vi "Text control 2 v7.3_pump-specific.vi"() -> ()   [LabVIEW 2019]
panel:
  in  "Tab Control":enum32{"Main", "Other parameters"}(tab)
  out "Vdg vs time (Bias Stress)":cluster{"Y data in":dbl[], "X data in":dbl[]}[](graph)
  out "Vp vs Vg (FPP)":cluster{"Y data in":dbl[], "X data in":dbl[]}[](graph)
  out "Vp vs time (FPP Bias Stress)":cluster{"Y data in":dbl[], "X data in":dbl[]}[](graph)
  out "Line running":i32
  out "Total lines":i32
  out "Path":path=path "C:/users/rlp38/09Apr2009LTtesting/test2.txt"
  out "I vs Vg":cluster{"Y data in":dbl[], "X data in":dbl[]}[](graph)
  out "Is max":dbl format="%.2e"
  out "Id max":dbl format="%.2e"
  out "Ig max":dbl format="%.2e"
  out "Imax vs time":cluster{"Y data in":dbl[], "X data in":dbl[]}[](graph)
  out "Imin vs time":cluster{"Y data in":dbl[], "X data in":dbl[]}[](graph)
  out "I vs Vd":cluster{"Y data in":dbl[], "X data in":dbl[]}[](graph)
  in  "Script":string
  out "Command running:":string
  out "Serial port data":string
  out "Elapsed Time":dbl caption="Elapsed Time (s)"
  in  "Time Units":u16(ring)=1 items=["Seconds", "Minutes", "Hours"]
  in  "Time Offset":dbl caption="Set Start Time (s)"
  in  "Reset":bool
  in  "Auto Reset":bool
  in  "integration time":u32(slide) max=2 step=1 scale=0.0..2.0
  in  "Interrupt scan":bool
  out "Absolute plunger position vs time":cluster{"Y data in":dbl[], "X data in":dbl[]}[](graph)
  out "Valve position vs time":cluster{"Y data in":dbl[], "X data in":dbl[]}[](graph)
  out "Is on":dbl format="%.2e"
  out "Id on":dbl format="%.2e"
  out "Ig on":dbl format="%.2e"
  out "Ion vs time":cluster{"Y data in":dbl[], "X data in":dbl[]}[](graph)
  out "Ioff vs time":cluster{"Y data in":dbl[], "X data in":dbl[]}[](graph)
  out "Ig min":dbl format="%.2e"
  out "Id min":dbl format="%.2e"
  out "Is min":dbl format="%.2e"
  out "Is off":dbl format="%.2e"
  out "Id off":dbl format="%.2e"
  out "Ig off":dbl format="%.2e"
  in  "Integration time (long)":dbl=0.32 min=0.04 max=2.0 step=0.02 format="%.2f"
  in  "Integration time (short)":dbl=0.0019 min=8e-05 max=0.0019 step=8e-05 format="%^.0e"
  in  "Gate: Compliance":dbl=0.001 format="%.8f"
  in  "Drain: Compliance":dbl=0.001 format="%.8f"
  in  "Hard stop pump":bool
  in  "Halt pump":bool
  in  "Interrupt program":bool
  in  "Suffix (script)":string="step_1_up-H2O_initial_script.txt"
  in  "Filename (variable part)":string="step_1_up-H2O_initial_"
  in  "Plot output curve extrema vs time":bool
  in  "Plot transfer curve extrema vs time":bool=TRUE
  in  "Plot sample extrema vs time":bool
  out "I vs time (Bias Stress)":cluster{"Y data in":dbl[], "X data in":dbl[]}[](graph)
  out "Vp1":dbl format="%.2e"
  out "Vp2":dbl format="%.2e"
  in  "Sample I - Probe 4 (Disabled)":u32(ring)=3 items=["SMU1  ", "SMU2  ", "SMU3  ", "SMU4  ", "SMU5  ", "SMU6  ", "VSU1  ", "VSU2  "]
  in  "Sample I - Source/Common":u32(ring) items=["SMU1  ", "SMU2  ", "SMU3  ", "SMU4  ", "SMU5  ", "SMU6  ", "VSU1  ", "VSU2  "]
  in  "Sample I - Probe 3 (Disabled)":u32(ring)=2 items=["SMU1  ", "SMU2  ", "SMU3  ", "SMU4  ", "SMU5  ", "SMU6  ", "VSU1  ", "VSU2  "]
  in  "Sample I - Drain/Gate":u32(ring)=1 items=["SMU1  ", "SMU2  ", "SMU3  ", "SMU4  ", "SMU5  ", "SMU6  ", "VSU1  ", "VSU2  "]
  in  "Sample - Probe 4":u32(ring)=3 items=["SMU1  ", "SMU2  ", "SMU3  ", "SMU4  ", "SMU5  ", "SMU6  ", "VSU1  ", "VSU2  "]
  in  "Sample - Source/Common":u32(ring) items=["SMU1  ", "SMU2  ", "SMU3  ", "SMU4  ", "SMU5  ", "SMU6  ", "VSU1  ", "VSU2  "]
  in  "Sample - Gate":u32(ring)=2 items=["SMU1  ", "SMU2  ", "SMU3  ", "SMU4  ", "SMU5  ", "SMU6  ", "VSU1  ", "VSU2  "]
  in  "Sample - Drain":u32(ring)=1 items=["SMU1  ", "SMU2  ", "SMU3  ", "SMU4  ", "SMU5  ", "SMU6  ", "VSU1  ", "VSU2  "]
  in  "VSU2 Stress - Source/Common":u32(ring) items=["SMU1  ", "SMU2  ", "SMU3  ", "SMU4  ", "SMU5  ", "SMU6  ", "VSU1  "]
  in  "Stress I - Source/Common":u32(ring) items=["SMU1  ", "SMU2  ", "SMU3  ", "SMU4  ", "SMU5  ", "SMU6  ", "VSU1  ", "VSU2  "]
  in  "Stress I - Drain/Gate":u32(ring)=1 items=["SMU1  ", "SMU2  ", "SMU3  ", "SMU4  ", "SMU5  ", "SMU6  ", "VSU1  ", "VSU2  "]
  in  "Stress V - Source/Common":u32(ring) items=["SMU1  ", "SMU2  ", "SMU3  ", "SMU4  ", "SMU5  ", "SMU6  ", "VSU1  ", "VSU2  "]
  in  "Stress V - Gate":u32(ring)=2 items=["SMU1  ", "SMU2  ", "SMU3  ", "SMU4  ", "SMU5  ", "SMU6  ", "VSU1  ", "VSU2  "]
  in  "Stress V - Drain":u32(ring)=1 items=["SMU1  ", "SMU2  ", "SMU3  ", "SMU4  ", "SMU5  ", "SMU6  ", "VSU1  ", "VSU2  "]
  in  "FPP - Source":u32(ring)=6 items=["SMU1  ", "SMU2  ", "SMU3  ", "SMU4  ", "SMU5  ", "SMU6  ", "VSU1  ", "VSU2  "]
  in  "FPP - Probe 2":u32(ring)=3 items=["SMU1  ", "SMU2  ", "SMU3  ", "SMU4  ", "SMU5  ", "SMU6  ", "VSU1  ", "VSU2  "]
  in  "FPP - Probe 1":u32(ring) items=["SMU1  ", "SMU2  ", "SMU3  ", "SMU4  ", "SMU5  ", "SMU6  ", "VSU1  ", "VSU2  "]
  in  "FPP - Gate":u32(ring)=2 items=["SMU1  ", "SMU2  ", "SMU3  ", "SMU4  ", "SMU5  ", "SMU6  ", "VSU1  ", "VSU2  "]
  in  "FPP - Drain":u32(ring)=1 items=["SMU1  ", "SMU2  ", "SMU3  ", "SMU4  ", "SMU5  ", "SMU6  ", "VSU1  ", "VSU2  "]
  in  "Pulsed Stress V - Vextra":u32(ring)=6 items=["SMU1  ", "SMU2  ", "SMU3  ", "SMU4  ", "SMU5  ", "SMU6  ", "VSU1  ", "VSU2  "]
  in  "Pulsed Stress V - Probe 4":u32(ring)=3 items=["SMU1  ", "SMU2  ", "SMU3  ", "SMU4  ", "SMU5  ", "SMU6  ", "VSU1  ", "VSU2  "]
  in  "Pulsed Stress V - Source/Common":u32(ring) items=["SMU1  ", "SMU2  ", "SMU3  ", "SMU4  ", "SMU5  ", "SMU6  ", "VSU1  ", "VSU2  "]
  in  "Pulsed Stress V - Gate":u32(ring)=2 items=["SMU1  ", "SMU2  ", "SMU3  ", "SMU4  ", "SMU5  ", "SMU6  ", "VSU1  ", "VSU2  "]
  in  "Pulsed Stress V - Drain":u32(ring)=1 items=["SMU1  ", "SMU2  ", "SMU3  ", "SMU4  ", "SMU5  ", "SMU6  ", "VSU1  ", "VSU2  "]
  in  "Transfer/Output - Probe 4":u32(ring)=3 items=["SMU1  ", "SMU2  ", "SMU3  ", "SMU4  ", "SMU5  ", "SMU6  ", "VSU1  ", "VSU2  "]
  in  "Transfer/Output - Source/Common":u32(ring) items=["SMU1  ", "SMU2  ", "SMU3  ", "SMU4  ", "SMU5  ", "SMU6  ", "VSU1  ", "VSU2  "]
  in  "Transfer/Output - Gate":u32(ring)=2 items=["SMU1  ", "SMU2  ", "SMU3  ", "SMU4  ", "SMU5  ", "SMU6  ", "VSU1  ", "VSU2  "]
  in  "Transfer/Output - Drain":u32(ring)=1 items=["SMU1  ", "SMU2  ", "SMU3  ", "SMU4  ", "SMU5  ", "SMU6  ", "VSU1  ", "VSU2  "]
  in  "Gate Range\nmode":u16(ring) items=["Auto", "Limited", "Fixed"]
  in  "Gate Range":u8(slide)=3 max=11 scale=0.0..11.0
  in  "Source/Drain\nRange mode":u16(ring) items=["Auto", "Limited", "Fixed"]
  in  "Source/Drain Range":u8(slide)=3 max=11 scale=0.0..11.0
  in  "Panel Controls":T1={"Emergency Stop"=refnum, "TransGraph Max"=1e-05, "Text/Graph (text=false)"=TRUE} {"TransGraph Max" format="%.2e"}
  in  "Panel Controls 2":T2={"Emergency Stop"=refnum, "TransGraph Max"=1e-05, "Text/Graph (text=false)"=TRUE, "TransGraph Min"=1e-11} {"TransGraph Min" format="%.2e"; "TransGraph Max" format="%.2e"}
  in  "Probe 4":cluster{"on/off":bool, "Voltage":dbl} {"Voltage" min=-100.0 max=100.0 format="%.2f"}
  in  "Full Reset":bool
  in  "Standby":T3
  out "error out":errorcluster
  in  "Delay before read (ms)":u32=1000
  in  "byte count":u32=64
  in  "Serial End Mode for Reads":u16(ring)=2 items=["None", "LastBit", "TermChar"]
  in  "Timeout (ms)":u32=10000
  in  "Enable Termination\nChar (T)":bool=TRUE
  in  "Termination char\n(0xA = '\\n' = LF)\n(0xD = '\\r' = CR)":u8=13 format="%.0x"
  in  "flow control":u16(ring) items=["None"=0, "XON/XOFF"=1, "RTS/CTS"=2, "DTR/DSR"=4]
  in  "stop bits":u16(ring)=10 items=["1.0"=10, "1.5"=15, "2.0"=20]
  in  "parity":u16(ring) items=["None", "Odd", "Even", "Mark", "Space"]
  in  "data bits":u16=8 min=5 max=8 step=1
  in  "VISA resource name":refnum<visa-resource-name>="COM6"
  in  "baud rate":u32=9600
  out "Timings Indicator":T4 {"integration time" scale=0.0..2.0}
  in  "Timings (overwritten by the Front Panel)":T5={"integration time"=0, "Short/Long integration time"=0.00064, "hold time (sec)"=0.0, "delay time (sec)"=0.0, "Step Time (0 disables)"=0.0, "sweep method"=0, "Pulse period"=0.005, "Base voltage"=0.0, "Pulse width"=0.0005} {"Pulse width" min=0.0005 max=0.1 step=0.0001 format="%.4f"; "Base voltage" format="%^.4e"; "Pulse period" min=0.005 max=1.0 step=0.0001 format="%.4f"; "sweep method" items=["Continuous", "Pulsed"]; "Step Time (0 disables)" format="%.2f"; "delay time (sec)" format="%.4f"; "hold time (sec)" format="%.4f"; "Short/Long integration time" format="%^.0e"; "integration time" scale=0.0..2.0}
  out "Probe 4 Indicator":cluster{"on/off":bool, "Voltage":dbl} {"Voltage" min=-100.0 max=100.0 format="%.2f"}
  in  "VISA resource name in":refnum<visa-resource-name>="GPIB0::14::INSTR"
  in  "Gate":T6={"Gate Start"=0.0, "Gate Stop"=2.0, "Gate Step (linear only)"=1.0, "Gate Compliance"=0.0001, "Gate PComp"=0.0, "Range mode"=0, "Range"=6} {"Range" max=11 scale=0.0..11.0; "Range mode" items=["Auto", "Limited", "Fixed"]; "Gate PComp" format="%^.2e"; "Gate Compliance" format="%^.2e"; "Gate Step (linear only)" format="%^.4e"; "Gate Stop" format="%^.4e"; "Gate Start" format="%^.4e"}
  in  "Drain 2":T7={"Drain Start"=0.0, "Drain Stop"=2.0, "Drain Compliance"=0.0001, "Drain Step"=1.0, "Drain PComp"=0.0, "Range mode"=0, "Range"=6} {"Range" max=11 scale=0.0..11.0; "Range mode" items=["Auto", "Limited", "Fixed"]; "Drain PComp" format="%^.2e"; "Drain Step" format="%^.4e"; "Drain Compliance" format="%^.2e"; "Drain Stop" format="%^.4e"; "Drain Start" format="%^.4e"}
  # "Syntax:\nitime [s|m|l] time(sec): [s|m|l] determines the integration time setting (small|medium|long) and time sets the value.\nNOTE: The value of the integration time has to be within the range allowed by its category (s|m|l), otherwise, the closest value will be used. (e.g. if the category is set to short but the time value is very long, the actual value used will be the maximum short integration time.\nIntegration times:\n    Short: Default: 640 us. Range: 8E-5 - 1.92E-3 seconds.\n    Medium: Fixed at 1 NPL cycle (0.02 seconds).\n    Long: Default: 16 NPL cycles (0.32 seconds). Range: 2-100 NPL cycles (0.04 seconds - 2 seconds).\ngaterangemode [a|l|f]\ndrainrangemode [a|l|f]\npulsed [on|off] PulsePeriod(sec) PulseBaseVoltage PulseONWidth(sec)\nstandby [on l off]\nwait NumMilliseconds\nwait-min NumMinutes\n# texthere = comment\nProbe4 [ON|OFF] Voltage\ntransfer [s|d] VgStart VgStop VgStep VdStart VdStop VdStep\noutput [s|d] VgStart VgStop VgStep VdStart VdStop VdStep\nsample Vg Vd NumSamples Time(s) SampleInterval(s)\nsamplei Idg NumSamples Time(s) SampleInterval(s) VDGcompliance\n100 samples is approximately 13 seconds with medium integration\n# If in doubt use SampleInterval(s) = 0.004\n    NOTE: When doing bias stress measurements, it is best to set the Time Units to \"Seconds\", as the \"sample\" command has been configured to give the output to seconds.\nstressV VG VD IGcompliance IDcompliance Duration(sec)\nstressI IDG VDGcompliance Duration(sec)\nvsu2pulse Bias Duration(s)\npulsedstressV [s|d] VEstop VgON VgOFF Period(s) PulseONwidth(s) Vd\nsample-fpp Vg Vd NumSamples Time\nresample-fpp Vg Vd\ntransfer-fpp [s|d] VgStart VgStop VgStep VdStart VdStop VdStep\noutput-fpp [s|d] VgStart VgStop VgStep VdStart VdStop VdStep\nserial SerialPortCommand\npump SerialPortCommand for the SPM pump\n\nSPM Pump Syntax (<x>: pump number, use 1 if only one pump):\nif the command syntax contains [R], then append the letter R to the command\n/<x>Q: query (a query command should follow each command)\n/<x>Z[R] or /<x>Y[R]: initialize pump\n/<x>N<n>[R] (<n>=0,1): <0> (<1>) microstep 0.01 mm (0.00125 mm) resolution\n/<x>I<n> (<n>=0-6): turn to port number n (clockwise)\n/<x>O<n> (<n>=0-6): turn to port number n (counterclockwise)\n/<x>X: Re-execute last command string\n/<x>G<n>[R] (<n>=0-60000): repeat command sequence (default: 0, 0=loop forever)\n/<x>g: Mark the start of a repeat sequence (max = 10)\n/<x>M<n>[R] (<n>=0-86400000): delay command execution by n milliseconds\n/<x>H: Halt; Pause the sequence after finishing the current move\n/<x>T: Hardstop; Interrupt the current move and suppress it from the sequence\n/<x>A<n>[R] (<n>=0-3000 with N=0, 0-24000 with N=1): absolute position\n/<x>P<n>[R] (<n>=0-3000 with N=0, 0-24000 with N=1): relative pickup\n/<x>D<n>[R] (<n>=0-3000 with N=0, 0-24000 with N=1): relative dispense\n/<x>V<n>[R] (<n>=1-1600 default: 150): set peak speed (pulses/sec)\nNOTE: The lowest speed limit is 1 pulse/sec, not 5, as the manual states.\n/<x>S<n>[R] (<n>=10-40 default: 22): set speed (NOT in pulses/sec, look in manual)\nNOTE: When controlled with absolute position, one does not need to pay special attention to the syringe that is mounted on the pump.\nWithdraw from lower stage (ports 3, 5), dispense from higher stage (ports 2, 4, 6).\nConnect Port 1 to waste."
  # "Time"
  # "1\n2\n3\n4\n5\n6\n7\n8\n9\n10\n11\n12\n13\n14\n15\n16\n17\n18\n19\n20"
  # "Serial port settings"
  # "SMUs"
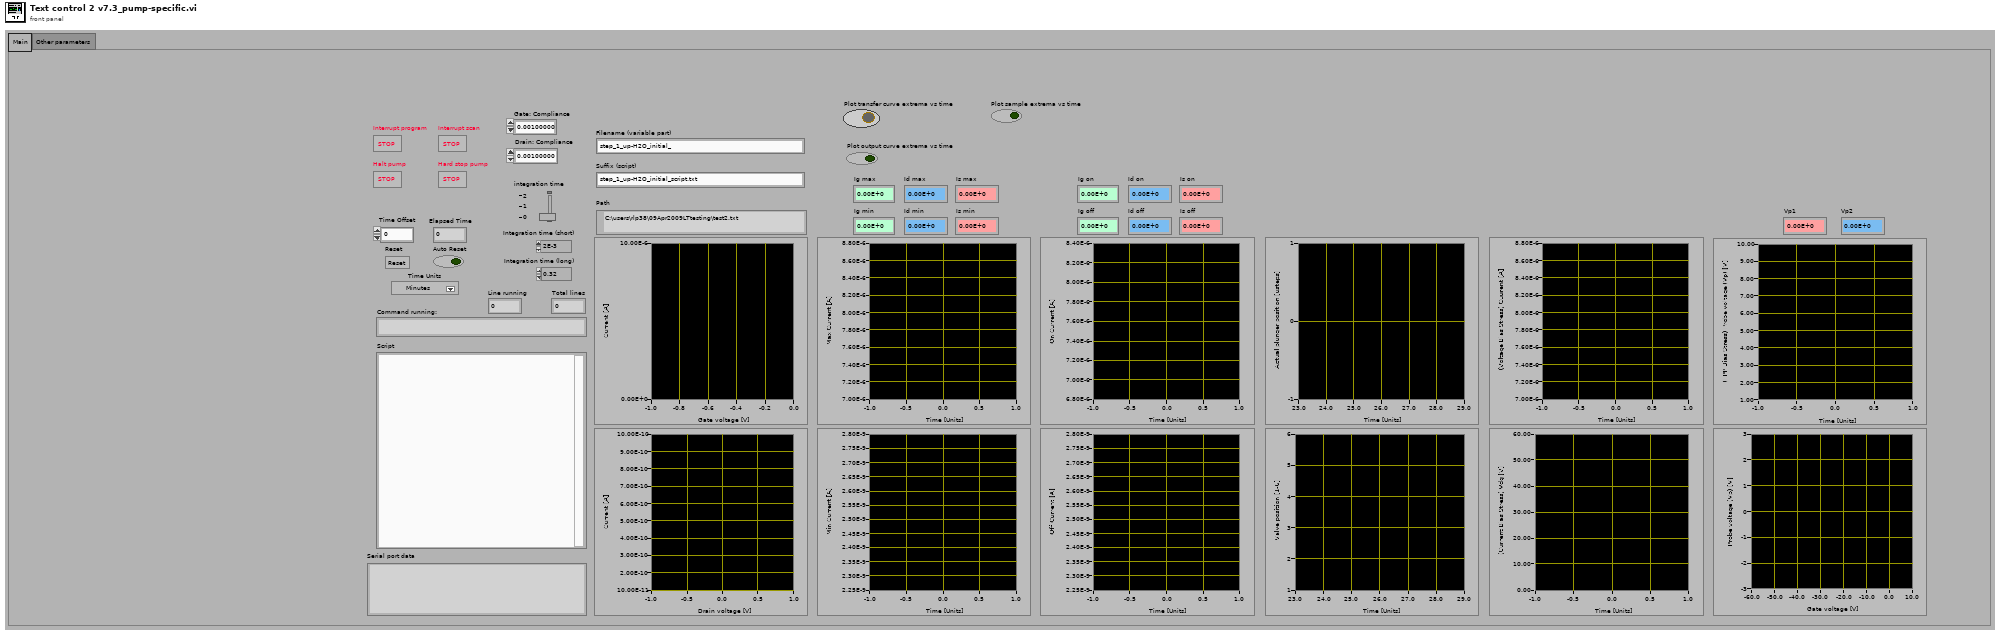
[diagram p1: front panel]
types:
  T1 = cluster{"Emergency Stop":refnum<vi>, "TransGraph Max":dbl, "Text/Graph (text=false)":bool}
  T2 = cluster{"Emergency Stop":refnum<vi>, "TransGraph Max":dbl, "Text/Graph (text=false)":bool, "TransGraph Min":dbl}
  T3 = cluster{"Gate Standby":bool, "Drain Standby":bool}
  T4 = cluster{"Short/Long integration time":dbl, "hold time (sec)":dbl, "delay time (sec)":dbl, "Step Time (0 disables)":dbl, "sweep method":u16, "Pulse period":dbl, "Base voltage":dbl, "Pulse width":dbl, "integration time":u32}
  T5 = cluster{"integration time":u32, "Short/Long integration time":dbl, "hold time (sec)":dbl, "delay time (sec)":dbl, "Step Time (0 disables)":dbl, "sweep method":u16, "Pulse period":dbl, "Base voltage":dbl, "Pulse width":dbl}
  T6 = cluster{"Gate Start":dbl, "Gate Stop":dbl, "Gate Step (linear only)":dbl, "Gate Compliance":dbl, "Gate PComp":dbl, "Range mode":u16, "Range":u8}
  T7 = cluster{"Drain Start":dbl, "Drain Stop":dbl, "Drain Compliance":dbl, "Drain Step":dbl, "Drain PComp":dbl, "Range mode":u16, "Range":u8}
  T8 = enum16{"open", "replace", "create", "open or create", "replace or create", "replace or create with confirmation"}
  T9 = cluster{"V2 Start":dbl, "V2 Step":dbl, "Number of points":i32}
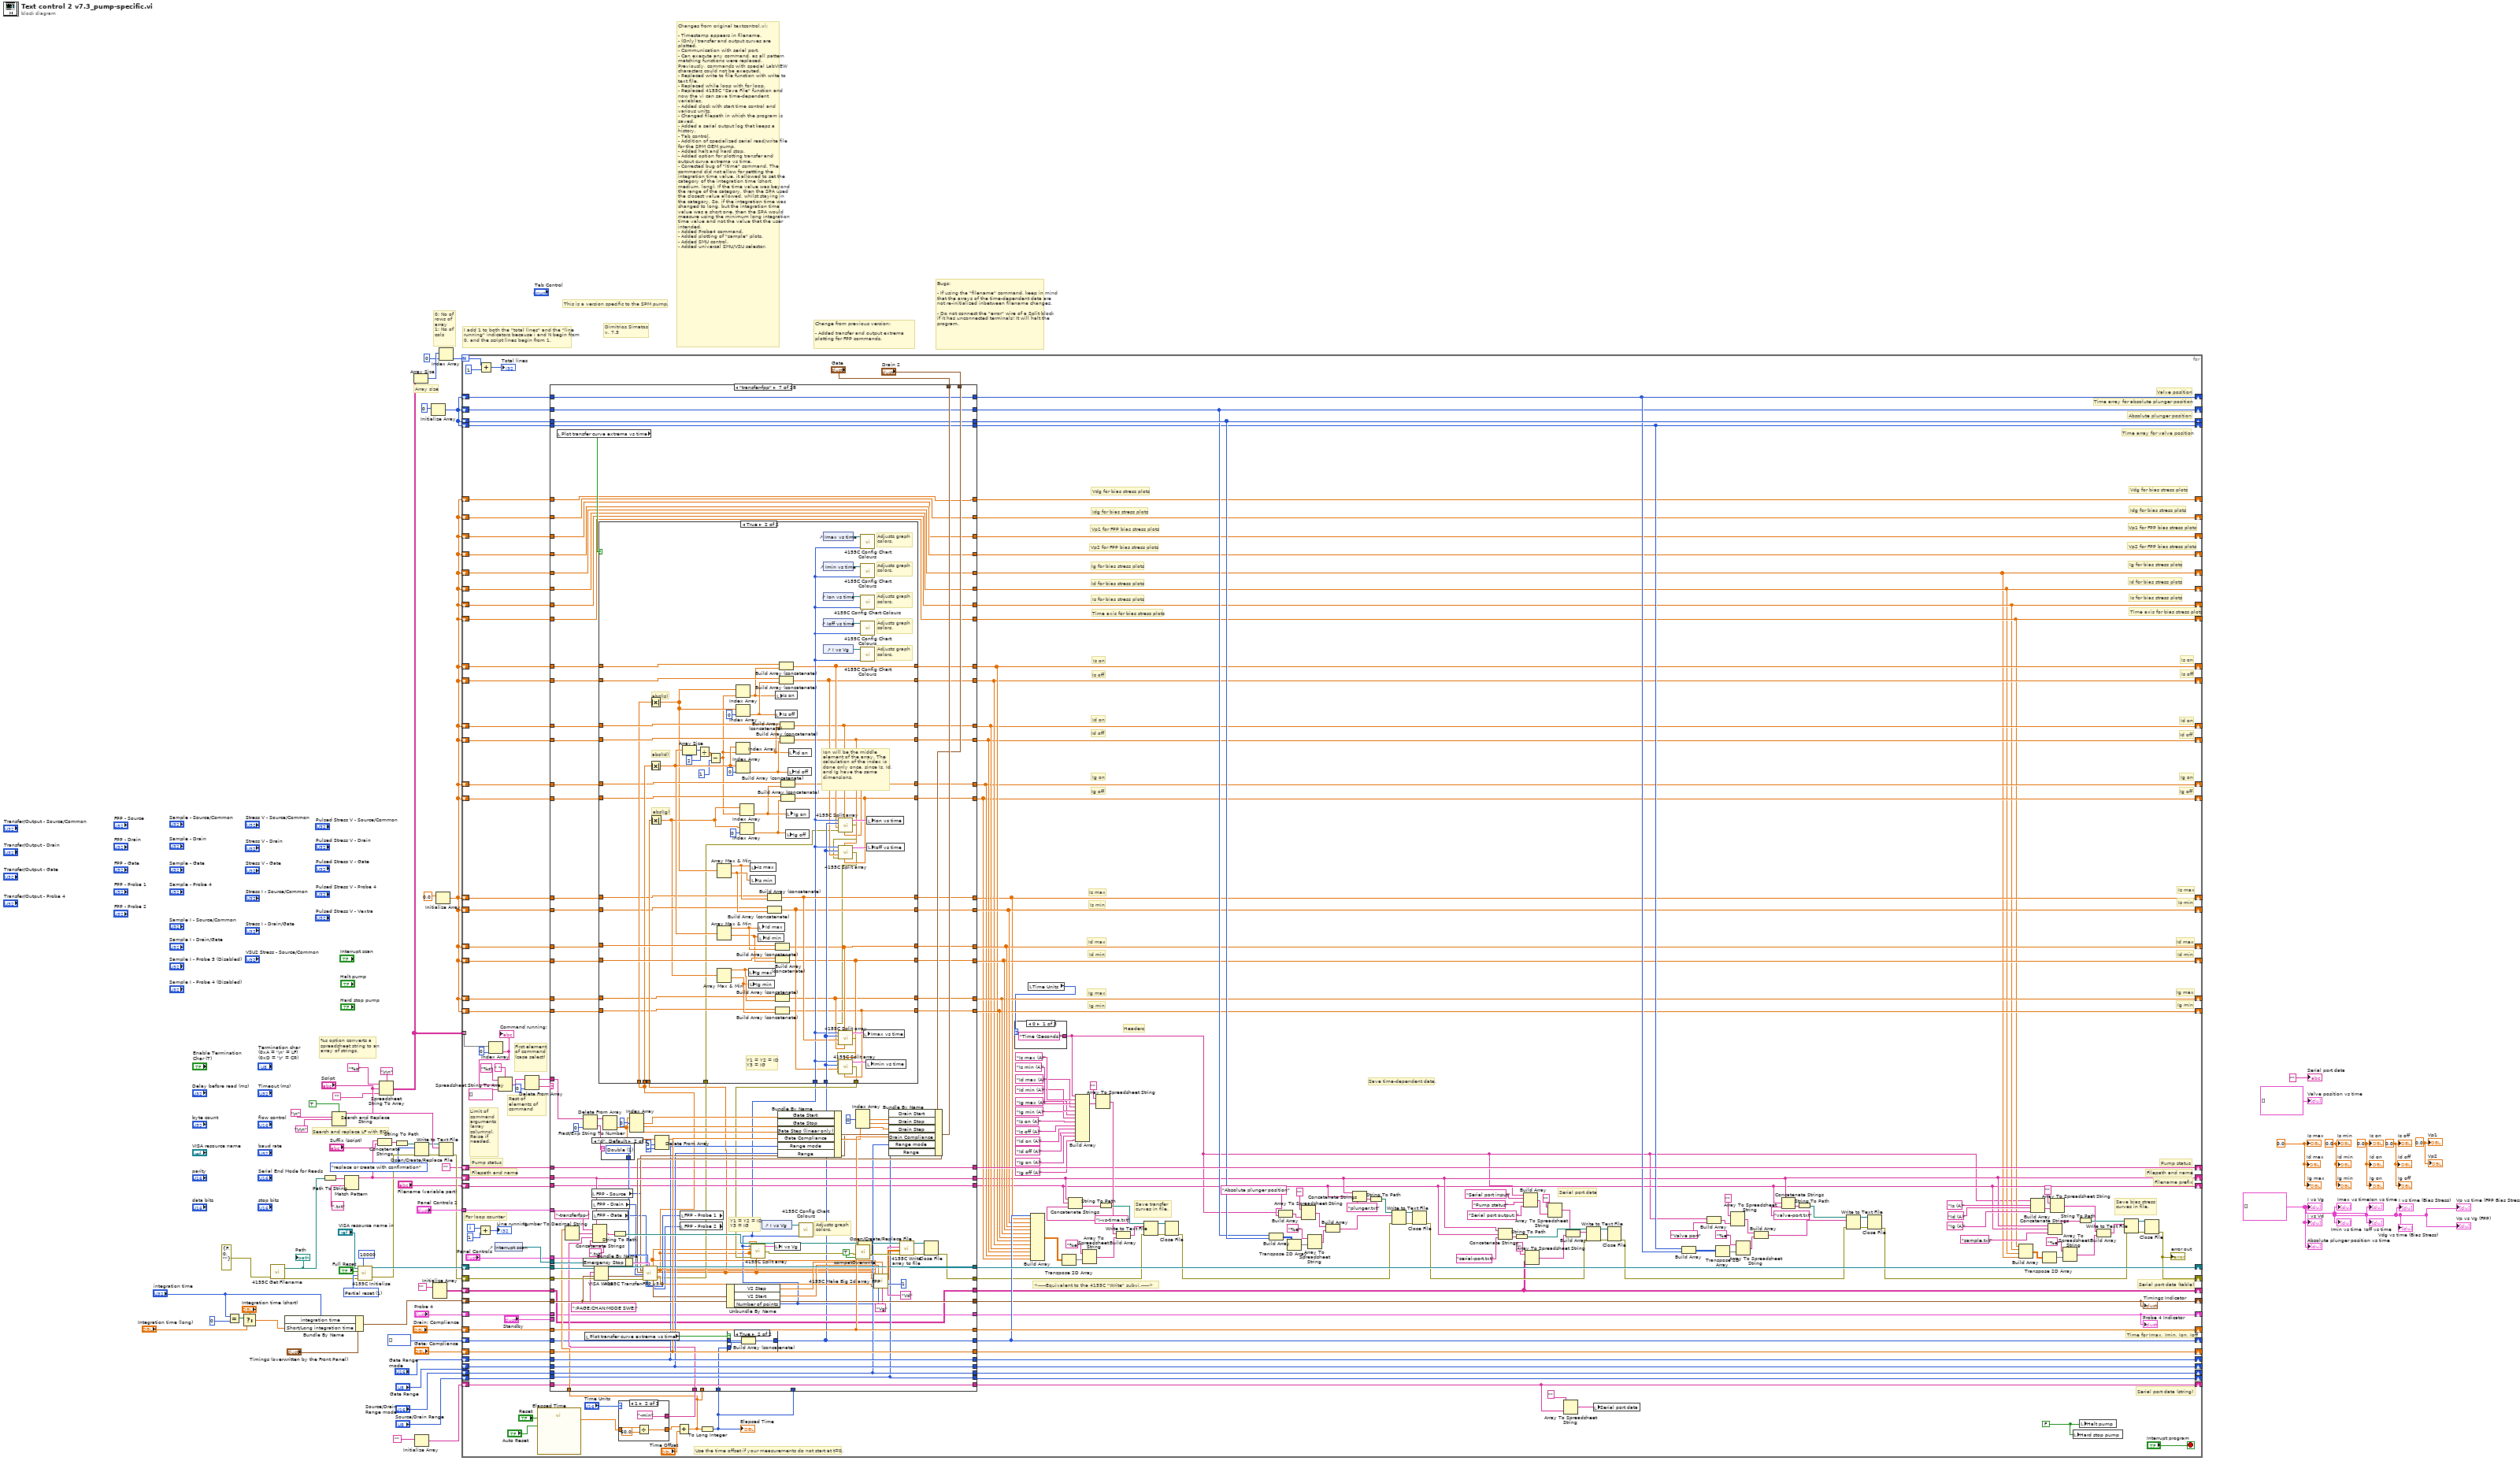
[diagram p0: block diagram]
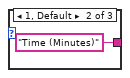
[diagram p2: hidden frame]
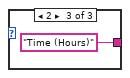
[diagram p3: hidden frame]
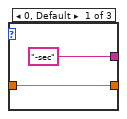
[diagram p4: hidden frame]
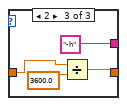
[diagram p5: hidden frame]
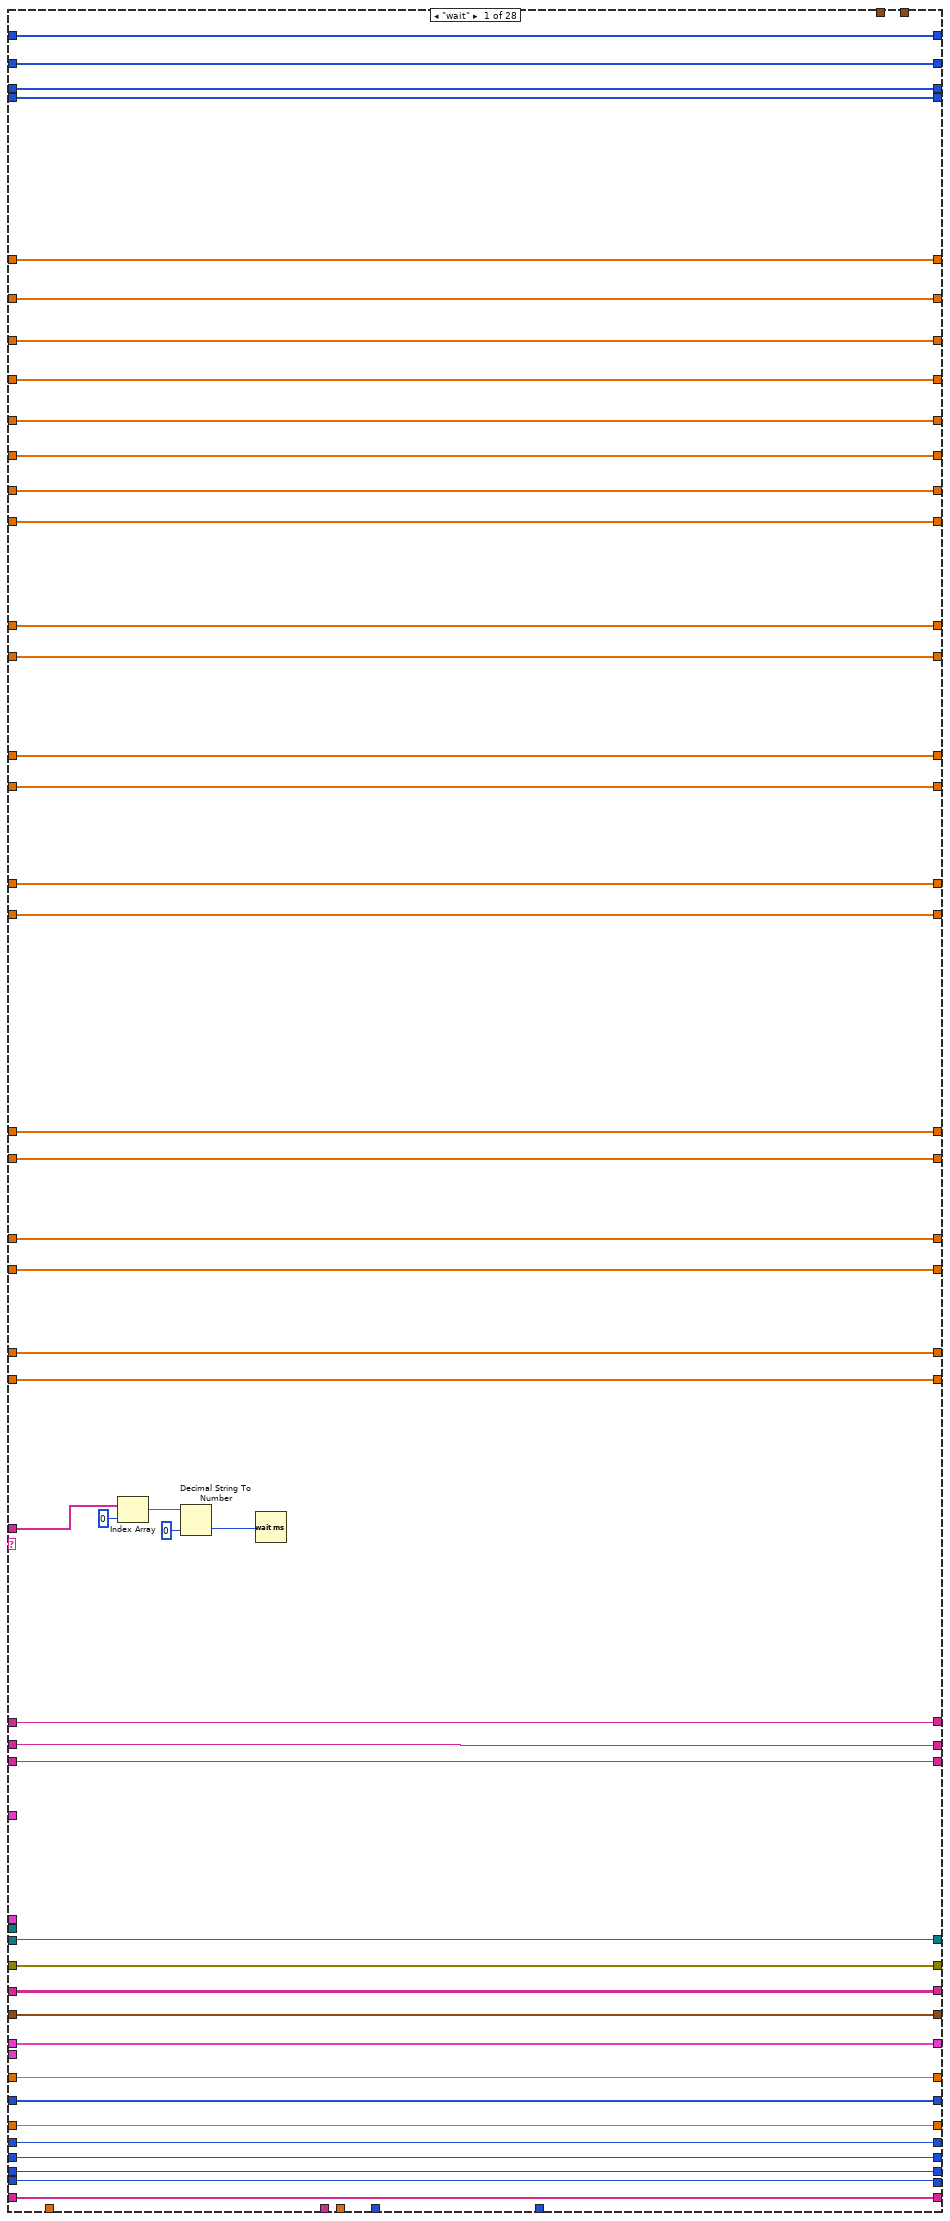
[diagram p6: hidden frame]
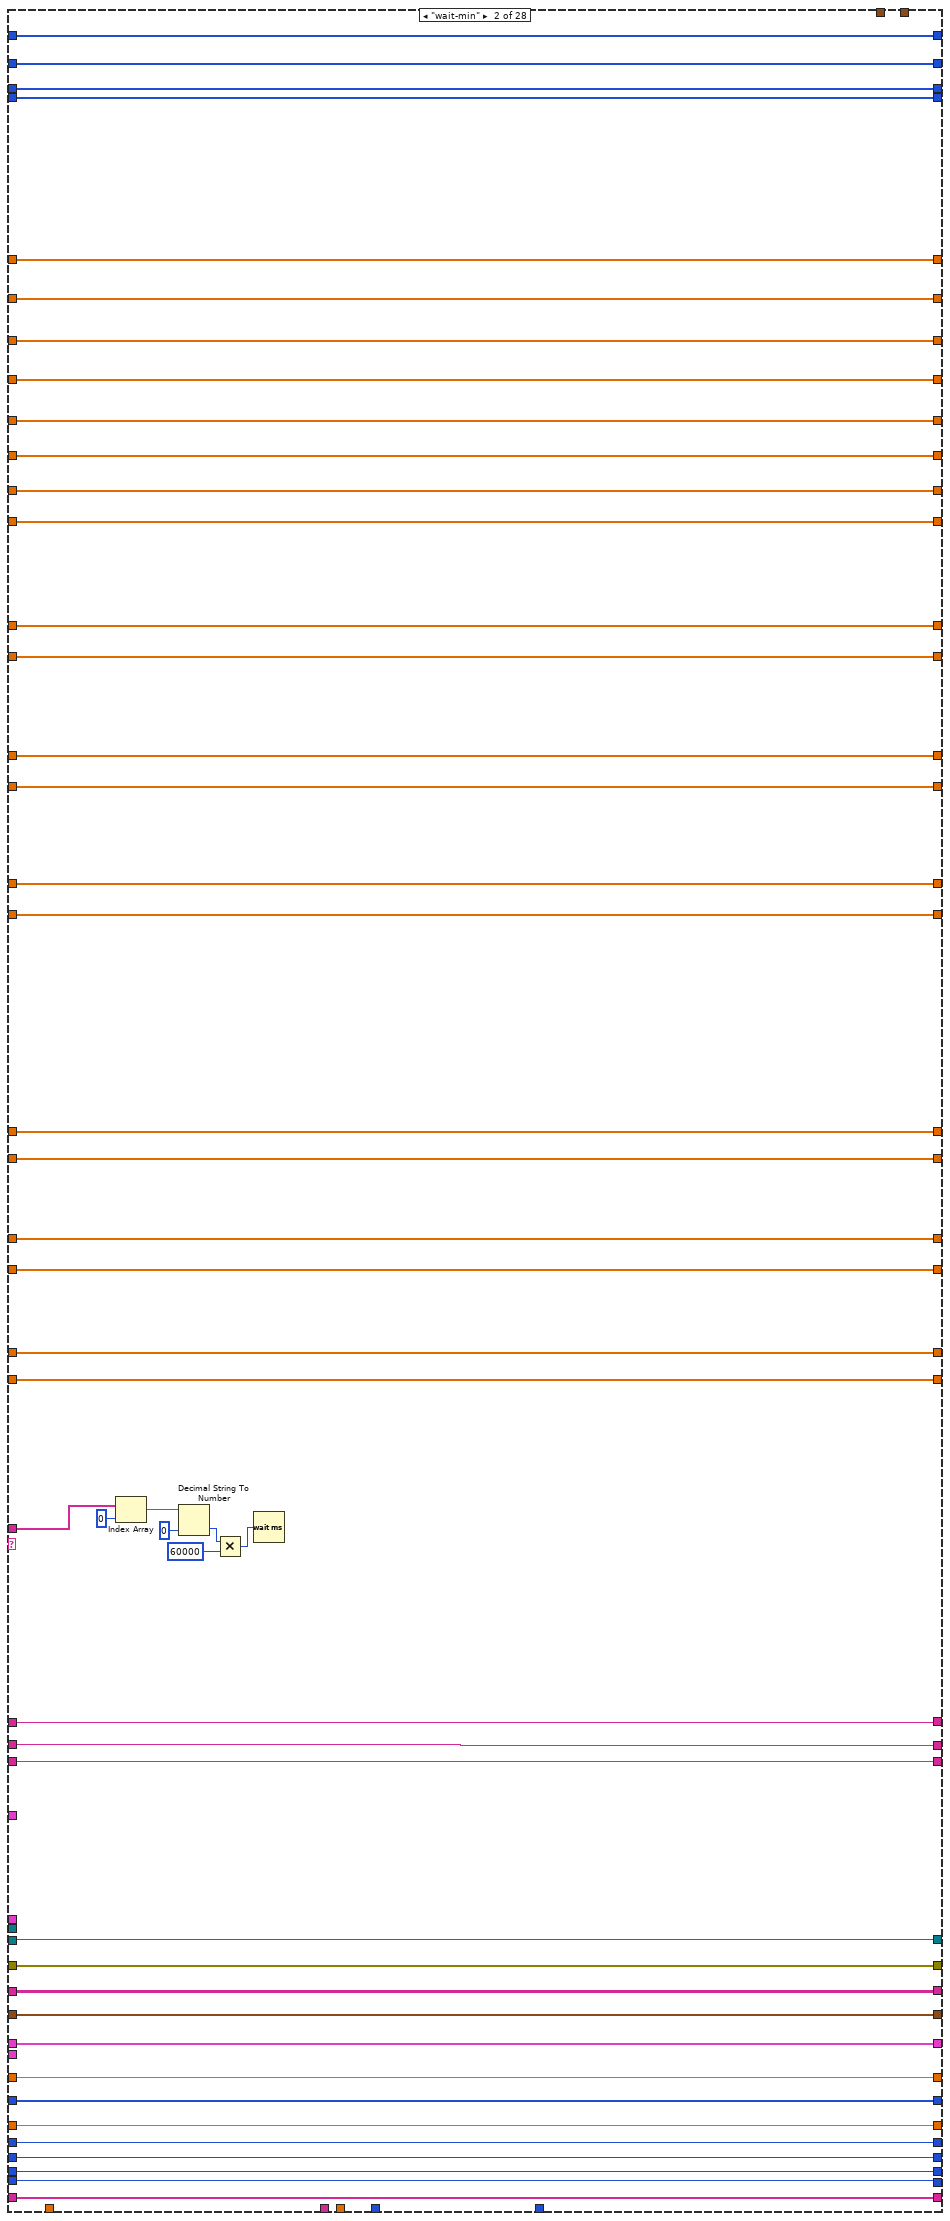
[diagram p7: hidden frame]
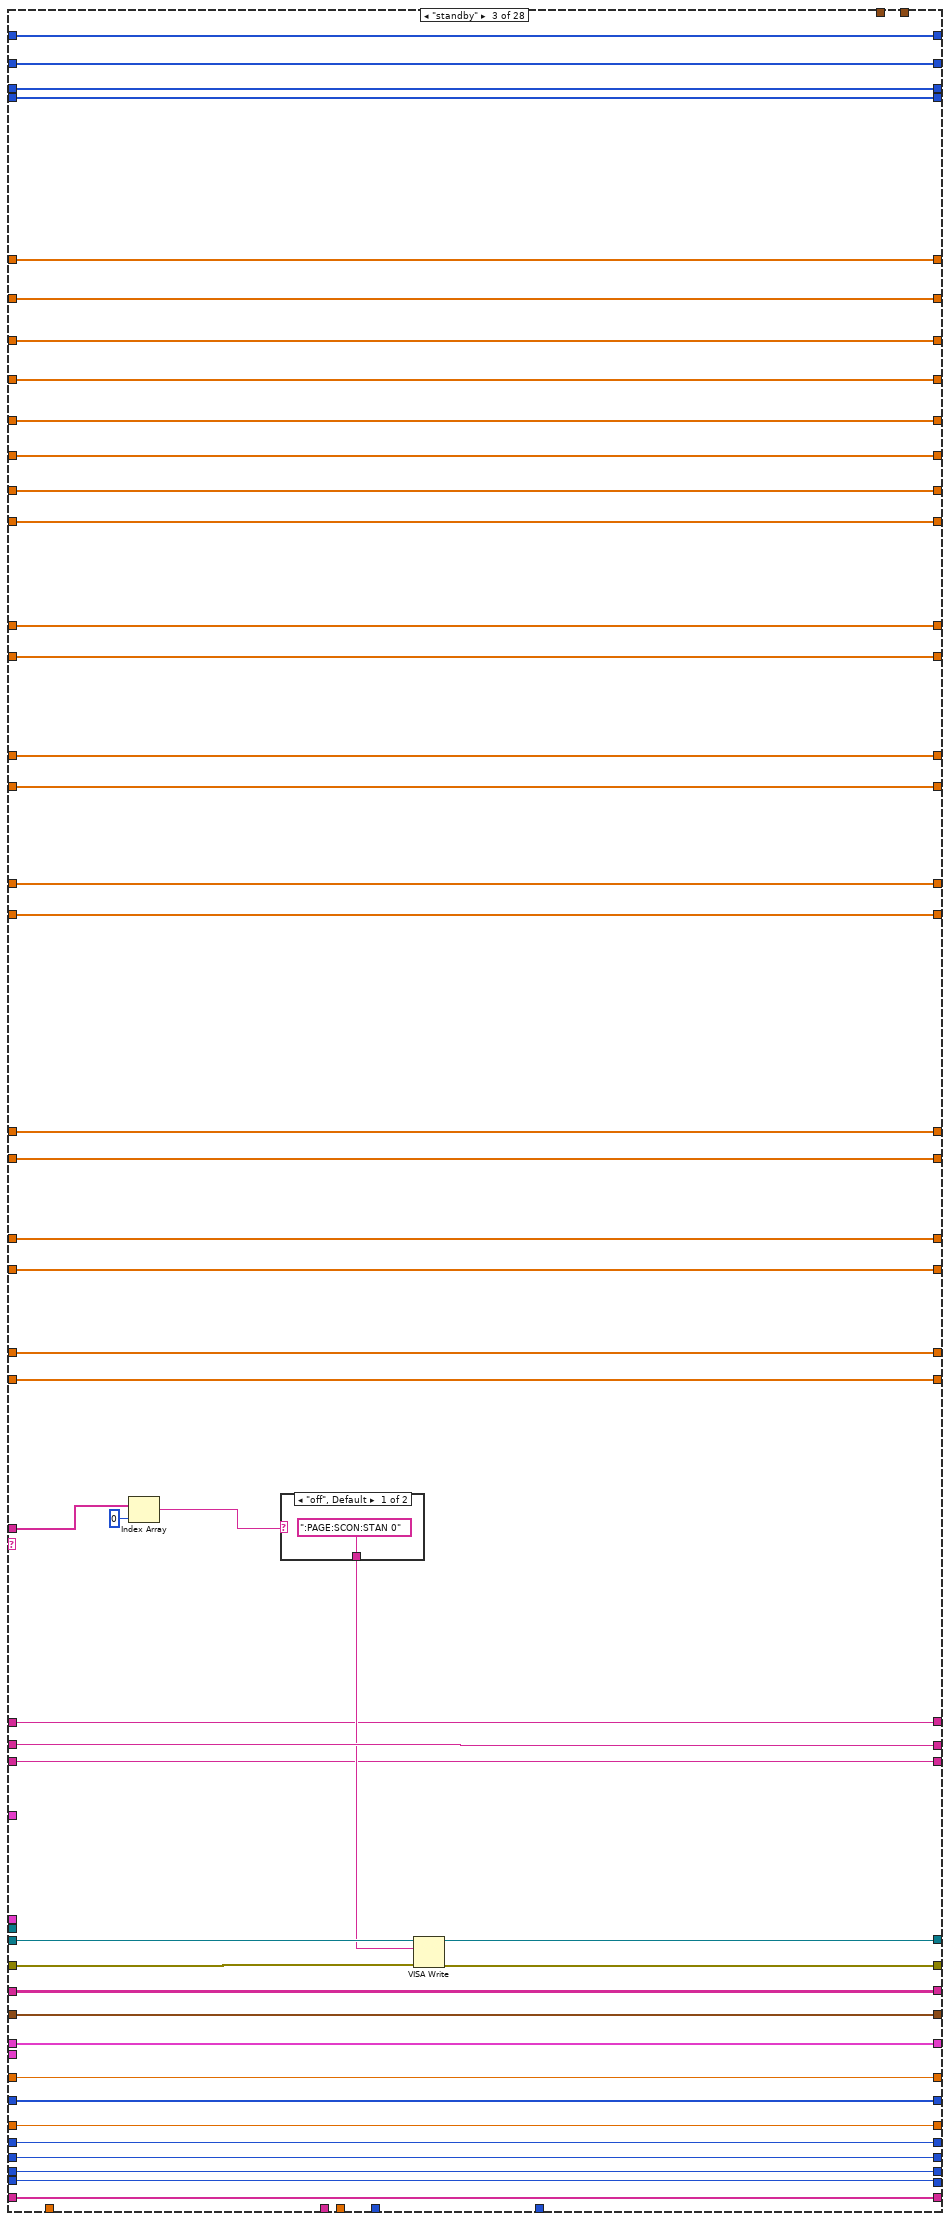
[diagram p8: hidden frame]
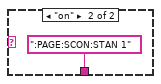
[diagram p9: hidden frame]
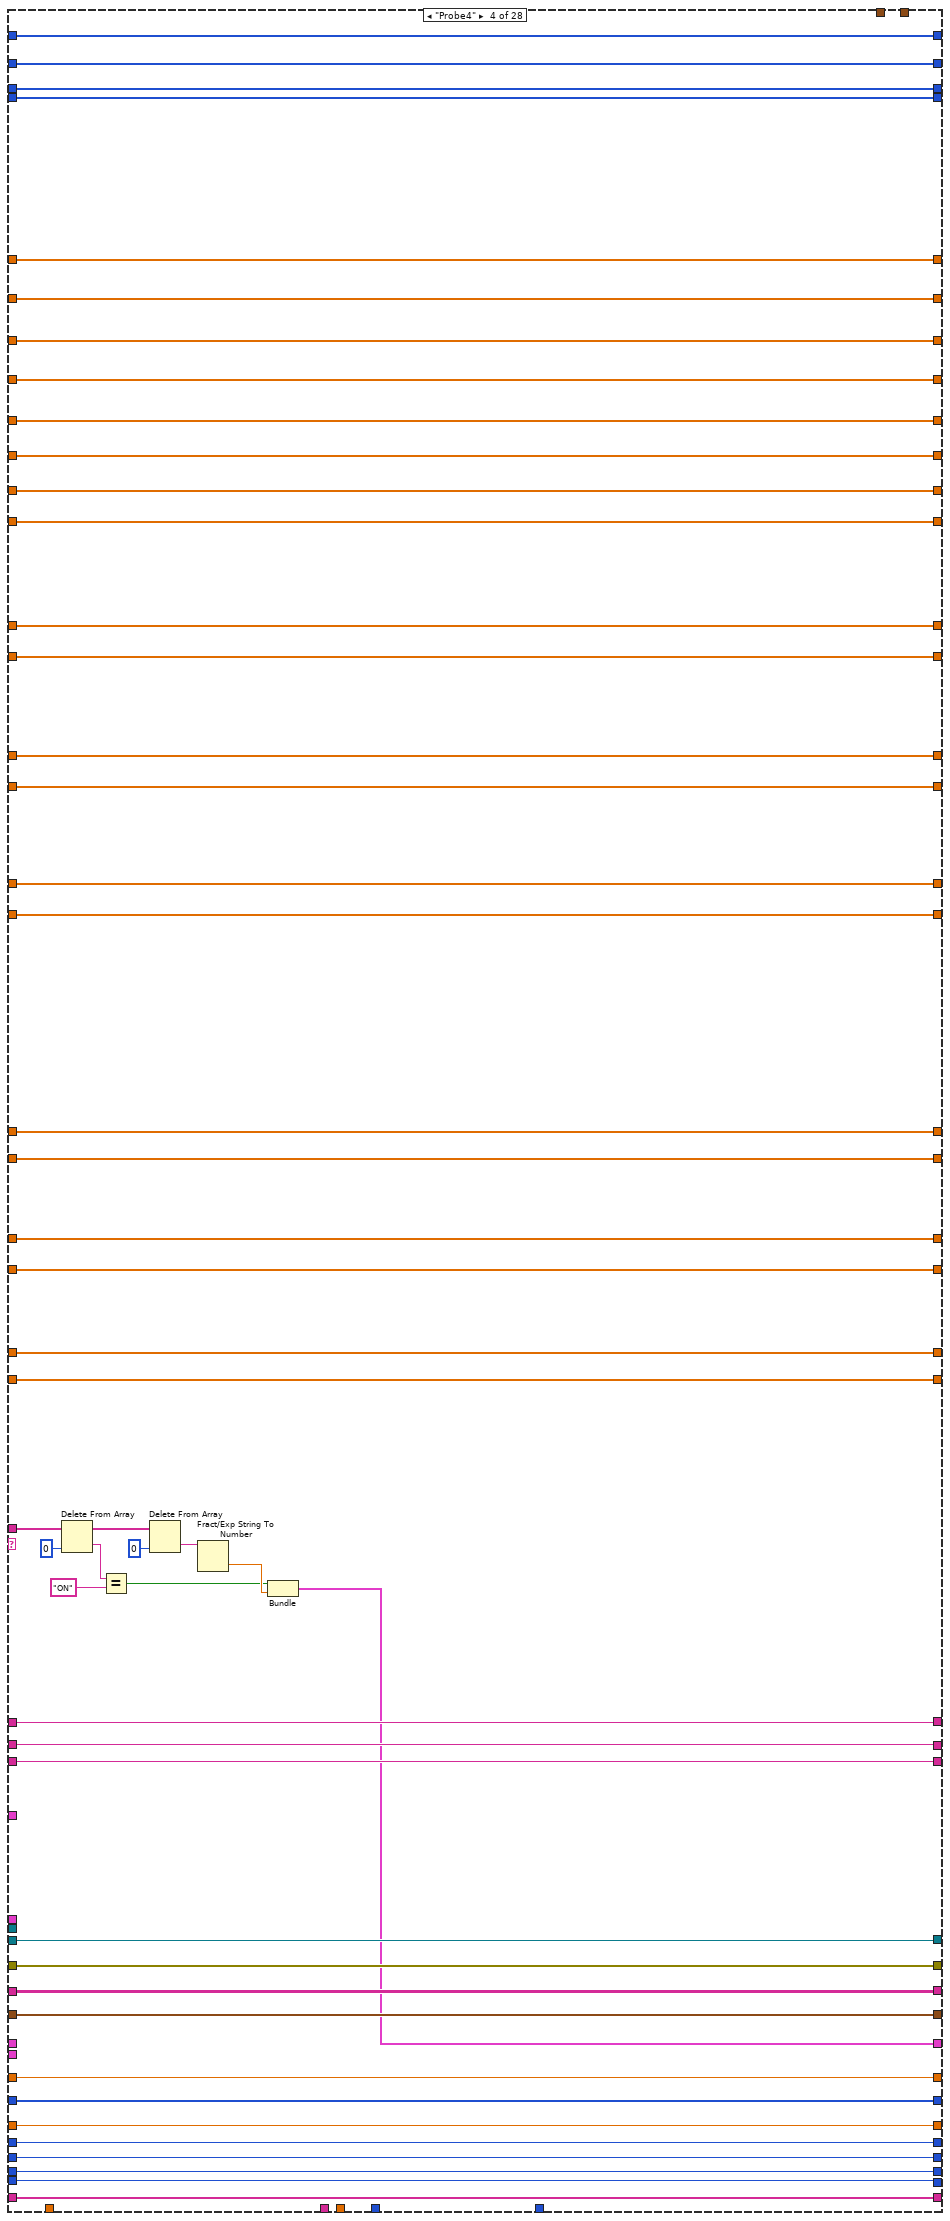
[diagram p10: hidden frame]
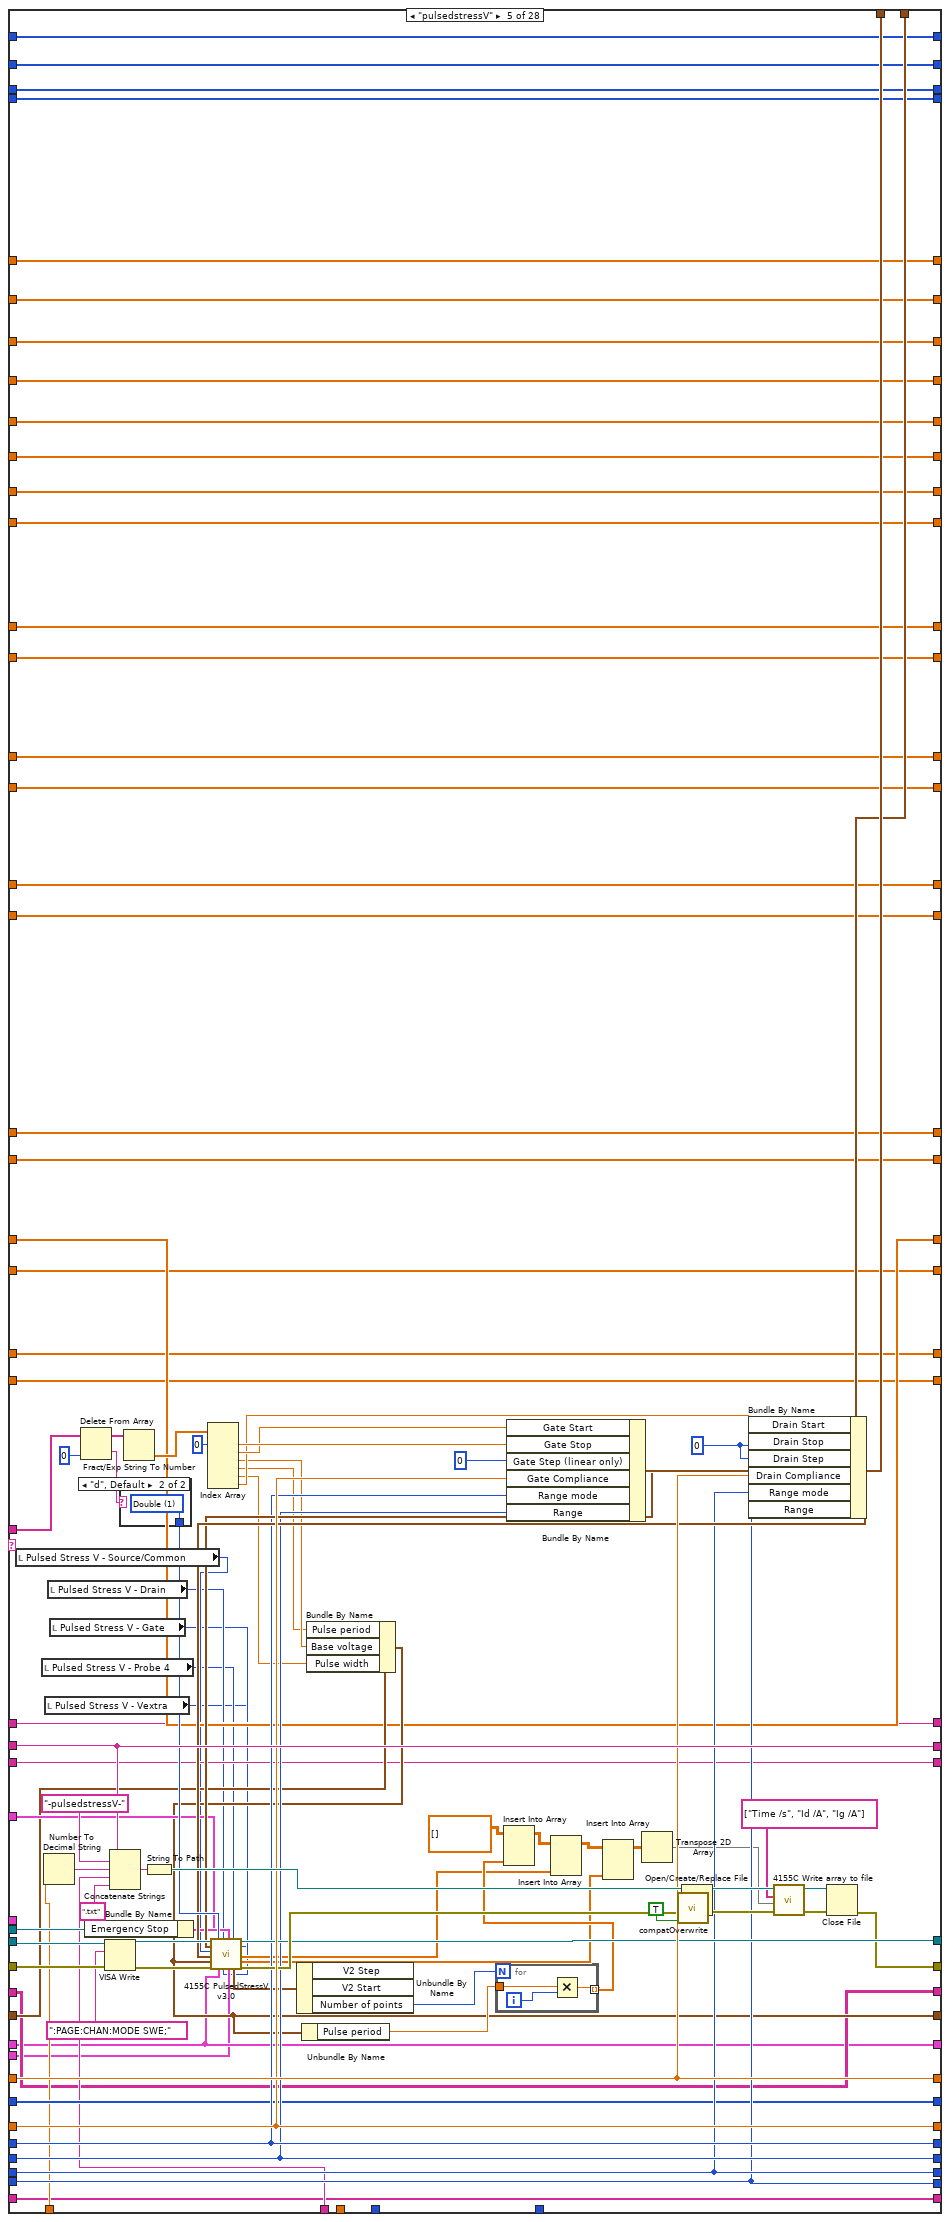
[diagram p11: hidden frame]
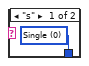
[diagram p12: hidden frame]
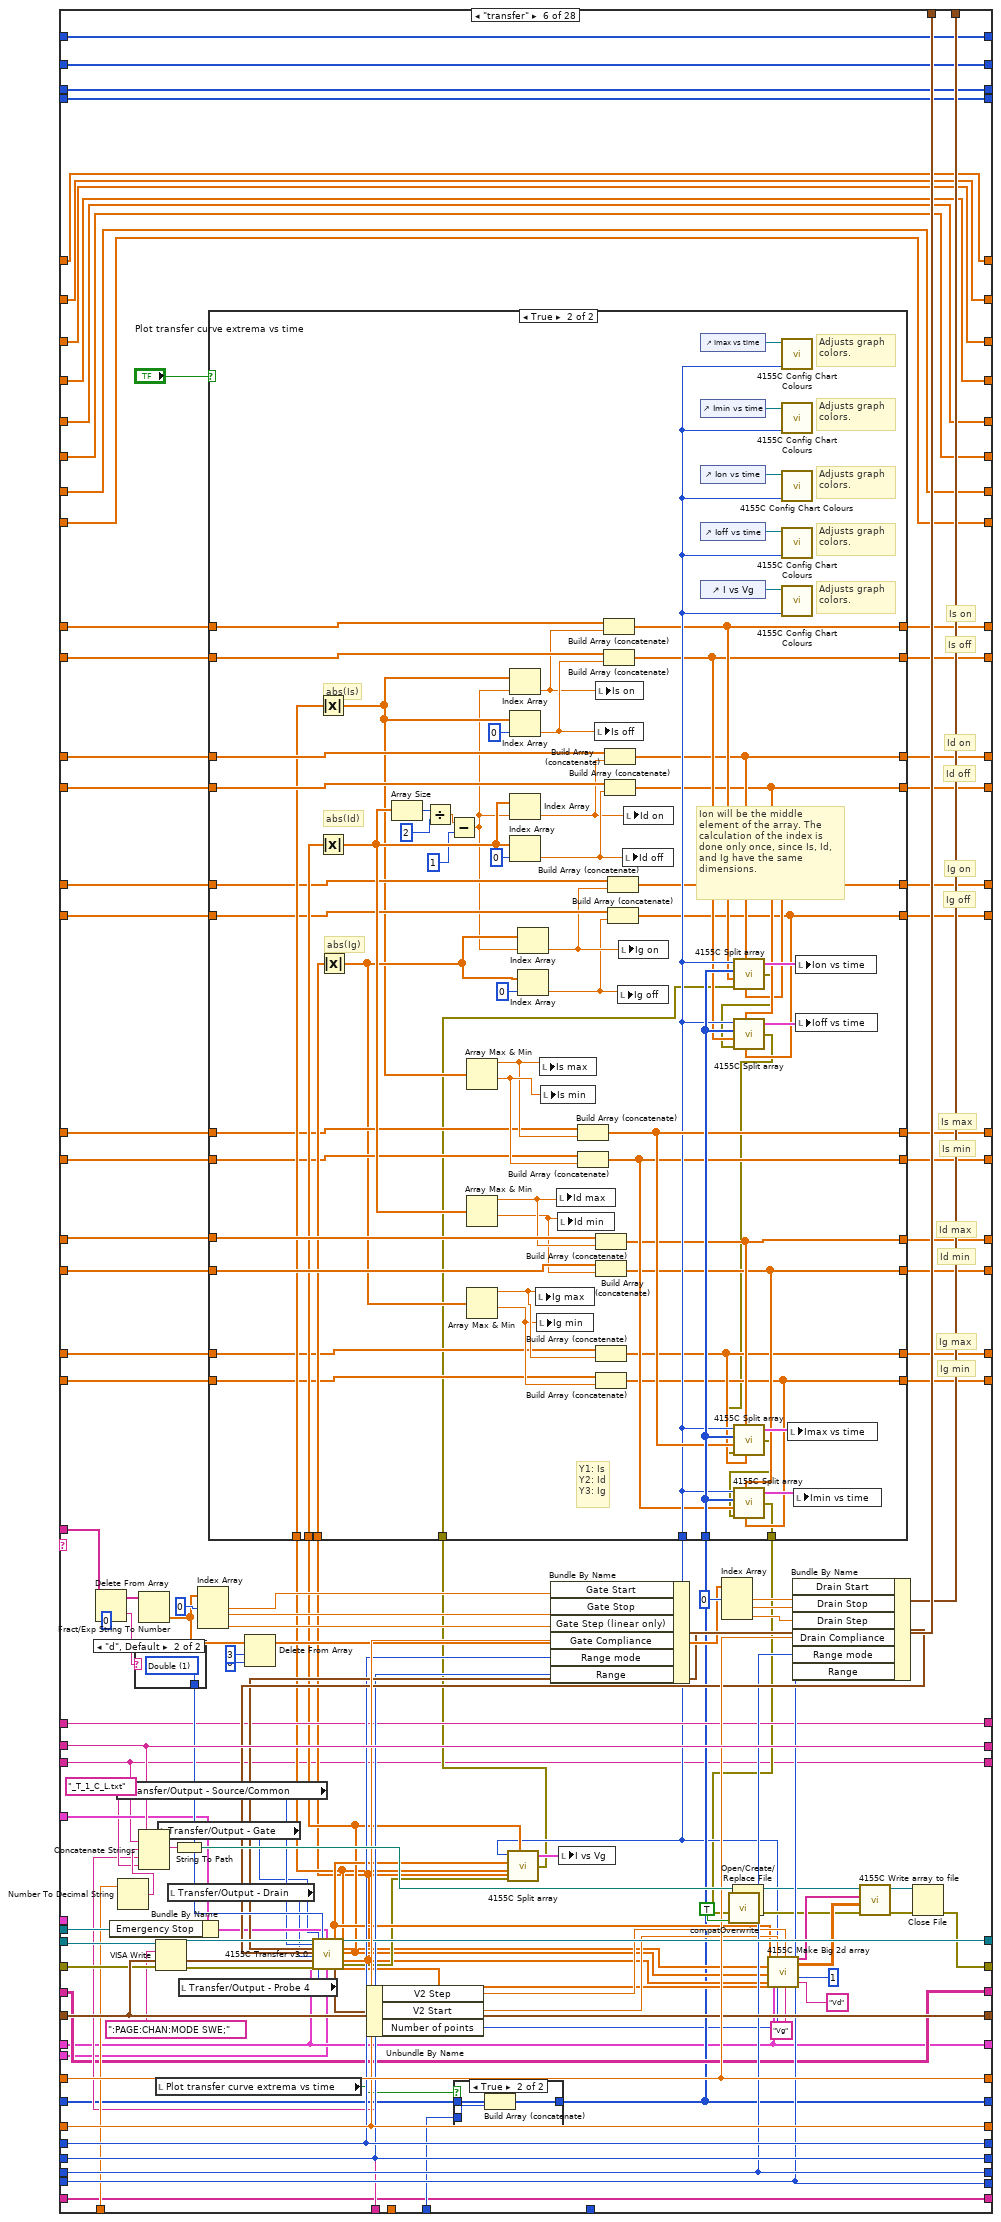
[diagram p13: hidden frame]
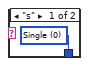
[diagram p16: hidden frame]
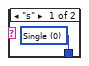
[diagram p19: hidden frame]
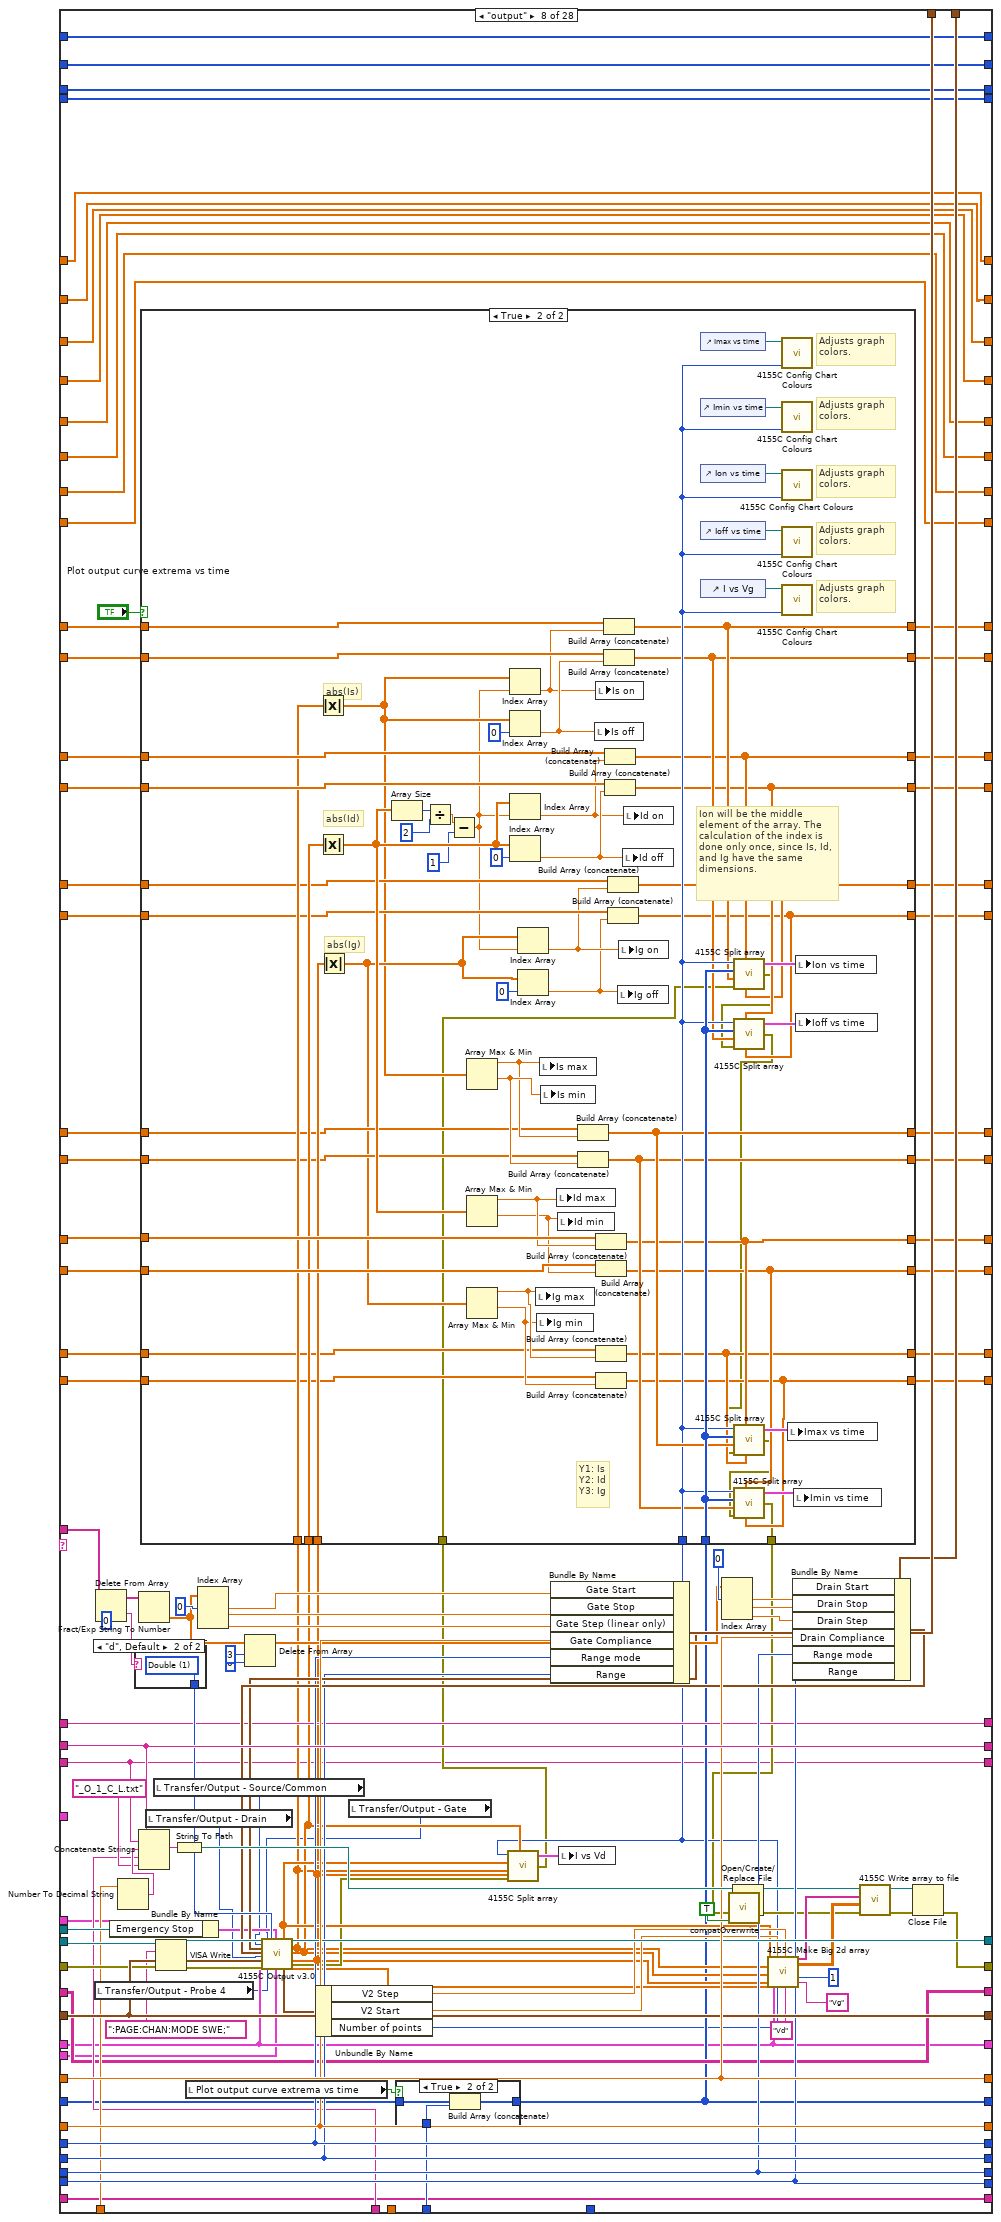
[diagram p20: hidden frame]
diagram:
  w3 = 0.0 ("Is off")
  w2 = cluster{"Y data in":dbl[], "X data in":dbl[]}[] [] ("I vs Vg")
  w12 = 0.0 ("Is off")
  w13 = 0.0 ("Is on")
  w14 = 0.0 ("Is min")
  w15 = 0.0 ("Is max")
  w61 = u16 1 items=["Reset All", "Partial reset"] ("Type of reset")
  # "Change from previous version:\n\n- Added transfer and output extrema plotting for FPP commands."
  # "This is a version specific to the SPM pump."
  # "I add 1 to both the \"total lines\" and the \"line running\" indicators because i and N begin from 0, and the script lines begin from 1."
  # "Bugs:\n\n- If using the \"filename\" command, keep in mind that the arrays of the time-dependent data are not re-initialized inbetween filename changes. \n\n- Do not connect the \"error\" wire of a Split block if it has unconnected terminals! It will halt the program."
  # "Array size"
  # "%s option converts a spreadsheet string to an array of strings."
  # "0: No of rows of array\n1: No of cols"
  # "Dimitrios Simatos\nv. 7.3"
  # "Changes from original textcontrol.vi:\n\n- Timestamp appears in filename.\n- (Only) transfer and output curves are plotted.\n- Communication with serial port.\n- Can execute any command, as all pattern matching functions were replaced. Previously, commands with special LabVIEW characters could not be executed.\n- Replaced write to file function with write to text file.\n- Replaced while loop with for loop.\n- Replaced 4155C \"Save File\" function and now the vi can save time-dependent variables.\n- Added clock with start time control and various units.\n- Changed filepath in which the program is saved.\n- Added a serial output log that keeps a history.\n- Tab control.\n- Addition of specialized serial read/write file for the SPM OEM pump.\n- Added halt and hard stop.\n- Added option for plotting transfer and output curve extrema vs time.\n- Corrected bug of \"itime\" command. The command did not allow for settting the integration time value, it allowed to set the category of the integration time (short, medium, long). If the time value was beyond the range of the category, then the SPA used the closest value allowed, whilst staying in the category. So, if the integration time was changed to long, but the integration time value was a short one, then the SPA would measure using the minimum long integration time value and not the value that the user intended.\n- Added Probe4 command.\n- Added plotting of \"sample\" plots.\n- Added SMU control.\n- Added universal SMU/VSU selector."
  # "Search and replace LF with EOL"
  n1 = Equal?(x="integration time", y=u32 0) -> (x = y?=w62:bool)
  n2 = Select(t="Integration time (short)", s=w62, f="Integration time (long)") -> (s? t:f=w16:dbl)
  n3 = call "4155C Get Filename.vi"("error in (no error)"=errorcluster {"status"=FALSE, "code"=0, "source"=""}) -> ("error out"=w56:errorcluster, "path"=w31:path)  [unwired: 2 in, 1 out]
  "Path" <- w31
  n4 = Bundle By Name(cluster="Timings (overwritten by the Front Panel)", "integration time"="integration time", "Short/Long integration time"=w16) -> (w54:T5)
  n5 = Path To String(path=w31) -> (string=w32:string)
  n6 = Search and Replace String(replace all?=TRUE ("replace all? (F)"), input string="Script", search string="\n", replace string="\r\n") -> (result string=w44:string)  [unwired: 4 in, 3 out]
  n7 = Match Pattern(string=w32, regular expression=".txt") -> (before substring=w28:string)  [unwired: 1 in, 3 out]
  n8 = call "4155C Initialise.vi"("VISA resource name in"="VISA resource name in", "Reset"="Full Reset", "Type of reset"=w61, "error in (no error)"=w56, "VISA Timeout Value"=u32 10000) -> ("VISA Resource Name out"=w55:refnum<visa-resource-name>, "error out"=w5:errorcluster)
  n9 = Concatenate Strings(w28, "Suffix (script)") -> (w27:string)
  n10 = Spreadsheet String To Array(delimiter (Tab)="\r\n", format string="%s", spreadsheet string="Script", array type (2D Dbl)="") -> (array=w35:string[][])
  n11 = String To Path(string=w27) -> (path=w8:path)
  n12 = Array Size(array=w35) -> (size(s)=w39:i32[])
  n13 = Initialize Array("") -> (w20:string[])  [unwired: 1 in]
  n14 = Open/Create/Replace File(file path (use dialog)=w8, error in=w5, operation (0:open)=T8."replace or create with confirmation") -> (refnum out=w7:refnum<file>, error out=w6:errorcluster)  [unwired: 3 in, 1 out]
  n15 = Initialize Array(0 ("element")) -> (w22:i32[])  [unwired: 1 in]
  n16 = Initialize Array("") -> (w18:string[][])  [unwired: 2 in]
  n17 = Initialize Array(0.0 ("element")) -> (w1:dbl[])  [unwired: 1 in]
  n18 = Index Array(array=w39, index=0) -> (element=w37:i32)
  n19 = Write to Text File(file (use dialog)=w7, text=w44, error in=w6) -> (error out=w26:errorcluster)  [unwired: 1 in, 2 out]
  n20 = for {
    N: w37 -> [w215]
    shift-left: "Source/Drain Range" -> [w255]
    shift-right: [w251] -> _
    shift-left: "Source/Drain\nRange mode" -> [w256]
    shift-right: [w252] -> _
    shift-left: "Gate Range" -> [w257]
    shift-right: [w253] -> _
    shift-left: "Gate Range\nmode" -> [w258]
    shift-right: [w254] -> _
    shift-left: "Gate: Compliance" -> [w266]
    shift-right: [w263] -> _
    shift-left: "Drain: Compliance" -> [w267]
    shift-right: [w264] -> _
    shift-left: w54 -> [w268]
    shift-right: [w77] -> _
    shift-left: w26 -> [w269]
    shift-right: [w76] -> _
    shift-left: w55 -> [w270]
    shift-right: [w265] -> _
    shift-left: w28 -> [w271]
    shift-right: [w86] -> _
    tunnel: "Panel Controls 2" -> [w249]
    shift-right: [w127] -> _
    shift-left: w1 -> [w248]
    shift-right: [w185] -> _
    shift-left: i32[] [] -> [w244]
    tunnel: w35 -> [w243] mode=indexing
    shift-right: [w126] -> _
    shift-left: w1 -> [w220]
    shift-right: [w158] -> _
    shift-left: w20 -> [w207]
    shift-right: [w186] -> _
    shift-left: w22 -> [w202]
    shift-right: [w168] -> _
    shift-left: w22 -> [w201]
    shift-right: [w200] -> _
    shift-left: "" -> [w199]
    shift-right: [w163] -> _
    shift-left: w22 -> [w183]
    shift-right: [w162] -> _
    shift-left: w22 -> [w167]
    shift-right: [w159] -> _
    shift-left: w18 -> [w161]
    shift-right: [w120] -> _
    shift-left: w1 -> [w148]
    shift-right: [w121] -> _
    shift-left: w1 -> [w147]
    shift-right: [w125] -> _
    shift-left: w1 -> [w136]
    shift-right: [w124] -> _
    shift-left: w1 -> [w135]
    shift-right: [w118] -> _
    shift-left: w1 -> [w134]
    shift-right: [w128] -> _
    shift-left: w1 -> [w133]
    shift-right: [w119] -> _
    shift-left: w1 -> [w132]
    shift-right: [w117] -> _
    shift-left: w1 -> [w131]
    shift-right: [w123] -> _
    shift-left: w1 -> [w130]
    shift-right: [w122] -> _
    shift-left: w1 -> [w129]
    shift-right: [w85] -> _
    shift-left: "Filename (variable part)" -> [w112]
    shift-right: [w78] -> _
    shift-left: "Probe 4" -> [w250]
    shift-right: [w81] -> _
    shift-left: w1 -> [w107]
    shift-right: [w82] -> _
    shift-left: w1 -> [w106]
    shift-right: [w83] -> _
    shift-left: w1 -> [w105]
    shift-right: [w84] -> _
    shift-left: w1 -> [w104]
    shift-right: [w72] -> _
    shift-left: w1 -> [w75]
    shift-right: [w73] -> _
    shift-left: w1 -> [w74]
    shift-right: [w68] -> _
    shift-left: w1 -> [w69]
    shift-right: [w67] -> _
    shift-left: w1 -> [w70]
    i -> [w210]
    stop <- "Interrupt program" stop-if-true
    w71 = FALSE
    # "Vdg for bias stress plots"
    # "Idg for bias stress plots"
    # "Vp2 for FPP bias stress plots"
    # "Vp1 for FPP bias stress plots"
    # "Ig for bias stress plots"
    # "Id for bias stress plots"
    # "Is for bias stress plots"
    # "Time axis for bias stress plots"
    # "Is off"
    # "Is on"
    # "Ig off"
    # "Ig on"
    # "Is min"
    # "Is max"
    # "Ig min"
    # "Ig max"
    # "Id min"
    # "Id max"
    # "Id off"
    # "Id on"
    # "Vdg for bias stress plots"
    # "Idg for bias stress plots"
    # "Vp2 for FPP bias stress plots"
    # "Vp1 for FPP bias stress plots"
    # "Ig for bias stress plots"
    # "Id for bias stress plots"
    # "Is for bias stress plots"
    # "Time axis for bias stress plots"
    # "Save bias stress curves in file."
    # "Filename prefix"
    # "Is off"
    # "Is on"
    # "Ig off"
    # "Ig on"
    # "Is min"
    # "Is max"
    # "Ig min"
    # "Ig max"
    # "Id min"
    # "Id max"
    # "Id off"
    # "Id on"
    # "Pump status"
    # "Filepath and name"
    # "Pump status"
    # "Limit of command arguments (array columns). Raise if needed."
    # "Serial port data (string)"
    # "Serial port data (table)"
    # "Time array for valve position"
    # "Time array for absolute plunger position"
    # "Valve position"
    # "Absolute plunger position"
    # "Serial port data"
    # "For loop counter"
    # "<-----Equivalent to the 4155C \"Write\" subvi.----->"
    # "Headers"
    # "Save transfer curves in file."
    # "Filepath and name"
    # "Save time-dependent data."
    # "Use the time offset if your measurements do not start at t=0."
    # "Time for Imax, Imin, Ion, Ioff"
    # "Rest of elements of command"
    # "First element of command\n(case select)"
    n21 = Add(x=w210, y=1) -> (x+y=→"Line running":i32)
    n22 = Add(x=w215, y=1) -> (x+y=→"Total lines":i32)
    n23 = Index Array(array=w243, index=0 ("line index")) -> (element=w238:string)
    "Command running:" <- w238
    n24 = control-ref of="Interrupt scan"() -> (w262:refnum<vi>)
    n25 = Spreadsheet String To Array(delimiter (Tab)=" ", format string="%s", spreadsheet string=w238, array type (2D Dbl)=string[] []) -> (array=w236:string[])
    n26 = Delete From Array(array=w236, index=0) -> (deleted portion=w149:string, array with subset deleted=w235:string[])  [unwired: 1 in]
    n27 = call "Elapsed Time"("Reset"="Reset", "Auto Reset"="Auto Reset") -> ("Elapsed Time (s)"=w245:dbl)  [unwired: 10 in, 7 out]
    n28 = case shown="1" "Time Units" {
      tunnel: ["-sec" "-min" "-h"] -> w246
      tunnel: [w275 w279 w282] -> w216
      tunnel: w245 -> [w275 w278 w283]
      frame 0, Default {
      }
      frame 1 {
        n29 = Divide(x=w278, y=60.0) -> (x/y=w279:dbl)
      }
      frame 2 {
        n30 = Divide(x=w283, y=3600.0) -> (x/y=w282:dbl)
      }
    }
    n31 = Add(x=w216, y="Time Offset") -> (x+y=w108:dbl)
    n32 = To Long Integer(number=w108) -> (32bit integer=w109:i32)
    "Elapsed Time" <- w109
    n33 = case shown="\"transfer-fpp\"" w149 {
      tunnel: w235 -> [w329 w376 w422 w434 w500 w688 w823 w1100 w1236 w1417 w1506 w1561 w1614 w1663 w1705 _ _ w1928 w2084 _ w2217 w2291 w2362 w2489 w2647 w2739 w2816 w2873]
      tunnel: w271 -> [w324 w372 w420 w456 w564 w695 w893 w1107 w1306 w1440 w1495 w1553 w1607 w1657 w1698 w1745 w1815 w1855 w2068 w2134 w2204 w2278 w2350 w2483 w2643 w2741 w2818 w2875]
      tunnel: w270 -> [w323 w371 w411 w454 w549 w666 w864 w1078 w1276 w1441 w1496 w1554 w1608 w1658 w1699 w1750 w1817 w1933 w2090 w2138 w2223 w2297 w2368 w2495 w2607 w2745 w2822 w2877]
      tunnel: w269 -> [w322 w370 w410 w453 w548 w665 w863 w1077 w1273 w1442 w1497 w1555 w1609 w1659 w1700 w1749 w1788 w1932 w2089 w2137 w2222 w2296 w2367 w2494 w2606 w2744 w2821 w2878]
      tunnel: w268 -> [w321 w369 w419 w451 w525 w691 w889 w1103 w1302 w1450 w1505 w1552 w1606 w1656 w1697 w1748 w1812 w1903 w2060 w2143 w2197 w2271 w2343 w2482 w2642 w2746 w2823 w2880]
      tunnel: w267 -> [w320 w368 w418 w450 w562 w693 w891 w1105 w1304 w1449 w1504 w1560 w1613 w1662 w1704 w1747 w1797 w1931 w2088 w2146 w2221 w2295 w2366 w2493 w2651 w2747 w2824 w2881]
      tunnel: w266 -> [w319 w367 w417 w448 w561 w692 w890 w1104 w1303 w1448 w1503 w1559 w1612 w1661 w1703 w1746 w1798 w1911 w2069 w2145 w2205 w2279 w2351 w2484 w2644 w2749 w2825 w2883]
      tunnel: [w323 w371 w409 w454 w559 w690 w888 w1102 w1301 w1441 w1496 w1554 w1608 w1658 w1699 w1750 w1817 w1904 w2042 w2136 w2198 w2272 w2344 w2442 w2609 w2745 w2822 w2877] -> w265
      tunnel: [w322 w370 w408 w453 w558 w689 w887 w1101 w1300 w1442 w1497 w1555 w1609 w1659 w1700 w1749 w1787 w1912 w2043 w2135 w2206 w2280 w2352 w2441 w2608 w2743 w2820 w2878] -> w182
      tunnel: [w321 w369 w419 w451 w521 w691 w889 w1103 w1302 w1443 w1498 w1552 w1606 w1656 w1697 w1748 w1812 w1903 w2060 w2143 w2197 w2271 w2343 w2482 w2642 w2746 w2823 w2880] -> w77
      tunnel: [w320 w368 w418 w450 w562 w693 w891 w1105 w1304 w1449 w1504 w1560 w1613 w1662 w1704 w1747 w1797 w1931 w2088 w2146 w2221 w2295 w2366 w2493 w2651 w2747 w2824 w2881] -> w264
      tunnel: [w319 w367 w417 w448 w561 w692 w890 w1104 w1303 w1448 w1503 w1559 w1612 w1661 w1703 w1746 w1798 w1911 w2069 w2145 w2205 w2279 w2351 w2484 w2644 w2749 w2825 w2883] -> w263
      tunnel: [w324 w372 w420 w456 w564 w695 w893 w1107 w1306 w1440 w1495 w1553 w1607 w1657 w1698 w1745 w1815 w1855 w2068 w2134 w2204 w2278 w2350 w2483 w2643 w2741 w2818 w2875] -> w86
      tunnel: w262 -> [_ _ _ _ w568 w697 w897 w1109 w1310 _ _ _ _ _ _ _ _ w1908 w2065 _ w2203 w2277 w2349 w2461 w2625 _ _ _]
      tunnel: "Gate" -> [_ _ _ _ w552 w675 w874 w1087 w1287 _ _ _ _ _ _ _ _ _ _ _ _ _ _ _ _ _ _ _]
      tunnel: "Drain 2" -> [_ _ _ _ w551 w674 w873 w1086 w1286 _ _ _ _ _ _ _ _ _ _ _ _ _ _ _ _ _ _ _]
      tunnel: "Panel Controls" -> [_ _ _ _ _ _ w872 w1007 w1285 _ _ _ _ _ _ _ _ _ _ _ _ _ _ _ _ _ _ _]
      tunnel: w258 -> [w318 w366 w416 w447 w542 w659 w857 w1071 w1271 w1447 w1502 _ w1605 w1655 w1696 w1744 w1799 w1899 w2056 w2139 w2193 w2267 w2339 w2478 w2638 w2750 w2826 w2884]
      tunnel: w257 -> [w317 w365 w415 w446 w541 w658 w856 w1070 w1270 w1446 w1501 w1558 _ w1646 w1702 w1743 w1800 w1900 w2057 w2140 w2194 w2268 w2340 w2479 w2639 w2751 w2827 w2885]
      tunnel: w256 -> [w316 w364 w414 w445 w540 w657 w855 w1069 w1269 w1445 w1500 w1557 w1611 w1660 _ w1742 w1801 w1901 w2058 w2141 w2195 w2269 w2341 w2480 w2640 w2752 w2828 w2886]
      tunnel: w255 -> [w315 w363 w413 w444 w539 w656 w854 w1068 w1272 w1444 w1499 w1556 w1610 _ w1701 w1741 w1802 w1902 w2059 w2142 w2196 w2270 w2342 w2481 w2641 w2753 w2829 w2887]
      tunnel: [w318 w366 w416 w447 w542 w659 w857 w1071 w1271 w1447 w1502 w1551 w1605 w1655 w1696 w1744 w1799 w1899 w2056 w2139 w2193 w2267 w2339 w2478 w2638 w2750 w2826 w2884] -> w254
      tunnel: [w317 w365 w415 w446 w541 w658 w856 w1070 w1270 w1446 w1501 w1558 w1597 w1646 w1702 w1743 w1800 w1900 w2057 w2140 w2194 w2268 w2340 w2479 w2639 w2751 w2827 w2885] -> w253
      tunnel: [w316 w364 w414 w445 w540 w657 w855 w1069 w1269 w1445 w1500 w1557 w1611 w1660 w1695 w1742 w1801 w1901 w2058 w2141 w2195 w2269 w2341 w2480 w2640 w2752 w2828 w2886] -> w252
      tunnel: [w315 w363 w413 w444 w539 w656 w854 w1068 w1272 w1444 w1499 w1556 w1610 w1647 w1701 w1741 w1802 w1902 w2059 w2142 w2196 w2270 w2342 w2481 w2641 w2753 w2829 w2887] -> w251
      tunnel: w250 -> [w293 w338 w385 _ w488 w592 w836 w1004 w1253 w1414 w1472 w1529 w1575 w1624 w1673 w1719 w1759 w1876 w2017 w2112 w2158 w2236 w2309 w2422 w2585 w2704 w2765 w2871]
      tunnel: w249 -> [_ _ _ _ w536 w650 _ _ _ _ _ _ _ _ _ _ _ _ _ _ _ _ _ _ _ _ _ _]
      tunnel: [w314 w359 w406 w461 w513 w607 w807 w1020 w1230 w1439 w1493 w1550 w1596 w1645 w1694 w1740 w1783 w1865 w2022 w2133 w2182 w2260 w2333 w2397 w2566 w2742 w2819 w2892] -> w127
      tunnel: w248 -> [w314 w359 w406 w461 w513 w647 w814 w1060 w1196 w1439 w1493 w1550 w1596 w1645 w1694 w1740 w1783 w1872 w2022 w2133 w2182 w2260 w2333 w2403 w2570 w2742 w2819 w2892]
      tunnel: w108 -> [_ _ _ _ w510 w646 w847 w1059 w1263 _ _ _ _ _ _ _ w1781 w1892 w2039 _ w2179 w2257 w2330 w2438 w2600 _ _ _]
      tunnel: w246 -> [_ _ _ _ w509 w643 w845 w1056 w1262 _ _ _ _ _ _ _ w1779 w1890 w2038 _ w2178 w2256 w2329 w2437 w2601 _ w2792 _]
      tunnel: w109 -> [_ _ _ _ _ w639 w826 w1052 w1239 _ _ _ _ _ _ _ _ _ _ _ _ _ _ _ _ _ w2795 _]
      tunnel: [w313 w358 w405 w449 w512 w611 w786 w1024 w1199 w1438 w1492 w1549 w1595 w1644 w1693 w1739 w1782 w1857 w2005 w2132 w2181 w2259 w2332 w2391 w2560 w2748 w2799 w2882] -> w185
      tunnel: w244 -> [w313 w358 w405 w449 w512 w642 w825 w1055 w1238 w1438 w1492 w1549 w1595 w1644 w1693 w1739 w1782 w1861 w2006 w2132 w2181 w2259 w2332 w2392 w2561 w2748 w2799 w2882]
      tunnel: [w312 w357 w404 w460 w508 w606 w808 w1019 w1231 w1437 w1491 w1548 w1594 w1643 w1692 w1738 w1778 w1864 w2021 w2131 w2177 w2255 w2328 w2396 w2565 w2737 w2815 w2891] -> w126
      tunnel: w220 -> [w312 w357 w404 w460 w508 w638 w813 w1051 w1229 w1437 w1491 w1548 w1594 w1643 w1692 w1738 w1778 w1871 w2021 w2131 w2177 w2255 w2328 w2402 w2569 w2737 w2815 w2891]
      tunnel: [w311 w356 w403 w443 w507 w631 w844 w1044 w1261 w1436 w1490 w1547 w1593 w1642 w1691 w1737 w1777 w1889 w2037 w2130 w2176 w2254 w2327 w2436 w2599 w2736 w2814 w2888] -> w158
      tunnel: w207 -> [w311 w356 w403 w443 w507 w631 w844 w1044 w1261 w1436 w1490 w1547 w1593 w1642 w1691 w1737 w1777 w1889 w2037 w2130 w2176 w2254 w2327 w2436 w2599 w2735 w2793 w2888]
      tunnel: [w310 w355 w402 w471 w506 w630 w843 w1043 w1260 w1435 w1489 w1546 w1592 w1641 w1690 w1736 w1776 w1888 w2036 w2129 w2175 w2253 w2326 w2435 w2598 w2721 w2801 w2902] -> w186
      tunnel: w202 -> [w310 w355 w402 w471 w506 w630 w843 w1043 w1260 w1435 w1489 w1546 w1592 w1641 w1690 w1736 w1776 w1888 w2036 w2129 w2175 w2253 w2326 w2435 w2598 w2721 w2800 w2902]
      tunnel: [w309 w354 w401 w473 w505 w629 w842 w1042 w1259 w1434 w1488 w1545 w1591 w1640 w1689 w1735 w1775 w1887 w2035 w2128 w2174 w2252 w2325 w2434 w2597 w2720 w2788 w2904] -> w168
      tunnel: w201 -> [w309 w354 w401 w473 w505 w629 w842 w1042 w1259 w1434 w1488 w1545 w1591 w1640 w1689 w1735 w1775 w1887 w2035 w2128 w2174 w2252 w2325 w2434 w2597 w2720 w2786 w2904]
      tunnel: [w308 w353 w400 w457 w504 w628 w841 w1041 w1258 w1433 w1487 w1544 w1590 w1639 w1688 w1734 w1774 w1886 w2034 w2127 w2173 w2251 w2324 w2433 w2596 w2719 w2785 w2876] -> w200
      tunnel: w199 -> [w308 w353 w400 w457 w504 w628 w841 w1041 w1258 w1433 w1487 w1544 w1590 w1639 w1688 w1734 w1774 w1886 w2034 w2127 w2173 w2251 w2324 w2433 w2596 w2719 w2796 w2876]
      tunnel: w109 -> [_ _ _ _ _ _ _ _ _ _ _ _ _ _ _ _ _ _ _ _ _ _ _ _ _ _ w2784 _]
      tunnel: w183 -> [w307 w352 w399 w472 w503 w627 w840 w1040 w1257 w1432 w1486 w1543 w1589 w1638 w1687 w1733 w1773 w1885 w2033 w2126 w2172 w2250 w2323 w2432 w2595 w2718 w2783 w2903]
      tunnel: [w307 w352 w399 w472 w503 w627 w840 w1040 w1257 w1432 w1486 w1543 w1589 w1638 w1687 w1733 w1773 w1885 w2033 w2126 w2172 w2250 w2323 w2432 w2595 w2718 w2782 w2903] -> w163
      tunnel: [w306 w351 w398 w470 w502 w626 w839 w1039 w1256 w1431 w1485 w1542 w1588 w1637 w1686 w1732 w1772 w1884 w2032 w2125 w2171 w2249 w2322 w2431 w2594 w2717 w2781 w2901] -> w162
      tunnel: w167 -> [w306 w351 w398 w470 w502 w626 w839 w1039 w1256 w1431 w1485 w1542 w1588 w1637 w1686 w1732 w1772 w1884 w2032 w2125 w2171 w2249 w2322 w2431 w2594 w2717 w2780 w2901]
      tunnel: [w305 w350 w397 w452 w501 w625 w838 w1038 w1255 w1430 w1484 w1541 w1587 w1636 w1685 w1731 w1771 w1883 w2031 w2124 w2170 w2248 w2321 w2430 w2593 w2716 w2778 w2879] -> w159
      tunnel: w161 -> [w305 w350 w397 w452 w501 w625 w838 w1038 w1255 w1430 w1484 w1541 w1587 w1636 w1685 w1731 w1771 w1883 w2031 w2124 w2170 w2248 w2321 w2430 w2593 w2716 w2777 w2879]
      tunnel: [w303 w348 w395 w466 w498 w600 w802 w1013 w1216 w1428 w1483 w1540 w1585 w1634 w1683 w1729 w1769 w1882 w2030 w2123 w2169 w2247 w2319 w2429 w2592 w2715 w2776 w2897] -> w120
      tunnel: w148 -> [w303 w348 w395 w466 w498 w624 w819 w1037 w1219 w1428 w1483 w1540 w1585 w1634 w1683 w1729 w1769 w1882 w2030 w2123 w2169 w2247 w2319 w2429 w2592 w2715 w2776 w2897]
      tunnel: [w304 w349 w396 w467 w499 w601 w801 w1014 w1215 w1429 w1482 w1539 w1586 w1635 w1684 w1730 w1770 w1881 w2029 w2122 w2168 w2246 w2320 w2428 w2591 w2714 w2775 w2898] -> w121
      tunnel: w147 -> [w304 w349 w396 w467 w499 w623 w820 w1036 w1220 w1429 w1482 w1539 w1586 w1635 w1684 w1730 w1770 w1881 w2029 w2122 w2168 w2246 w2320 w2428 w2591 w2714 w2775 w2898]
      tunnel: [w296 w341 w388 w459 w495 w605 w809 w1018 w1232 w1421 w1480 w1537 w1583 w1632 w1681 w1727 w1762 w1863 w2020 w2121 w2161 w2239 w2312 w2395 w2564 w2707 w2774 w2890] -> w125
      tunnel: w136 -> [w296 w341 w388 w459 w495 w619 w812 w1032 w1235 w1421 w1480 w1537 w1583 w1632 w1681 w1727 w1762 w1870 w2020 w2121 w2161 w2239 w2312 w2401 w2568 w2707 w2774 w2890]
      tunnel: [w295 w340 w387 w458 w496 w604 w810 w1017 w1233 w1420 w1481 w1538 w1584 w1633 w1682 w1728 w1761 w1862 w2019 w2120 w2160 w2238 w2311 w2394 w2563 w2706 w2773 w2889] -> w124
      tunnel: w135 -> [w295 w340 w387 w458 w496 w618 w811 w1031 w1234 w1420 w1481 w1538 w1584 w1633 w1682 w1728 w1761 w1869 w2019 w2120 w2160 w2238 w2311 w2400 w2567 w2706 w2773 w2889]
      tunnel: [w298 w343 w390 w463 w494 w610 w805 w1023 w1226 w1426 w1478 w1535 w1581 w1630 w1679 w1725 w1764 w1867 w2024 w2115 w2163 w2241 w2314 w2399 w2573 w2711 w2771 w2894] -> w118
      tunnel: w134 -> [w298 w343 w390 w463 w494 w617 w816 w1030 w1227 w1426 w1478 w1535 w1581 w1630 w1679 w1725 w1764 w1874 w2024 w2115 w2163 w2241 w2314 w2405 w2574 w2711 w2771 w2894]
      tunnel: [w297 w342 w389 w462 w497 w608 w806 w1021 w1225 w1427 w1479 w1536 w1582 w1631 w1680 w1726 w1763 w1866 w2023 w2114 w2162 w2240 w2313 w2398 w2571 w2710 w2772 w2893] -> w128
      tunnel: w133 -> [w297 w342 w389 w462 w497 w616 w815 w1029 w1228 w1427 w1479 w1536 w1582 w1631 w1680 w1726 w1763 w1873 w2023 w2114 w2162 w2240 w2313 w2404 w2572 w2710 w2772 w2893]
      tunnel: [w300 w345 w392 w465 w493 w599 w804 w1012 w1224 w1424 w1476 w1533 w1579 w1628 w1677 w1723 w1766 w1878 w2026 w2117 w2165 w2243 w2316 w2425 w2588 w2713 w2769 w2896] -> w119
      tunnel: w132 -> [w300 w345 w392 w465 w493 w615 w818 w1028 w1221 w1424 w1476 w1533 w1579 w1628 w1677 w1723 w1766 w1878 w2026 w2117 w2165 w2243 w2316 w2425 w2588 w2713 w2769 w2896]
      tunnel: [w299 w344 w391 w464 w492 w598 w803 w1011 w1223 w1425 w1477 w1534 w1580 w1629 w1678 w1724 w1765 w1877 w2025 w2116 w2164 w2242 w2315 w2424 w2587 w2712 w2770 w2895] -> w117
      tunnel: w131 -> [w299 w344 w391 w464 w492 w614 w817 w1027 w1222 w1425 w1477 w1534 w1580 w1629 w1678 w1724 w1765 w1877 w2025 w2116 w2164 w2242 w2315 w2424 w2587 w2712 w2770 w2895]
      tunnel: [w302 w347 w394 w469 w491 w603 w799 w1016 w1213 w1422 w1474 w1531 w1577 w1626 w1675 w1721 w1768 w1880 w2028 w2119 w2167 w2245 w2318 w2427 w2590 w2709 w2767 w2900] -> w123
      tunnel: w130 -> [w302 w347 w394 w469 w491 w613 w822 w1026 w1217 w1422 w1474 w1531 w1577 w1626 w1675 w1721 w1768 w1880 w2028 w2119 w2167 w2245 w2318 w2427 w2590 w2709 w2767 w2900]
      tunnel: [w301 w346 w393 w468 w490 w602 w800 w1015 w1214 w1423 w1475 w1532 w1578 w1627 w1676 w1722 w1767 w1879 w2027 w2118 w2166 w2244 w2317 w2426 w2589 w2708 w2768 w2899] -> w122
      tunnel: w129 -> [w301 w346 w393 w468 w490 w612 w821 w1025 w1218 w1423 w1475 w1532 w1578 w1627 w1676 w1722 w1767 w1879 w2027 w2118 w2166 w2244 w2317 w2426 w2589 w2708 w2768 w2899]
      tunnel: w112 -> [w294 w339 w386 w455 w489 w595 w837 w1008 w1254 w1419 w1473 w1530 w1576 w1625 w1674 w1720 w1760 w1854 w2018 w2113 w2159 w2237 w2310 w2423 w2586 w2705 w2766 _]
      tunnel: [w294 w339 w386 w455 w489 w595 w837 w1008 w1254 w1419 w1473 w1530 w1576 w1625 w1674 w1720 w1760 w1854 w2018 w2113 w2159 w2237 w2310 w2423 w2586 w2705 w2766 w2872] -> w85
      tunnel: [w293 w338 w385 w433 w488 w592 w836 w1004 w1253 w1414 w1472 w1529 w1575 w1624 w1673 w1719 w1759 w1876 w2017 w2112 w2158 w2236 w2309 w2422 w2585 w2704 w2765 w2871] -> w78
      tunnel: w108 -> [_ _ _ _ _ _ _ _ _ _ _ _ _ _ _ _ _ w1824 w2001 _ _ _ _ w2407 w2577 _ _ _]
      tunnel: [w292 w337 w384 w432 w487 w591 w794 w1003 w1205 w1413 w1471 w1528 w1574 w1623 w1672 w1718 w1758 w1838 w2016 w2111 w2157 w2235 w2308 w2412 w2581 w2703 w2764 w2870] -> w81
      tunnel: [w291 w336 w383 w431 w486 w590 w795 w1002 w1206 w1412 w1470 w1527 w1573 w1622 w1671 w1717 w1757 w1837 w2015 w2110 w2156 w2234 w2307 w2373 w2542 w2702 w2763 w2869] -> w82
      tunnel: [w290 w335 w382 w430 w485 w589 w796 w1001 w1207 w1411 w1469 w1526 w1572 w1621 w1670 w1716 w1756 w1839 w1988 w2109 w2155 w2233 w2306 w2385 w2554 w2701 w2762 w2868] -> w83
      tunnel: [w289 w334 w381 w429 w484 w588 w797 w1000 w1208 w1410 w1468 w1525 w1571 w1620 w1669 w1715 w1755 w1836 w1995 w2108 w2154 w2232 w2305 w2382 w2551 w2700 w2761 w2867] -> w84
      tunnel: w107 -> [w292 w337 w384 w432 w487 w591 w794 w1003 w1205 w1413 w1471 w1528 w1574 w1623 w1672 w1718 w1758 w1835 w2016 w2111 w2157 w2235 w2308 w2415 w2584 w2703 w2764 w2870]
      tunnel: w106 -> [w291 w336 w383 w431 w486 w590 w795 w1002 w1206 w1412 w1470 w1527 w1573 w1622 w1671 w1717 w1757 w1834 w2015 w2110 w2156 w2234 w2307 w2414 w2583 w2702 w2763 w2869]
      tunnel: w105 -> [w290 w335 w382 w430 w485 w589 w796 w1001 w1207 w1411 w1469 w1526 w1572 w1621 w1670 w1716 w1756 w1833 w1989 w2109 w2155 w2233 w2306 w2385 w2554 w2701 w2762 w2868]
      tunnel: w104 -> [w289 w334 w381 w429 w484 w588 w797 w1000 w1208 w1410 w1468 w1525 w1571 w1620 w1669 w1715 w1755 w1832 w1997 w2108 w2154 w2232 w2305 w2413 w2582 w2700 w2761 w2867]
      tunnel: "Standby" -> [_ _ _ _ w483 w587 _ w999 _ _ _ _ _ _ _ _ _ w1830 w2014 _ _ _ _ w2421 _ _ _ _]
      tunnel: w75 -> [w288 w333 w380 w428 w477 w581 w792 w993 w1203 w1409 w1467 w1524 w1570 w1619 w1668 w1714 w1754 w1821 w2009 w2107 w2150 w2229 w2303 w2379 w2548 w2699 w2760 w2866]
      tunnel: [w288 w333 w380 w428 w477 w581 w792 w993 w1203 w1409 w1467 w1524 w1570 w1619 w1668 w1714 w1754 w1821 w2009 w2107 w2150 w2229 w2303 w2374 w2543 w2699 w2760 w2866] -> w72
      tunnel: w74 -> [w287 w332 w379 w427 w476 w582 w793 w994 w1204 w1408 w1466 w1523 w1569 w1618 w1667 w1713 w1753 w1820 w2008 w2106 w2149 w2228 w2302 w2378 w2547 w2698 w2759 w2865]
      tunnel: [w287 w332 w379 w427 w476 w582 w793 w994 w1204 w1408 w1466 w1523 w1569 w1618 w1667 w1713 w1753 w1820 w2008 w2106 w2149 w2228 w2302 w2377 w2546 w2698 w2759 w2865] -> w73
      tunnel: w70 -> [w285 w330 w377 w425 w475 w580 w791 w992 w1202 w1407 w1465 w1522 w1568 w1616 w1665 w1711 w1751 w1818 w1994 w2104 w2147 w2226 w2300 w2371 w2540 w2696 w2754 w2863]
      tunnel: w69 -> [w286 w331 w378 w426 w474 w579 w790 w991 w1201 w1406 w1464 w1521 w1567 w1617 w1666 w1712 w1752 w1819 w1992 w2105 w2148 w2227 w2301 w2372 w2541 w2697 w2755 w2864]
      tunnel: [w286 w331 w378 w426 w474 w579 w790 w991 w1201 w1406 w1464 w1521 w1567 w1617 w1666 w1712 w1752 w1819 w1986 w2105 w2148 w2227 w2301 w2372 w2541 w2697 w2755 w2864] -> w68
      tunnel: [w285 w330 w377 w425 w475 w580 w791 w992 w1202 w1407 w1465 w1522 w1568 w1616 w1665 w1711 w1751 w1818 w1993 w2104 w2147 w2226 w2300 w2371 w2540 w2696 w2754 w2863] -> w67
      frame "wait" {
        n34 = Index Array(array=w329, index=0 ("Index")) -> (element=w327:string)
        n35 = Decimal String To Number(string=w327, default (0L)=u32 0) -> (number=w326:u32)  [unwired: 1 in, 1 out]
        n36 = Wait (ms)(milliseconds to wait=w326) -> ()  [unwired: 1 out]
      }
      frame "wait-min" {
        n37 = Index Array(array=w376, index=0 ("Index")) -> (element=w374:string)
        n38 = Decimal String To Number(string=w374, default (0L)=u32 0) -> (number=w362:u32)  [unwired: 1 in, 1 out]
        n39 = Multiply(x=w362, y=u32 60000) -> (x*y=w361:u32)
        n40 = Wait (ms)(milliseconds to wait=w361) -> ()  [unwired: 1 out]
      }
      frame "standby" {
        n41 = Index Array(array=w422, index=0 ("Index")) -> (element=w412:string)
        n42 = case shown="\"off\", Default" w412 {
          tunnel: [":PAGE:SCON:STAN 0" ":PAGE:SCON:STAN 1"] -> w407
          frame "off", Default {
          }
          frame "on" {
          }
        }
        n43 = VISA Write(VISA resource name=w411, write buffer=w407, error in (no error)=w410) -> (VISA resource name out=w409:refnum<visa-resource-name>, error out=w408:errorcluster)  [unwired: 1 out]
      }
      frame "Probe4" {
        n44 = Delete From Array(array=w434, index=0) -> (deleted portion=w437:string, array with subset deleted=w440:string[])  [unwired: 1 in]
        n45 = Equal?(x=w437, y="ON") -> (x = y?=w435:bool)
        n46 = Delete From Array(array=w440, index=0) -> (deleted portion=w439:string)  [unwired: 1 in, 1 out]
        n47 = Fract/Exp String To Number(string=w439) -> (number=w436:dbl)  [unwired: 3 in, 1 out]
        n48 = Bundle(w435, w436) -> (w433:cluster{bool, dbl})  [unwired: 1 in]
      }
      frame "pulsedstressV" {
        w519 = 0
        n49 = local read "Pulsed Stress V - Source/Common"() -> (w482:u32)
        n50 = local read "Pulsed Stress V - Probe 4"() -> (w479:u32)
        n51 = Number To Decimal String(number=w510) -> (decimal integer string=w565:string)  [unwired: 1 in]
        n52 = local read "Pulsed Stress V - Vextra"() -> (w478:u32)
        n53 = local read "Pulsed Stress V - Drain"() -> (w481:u32)
        n54 = local read "Pulsed Stress V - Gate"() -> (w480:u32)
        n55 = Delete From Array(array=w500, index=0 ("Index")) -> (deleted portion=w556:string, array with subset deleted=w555:string[])  [unwired: 1 in]
        n56 = Bundle By Name(cluster=w536, "Emergency Stop"=w568) -> (w537:T2)
        n57 = VISA Write(VISA resource name=w549, write buffer=":PAGE:CHAN:MODE SWE;" ("write buffer (\"\")"), error in (no error)=w548) -> (VISA resource name out=w546:refnum<visa-resource-name>, error out=w547:errorcluster)  [unwired: 1 out]
        n58 = Concatenate Strings(w564, "-pulsedstressV-" ("Substring"), w565, w509, ".txt" ("Substring")) -> (w567:string)
        n59 = case shown="\"d\", Default" w556 {
          tunnel: [w577 w578] -> w554
          frame "s" {
            w577 = u16 0 items=["Single", "Double"] ("sweep mode")
          }
          frame "d", Default {
            w578 = u16 1 items=["Single", "Double"] ("sweep mode")
          }
        }
        n60 = Fract/Exp String To Number(string=w555) -> (number=w550:dbl[])  [unwired: 3 in, 1 out]
        n61 = String To Path(string=w567) -> (path=w563:path)
        n62 = Index Array(array=w550, index #1=0 ("Index")) -> (element #1=w528:dbl, element #2=w527:dbl, element #3=w524:dbl, element #4=w523:dbl, element #5=w522:dbl, element #6=w526:dbl)  [unwired: 5 in]
        n63 = Bundle By Name(cluster=w525, "Pulse period"=w523, "Base voltage"=w524, "Pulse width"=w522) -> (w521:T5)
        n64 = Unbundle By Name(w521) -> ("Pulse period"=w529:dbl)
        n65 = Bundle By Name(cluster=w552, "Gate Start"=w527, "Gate Stop"=w528, "Gate Step (linear only)"=0, "Gate Compliance"=w561, "Range mode"=w542, "Range"=w541) -> (w543:T6)
        n66 = call <vilib>:"compatOverwrite.vi"("overwrite (F)"=TRUE) -> ("overwrite?"=w514:T8)
        n67 = Bundle By Name(cluster=w551, "Drain Start"=w526, "Drain Stop"=w519, "Drain Step"=w519, "Drain Compliance"=w562, "Range mode"=w540, "Range"=w539) -> (w544:T7)
        n68 = call "4155C PulsedStressV v3.0.vi"("VISA resource name in"=w546, "Gate"=w543, "Pulsed Stress V - Source/Common"=w482, "Drain"=w544, "Timings"=w521, "error in (no error)"=w547, "sweep mode"=w554, "Probe 4"=w488, "Pulsed Stress V - Drain"=w481, "Pulsed Stress V - Gate"=w480, "Panel Controls"=w537, "Standby"=w483, "Pulsed Stress V - Probe 4"=w479, "Pulsed Stress V - Vextra"=w478) -> ("Outparams"=w538:T9, "VISA Resource Name out"=w559:refnum<visa-resource-name>, "ID"=w517:dbl[], "IG"=w515:dbl[], "error out"=w560:errorcluster)  [unwired: 1 in]
        n69 = Unbundle By Name(w538) -> ("Number of points"=w516:i32)  [unwired: 2 out]
        n70 = for {
          N: w516 -> [_]
          tunnel: [w574] -> w518 mode=indexing
          tunnel: w529 -> [w576]
          i -> [w575]
          n71 = Multiply(x=w576, y=w575) -> (x*y=w574:dbl)
        }
        n72 = Insert Into Array(array=dbl[][] [] ("Input Array"), new element=w518) -> (w530:dbl[][])  [unwired: 2 in]
        n73 = Insert Into Array(array=w530, new element=w517) -> (w535:dbl[][])  [unwired: 2 in]
        n74 = Insert Into Array(array=w535, new element=w515) -> (w534:dbl[][])  [unwired: 2 in]
        n75 = Transpose 2D Array(2D array=w534) -> (transposed array=w533:dbl[][])
        n76 = Open/Create/Replace File(file path (use dialog)=w563, error in=w560, operation (0:open)=w514) -> (refnum out=w571:refnum<file>, error out=w572:errorcluster)  [unwired: 3 in, 1 out]
        n77 = call "4155C Write array to file.vi"("Byte Stream File Refnum"=w571, "Header"=string[] ["Time /s", "Id /A", "Ig /A"], "Data Array"=w533, "error in (no error)"=w572) -> ("dup refnum"=w569:refnum<file>, "error out"=w570:errorcluster)  [unwired: 1 in]
        n78 = Close File(refnum=w569, error in=w570) -> (error out=w558:errorcluster)  [unwired: 1 out]
      }
      frame "transfer" {
        # "Is off"
        # "Is on"
        # "Ig off"
        # "Ig on"
        # "Is min"
        # "Is max"
        # "Ig min"
        # "Ig max"
        # "Id min"
        # "Id max"
        # "Id off"
        # "Id on"
        n79 = Delete From Array(array=w688, index=0 ("Index")) -> (deleted portion=w686:string, array with subset deleted=w685:string[])  [unwired: 1 in]
        n80 = Bundle By Name(cluster=w650, "Emergency Stop"=w697) -> (w651:T2)
        n81 = local read "Transfer/Output - Source/Common"() -> (w586:u32)
        n82 = Number To Decimal String(number=w646) -> (decimal integer string=w645:string)  [unwired: 1 in]
        n83 = case shown="\"d\", Default" w686 {
          tunnel: [w782 w783] -> w684
          frame "s" {
            w782 = u16 0 items=["Single", "Double"] ("sweep mode")
          }
          frame "d", Default {
            w783 = u16 1 items=["Single", "Double"] ("sweep mode")
          }
        }
        n84 = Fract/Exp String To Number(string=w685) -> (number=w670:dbl[])  [unwired: 3 in, 1 out]
        n85 = Concatenate Strings(w695, w595, w645, w643, "_T_1_C_L.txt" ("Suffix (transfer)")) -> (w696:string)
        n86 = VISA Write(VISA resource name=w666, write buffer=":PAGE:CHAN:MODE SWE;" ("write buffer (\"\")"), error in (no error)=w665) -> (VISA resource name out=w663:refnum<visa-resource-name>, error out=w664:errorcluster)  [unwired: 1 out]
        n87 = local read "Plot transfer curve extrema vs time"() -> (w593:bool)
        n88 = local read "Transfer/Output - Gate"() -> (w584:u32)
        n89 = local read "Transfer/Output - Drain"() -> (w585:u32)
        n90 = String To Path(string=w696) -> (path=w694:path)
        n91 = local read "Transfer/Output - Probe 4"() -> (w583:u32)
        n92 = Index Array(array=w670, index #1=0 ("Index")) -> (element #1=w683:dbl, element #2=w682:dbl, element #3=w681:dbl)  [unwired: 2 in]
        n93 = Delete From Array(array=w670, length=3 ("Length"), index=0 ("Index")) -> (array with subset deleted=w668:dbl[])  [unwired: 1 out]
        n94 = case shown="True" w593 {
          tunnel: w642 -> [w699 w702]
          tunnel: w639 -> [_ w701]
          tunnel: [w699 w700] -> w611
          frame False {
          }
          frame True {
            n95 = Build Array (concatenate)(w702, w701) -> (w700:i32[])
          }
        }
        n96 = Bundle By Name(cluster=w675, "Gate Start"=w683, "Gate Stop"=w682, "Gate Step (linear only)"=w681, "Gate Compliance"=w692, "Range mode"=w659, "Range"=w658) -> (w660:T6)
        n97 = Index Array(array=w668, index #1=0 ("Index")) -> (element #1=w678:dbl, element #2=w677:dbl, element #3=w676:dbl)  [unwired: 2 in]
        n98 = call <vilib>:"compatOverwrite.vi"("overwrite (F)"=TRUE) -> ("overwrite?"=w649:T8)
        n99 = Bundle By Name(cluster=w674, "Drain Start"=w678, "Drain Stop"=w677, "Drain Step"=w676, "Drain Compliance"=w693, "Range mode"=w657, "Range"=w656) -> (w661:T7)
        n100 = call "4155C Transfer v3.0.vi"("VISA resource name in"=w663, "Source/Common"=w586, 2:"Gate"=w660, 3:"Drain"=w661, 4:"Drain"=w585, "Timings"=w691, "error in (no error)"=w664, 7:"Probe 4"=w592, 8:"Gate"=w584, 9:"Probe 4"=w583, "sweep mode"=w684, "Panel Controls"=w651, "Standby"=w587) -> ("VG"=w648:dbl[], "Outparams"=w655:T9, "VISA Resource Name out"=w690:refnum<visa-resource-name>, "IS"=w621:dbl[], "ID"=w622:dbl[], "IG"=w620:dbl[], "error out"=w640:errorcluster, "Probe 4"=w652:dbl[])  [unwired: 7 in]
        n101 = Unbundle By Name(w655) -> ("V2 Step"=w654:dbl, "V2 Start"=w653:dbl, "Number of points"=w609:i32)
        n102 = call "4155C Split array.vi"("Number of VAR2 steps"=w609, "Y2 data in"=w622, "X data in"=w648, "Y1 data in"=w621, "Y3 data in"=w620, "error in (no error)"=w640) -> ("Array of clusters"=w641:cluster{"Y data in":dbl[], "X data in":dbl[]}[], "error out"=w597:errorcluster)  [unwired: 1 in]
        n103 = case shown="True" "Plot transfer curve extrema vs time" {
          tunnel: w647 -> [w711 w781]
          tunnel: w638 -> [w712 w776]
          tunnel: w624 -> [w705 w772]
          tunnel: w623 -> [w706 w771]
          tunnel: w622 -> [_ w768]
          tunnel: w621 -> [_ w766]
          tunnel: w620 -> [_ w765]
          tunnel: w619 -> [w713 w761]
          tunnel: w618 -> [w714 w760]
          tunnel: w617 -> [w709 w757]
          tunnel: w616 -> [w710 w756]
          tunnel: w615 -> [w704 w753]
          tunnel: w614 -> [w703 w752]
          tunnel: w613 -> [w708 w749]
          tunnel: w612 -> [w707 w748]
          tunnel: w611 -> [_ w741]
          tunnel: [w709 w736] -> w610
          tunnel: w609 -> [_ w735]
          tunnel: [w710 w734] -> w608
          tunnel: [w711 w733] -> w607
          tunnel: [w712 w732] -> w606
          tunnel: [w713 w731] -> w605
          tunnel: [w714 w730] -> w604
          tunnel: [w708 w729] -> w603
          tunnel: [w707 w728] -> w602
          tunnel: [w706 w727] -> w601
          tunnel: [w705 w726] -> w600
          tunnel: [w704 w725] -> w599
          tunnel: [w703 w724] -> w598
          tunnel: w597 -> [w715 w723]
          tunnel: [w715 w719] -> w596
          frame False {
          }
          frame True {
            # "Adjusts graph colors."
            # "Adjusts graph colors."
            # "Ion will be the middle element of the array. The calculation of the index is done only once, since Is, Id, and Ig have the same dimensions."
            # "abs(Ig)"
            # "abs(Is)"
            # "Y1: Is\nY2: Id\nY3: Ig"
            # "abs(Id)"
            # "Adjusts graph colors."
            # "Adjusts graph colors."
            # "Adjusts graph colors."
            n104 = Absolute Value(x=w766) -> (abs(x)=w751:dbl[])
            n105 = Absolute Value(x=w768) -> (abs(x)=w767:dbl[])
            n106 = Absolute Value(x=w765) -> (abs(x)=w754:dbl[])
            n107 = Array Size(array=w767) -> (size(s)=w775:i32)
            n108 = Divide(x=w775, y=2) -> (x/y=w718:dbl)
            n109 = Subtract(x=w718, y=1) -> (x-y=w717:dbl)
            n110 = Array Max & Min(array=w751) -> (max value=w758:dbl, min value=w759:dbl)  [unwired: 2 out]
            n111 = Array Max & Min(array=w767) -> (max value=w780:dbl, min value=w764:dbl)  [unwired: 2 out]
            n112 = Array Max & Min(array=w754) -> (max value=w763:dbl, min value=w762:dbl)  [unwired: 2 out]
            n113 = Index Array(array=w751, index=w717) -> (element=w742:dbl)
            n114 = Index Array(array=w751, index=0) -> (element=w743:dbl)
            n115 = Index Array(array=w767, index=w717) -> (element=w744:dbl)
            n116 = Index Array(array=w767, index=0) -> (element=w745:dbl)
            n117 = Index Array(array=w754, index=w717) -> (element=w747:dbl)
            n118 = Index Array(array=w754, index=0) -> (element=w746:dbl)
            n119 = local write "Ig max"(w763) -> ()
            n120 = local write "Ig min"(w762) -> ()
            n121 = local write "Is max"(w758) -> ()
            n122 = local write "Is min"(w759) -> ()
            n123 = local write "Id max"(w780) -> ()
            n124 = local write "Id min"(w764) -> ()
            n125 = Build Array (concatenate)(w757, w758) -> (w736:dbl[])
            n126 = Build Array (concatenate)(w756, w759) -> (w734:dbl[])
            n127 = local write "Is off"(w743) -> ()
            n128 = local write "Is on"(w742) -> ()
            n129 = Build Array (concatenate)(w781, w780) -> (w733:dbl[])
            n130 = Build Array (concatenate)(w776, w764) -> (w732:dbl[])
            n131 = Build Array (concatenate)(w761, w763) -> (w731:dbl[])
            n132 = Build Array (concatenate)(w760, w762) -> (w730:dbl[])
            n133 = Build Array (concatenate)(w749, w742) -> (w729:dbl[])
            n134 = Build Array (concatenate)(w748, w743) -> (w728:dbl[])
            n135 = Build Array (concatenate)(w771, w744) -> (w727:dbl[])
            n136 = Build Array (concatenate)(w772, w745) -> (w726:dbl[])
            n137 = Build Array (concatenate)(w753, w747) -> (w725:dbl[])
            n138 = Build Array (concatenate)(w752, w746) -> (w724:dbl[])
            n139 = local write "Ig off"(w746) -> ()
            n140 = local write "Ig on"(w747) -> ()
            n141 = local write "Id off"(w745) -> ()
            n142 = local write "Id on"(w744) -> ()
            n143 = control-ref of="Imax vs time"() -> (w770:refnum<vi>)
            n144 = control-ref of="Imin vs time"() -> (w769:refnum<vi>)
            n145 = control-ref of="Ion vs time"() -> (w738:refnum<vi>)
            n146 = control-ref of="Ioff vs time"() -> (w737:refnum<vi>)
            n147 = control-ref of="I vs Vg"() -> (w779:refnum<vi>)
            n148 = call "4155C Split array.vi"("Number of VAR2 steps"=w735, "Y2 data in"=w727, "X data in"=w741, "Y1 data in"=w729, "Y3 data in"=w725, "error in (no error)"=w723) -> ("Array of clusters"=w739:cluster{"Y data in":dbl[], "X data in":dbl[]}[], "error out"=w722:errorcluster)  [unwired: 1 in]
            n149 = call "4155C Split array.vi"("Number of VAR2 steps"=w735, "Y2 data in"=w726, "X data in"=w741, "Y1 data in"=w728, "Y3 data in"=w724, "error in (no error)"=w722) -> ("Array of clusters"=w740:cluster{"Y data in":dbl[], "X data in":dbl[]}[], "error out"=w721:errorcluster)  [unwired: 1 in]
            n150 = call "4155C Split array.vi"("Number of VAR2 steps"=w735, "Y2 data in"=w733, "X data in"=w741, "Y1 data in"=w736, "Y3 data in"=w731, "error in (no error)"=w721) -> ("Array of clusters"=w778:cluster{"Y data in":dbl[], "X data in":dbl[]}[], "error out"=w720:errorcluster)  [unwired: 1 in]
            n151 = call "4155C Split array.vi"("Number of VAR2 steps"=w735, "Y2 data in"=w732, "X data in"=w741, "Y1 data in"=w734, "Y3 data in"=w730, "error in (no error)"=w720) -> ("Array of clusters"=w777:cluster{"Y data in":dbl[], "X data in":dbl[]}[], "error out"=w719:errorcluster)  [unwired: 1 in]
            n152 = call "4155C Config Chart Colours.vi"("Numeric"=w735, "XY Graph 2"=w770) -> ()  [unwired: 6 in]
            n153 = call "4155C Config Chart Colours.vi"("Numeric"=w735, "XY Graph 2"=w769) -> ()  [unwired: 6 in]
            n154 = call "4155C Config Chart Colours.vi"("Numeric"=w735, "XY Graph 2"=w738) -> ()  [unwired: 6 in]
            n155 = call "4155C Config Chart Colours.vi"("Numeric"=w735, "XY Graph 2"=w737) -> ()  [unwired: 6 in]
            n156 = call "4155C Config Chart Colours.vi"("Numeric"=w735, "XY Graph 2"=w779) -> ()  [unwired: 6 in]
            n157 = local write "Imax vs time"(w778) -> ()
            n158 = local write "Imin vs time"(w777) -> ()
            n159 = local write "Ion vs time"(w739) -> ()
            n160 = local write "Ioff vs time"(w740) -> ()
          }
        }
        n161 = local write "I vs Vg"(w641) -> ()
        n162 = Open/Create/Replace File(file path (use dialog)=w694, error in=w596, operation (0:open)=w649) -> (refnum out=w636:refnum<file>, error out=w634:errorcluster)  [unwired: 3 in, 1 out]
        n163 = call "4155C Make Big 2d array.vi"("1D Var1"=w648, "1d IS"=w621, "1d ID"=w622, "1d IG"=w620, "1d SMU4"=w652, "SMU4"=w592, "VAR2 START"=w653, "Number of VAR2 steps"=w609, "VAR2 STEP"=w654, "VAR1 Name"="Vg", "Decimal places in header"=i8 1, "VAR2 Name"="Vd") -> ("Header array"=w637:string[], "Data array"=w635:dbl[][])  [unwired: 14 in]
        n164 = call "4155C Write array to file.vi"("Byte Stream File Refnum"=w636, "Header"=w637, "Data Array"=w635, "error in (no error)"=w634) -> ("dup refnum"=w633:refnum<file>, "error out"=w632:errorcluster)  [unwired: 1 in]
        n165 = Close File(refnum=w633, error in=w632) -> (error out=w689:errorcluster)  [unwired: 1 out]
      }
      frame "transfer-fpp" {
        # "Adjusts graph colors."
        # "Y1 = Y2 = ID\nY3 = IG"
        n166 = local read "Plot transfer curve extrema vs time"() -> (w798:bool)
        n167 = Number To Decimal String(number=w847) -> (decimal integer string=w894:string)  [unwired: 1 in]
        n168 = Bundle By Name(cluster=w872, "Emergency Stop"=w897) -> (w905:T1)
        n169 = Delete From Array(array=w823, index=0 ("Index")) -> (deleted portion=w885:string, array with subset deleted=w884:string[])  [unwired: 1 in]
        n170 = local read "Plot transfer curve extrema vs time"() -> (w824:bool)
        n171 = local read "FPP - Source"() -> (w835:u32)
        n172 = local read "FPP - Drain"() -> (w833:u32)
        n173 = local read "FPP - Gate"() -> (w834:u32)
        n174 = Concatenate Strings(w893, "-transferfpp-" ("Substring"), w894, w845, ".txt" ("Substring")) -> (w896:string)
        n175 = VISA Write(VISA resource name=w864, write buffer=":PAGE:CHAN:MODE SWE;" ("write buffer (\"\")"), error in (no error)=w863) -> (VISA resource name out=w861:refnum<visa-resource-name>, error out=w862:errorcluster)  [unwired: 1 out]
        n176 = case shown="\"d\", Default" w885 {
          tunnel: [w989 w990] -> w883
          frame "s" {
            w989 = u16 0 items=["Single", "Double"] ("sweep mode")
          }
          frame "d", Default {
            w990 = u16 1 items=["Single", "Double"] ("sweep mode")
          }
        }
        n177 = Fract/Exp String To Number(string=w884) -> (number=w868:dbl[])  [unwired: 3 in, 1 out]
        n178 = String To Path(string=w896) -> (path=w892:path)
        n179 = Index Array(array=w868, index #1=0 ("Index")) -> (element #1=w882:dbl, element #2=w881:dbl, element #3=w880:dbl)  [unwired: 2 in]
        n180 = Delete From Array(array=w868, length=3 ("Length"), index=0 ("Index")) -> (array with subset deleted=w866:dbl[])  [unwired: 1 out]
        n181 = local read "FPP - Probe 2"() -> (w831:u32)
        n182 = local read "FPP - Probe 1"() -> (w832:u32)
        n183 = case shown="True" w824 {
          tunnel: w825 -> [w985 w988]
          tunnel: w826 -> [_ w987]
          tunnel: [w985 w986] -> w786
          frame False {
          }
          frame True {
            n184 = Build Array (concatenate)(w988, w987) -> (w986:i32[])
          }
        }
        n185 = control-ref of="I vs Vg"() -> (w827:refnum<vi>)
        n186 = Bundle By Name(cluster=w874, "Gate Start"=w882, "Gate Stop"=w881, "Gate Step (linear only)"=w880, "Gate Compliance"=w890, "Range mode"=w857, "Range"=w856) -> (w858:T6)
        n187 = Index Array(array=w866, index #1=0 ("Index")) -> (element #1=w877:dbl, element #2=w876:dbl, element #3=w875:dbl)  [unwired: 2 in]
        n188 = call <vilib>:"compatOverwrite.vi"("overwrite (F)"=TRUE) -> ("overwrite?"=w848:T8)
        n189 = Bundle By Name(cluster=w873, "Drain Start"=w877, "Drain Stop"=w876, "Drain Step"=w875, "Drain Compliance"=w891, "Range mode"=w855, "Range"=w854) -> (w859:T7)
        n190 = call "4155C Transfer-FPP v3.0.vi"("VISA resource name in"=w861, "FPP - Source"=w835, "Gate"=w858, "Drain"=w859, "FPP - Drain"=w833, "Timings"=w889, "error in (no error)"=w862, "FPP - Gate"=w834, "FPP - Probe 1"=w832, "sweep mode"=w883, "FPP - Probe 2"=w831, "Panel Controls"=w905) -> ("VG"=w828:dbl[], "Outparams"=w853:T9, "VISA Resource Name out"=w888:refnum<visa-resource-name>, "Vprobe2"=w850:dbl[], "ID"=w784:dbl[], "IG"=w785:dbl[], "Vprobe1"=w849:dbl[], "error out"=w789:errorcluster)  [unwired: 8 in]
        n191 = Unbundle By Name(w853) -> ("V2 Step"=w852:dbl, "V2 Start"=w851:dbl, "Number of points"=w787:i32)
        n192 = case shown="True" w798 {
          tunnel: w814 -> [w914 w984]
          tunnel: w813 -> [w915 w979]
          tunnel: w819 -> [w908 w975]
          tunnel: w820 -> [w909 w974]
          tunnel: w784 -> [_ w971]
          tunnel: w784 -> [_ w969]
          tunnel: w785 -> [_ w968]
          tunnel: w812 -> [w916 w964]
          tunnel: w811 -> [w917 w963]
          tunnel: w816 -> [w912 w960]
          tunnel: w815 -> [w913 w959]
          tunnel: w818 -> [w907 w956]
          tunnel: w817 -> [w906 w955]
          tunnel: w822 -> [w911 w952]
          tunnel: w821 -> [w910 w951]
          tunnel: w786 -> [_ w944]
          tunnel: [w912 w939] -> w805
          tunnel: w787 -> [_ w938]
          tunnel: [w913 w937] -> w806
          tunnel: [w914 w936] -> w807
          tunnel: [w915 w935] -> w808
          tunnel: [w916 w934] -> w809
          tunnel: [w917 w933] -> w810
          tunnel: [w911 w932] -> w799
          tunnel: [w910 w931] -> w800
          tunnel: [w909 w930] -> w801
          tunnel: [w908 w929] -> w802
          tunnel: [w907 w928] -> w804
          tunnel: [w906 w927] -> w803
          tunnel: w789 -> [w918 w926]
          tunnel: [w918 w922] -> w788
          frame False {
          }
          frame True {
            # "Y1 = Y2 = ID\nY3 = IG"
            # "Adjusts graph colors."
            # "Adjusts graph colors."
            # "Ion will be the middle element of the array. The calculation of the index is done only once, since Is, Id, and Ig have the same dimensions."
            # "abs(Ig)"
            # "abs(Is)"
            # "abs(Id)"
            # "Adjusts graph colors."
            # "Adjusts graph colors."
            # "Adjusts graph colors."
            n193 = Absolute Value(x=w969) -> (abs(x)=w954:dbl[])
            n194 = Absolute Value(x=w971) -> (abs(x)=w970:dbl[])
            n195 = Absolute Value(x=w968) -> (abs(x)=w957:dbl[])
            n196 = Array Size(array=w970) -> (size(s)=w978:i32)
            n197 = Divide(x=w978, y=2) -> (x/y=w921:dbl)
            n198 = Subtract(x=w921, y=1) -> (x-y=w920:dbl)
            n199 = Array Max & Min(array=w954) -> (max value=w961:dbl, min value=w962:dbl)  [unwired: 2 out]
            n200 = Array Max & Min(array=w970) -> (max value=w983:dbl, min value=w967:dbl)  [unwired: 2 out]
            n201 = Array Max & Min(array=w957) -> (max value=w966:dbl, min value=w965:dbl)  [unwired: 2 out]
            n202 = Index Array(array=w954, index=w920) -> (element=w945:dbl)
            n203 = Index Array(array=w954, index=0) -> (element=w946:dbl)
            n204 = Index Array(array=w970, index=w920) -> (element=w947:dbl)
            n205 = Index Array(array=w970, index=0) -> (element=w948:dbl)
            n206 = Index Array(array=w957, index=w920) -> (element=w950:dbl)
            n207 = Index Array(array=w957, index=0) -> (element=w949:dbl)
            n208 = local write "Ig max"(w966) -> ()
            n209 = local write "Ig min"(w965) -> ()
            n210 = local write "Is max"(w961) -> ()
            n211 = local write "Is min"(w962) -> ()
            n212 = local write "Id max"(w983) -> ()
            n213 = local write "Id min"(w967) -> ()
            n214 = Build Array (concatenate)(w960, w961) -> (w939:dbl[])
            n215 = Build Array (concatenate)(w959, w962) -> (w937:dbl[])
            n216 = local write "Is off"(w946) -> ()
            n217 = local write "Is on"(w945) -> ()
            n218 = Build Array (concatenate)(w984, w983) -> (w936:dbl[])
            n219 = Build Array (concatenate)(w979, w967) -> (w935:dbl[])
            n220 = Build Array (concatenate)(w964, w966) -> (w934:dbl[])
            n221 = Build Array (concatenate)(w963, w965) -> (w933:dbl[])
            n222 = Build Array (concatenate)(w952, w945) -> (w932:dbl[])
            n223 = Build Array (concatenate)(w951, w946) -> (w931:dbl[])
            n224 = Build Array (concatenate)(w974, w947) -> (w930:dbl[])
            n225 = Build Array (concatenate)(w975, w948) -> (w929:dbl[])
            n226 = Build Array (concatenate)(w956, w950) -> (w928:dbl[])
            n227 = Build Array (concatenate)(w955, w949) -> (w927:dbl[])
            n228 = local write "Ig off"(w949) -> ()
            n229 = local write "Ig on"(w950) -> ()
            n230 = local write "Id off"(w948) -> ()
            n231 = local write "Id on"(w947) -> ()
            n232 = control-ref of="Imax vs time"() -> (w973:refnum<vi>)
            n233 = control-ref of="Imin vs time"() -> (w972:refnum<vi>)
            n234 = control-ref of="Ion vs time"() -> (w941:refnum<vi>)
            n235 = control-ref of="Ioff vs time"() -> (w940:refnum<vi>)
            n236 = control-ref of="I vs Vg"() -> (w982:refnum<vi>)
            n237 = call "4155C Split array.vi"("Number of VAR2 steps"=w938, "Y2 data in"=w930, "X data in"=w944, "Y1 data in"=w932, "Y3 data in"=w928, "error in (no error)"=w926) -> ("Array of clusters"=w942:cluster{"Y data in":dbl[], "X data in":dbl[]}[], "error out"=w925:errorcluster)  [unwired: 1 in]
            n238 = call "4155C Split array.vi"("Number of VAR2 steps"=w938, "Y2 data in"=w929, "X data in"=w944, "Y1 data in"=w931, "Y3 data in"=w927, "error in (no error)"=w925) -> ("Array of clusters"=w943:cluster{"Y data in":dbl[], "X data in":dbl[]}[], "error out"=w924:errorcluster)  [unwired: 1 in]
            n239 = call "4155C Split array.vi"("Number of VAR2 steps"=w938, "Y2 data in"=w936, "X data in"=w944, "Y1 data in"=w939, "Y3 data in"=w934, "error in (no error)"=w924) -> ("Array of clusters"=w981:cluster{"Y data in":dbl[], "X data in":dbl[]}[], "error out"=w923:errorcluster)  [unwired: 1 in]
            n240 = call "4155C Split array.vi"("Number of VAR2 steps"=w938, "Y2 data in"=w935, "X data in"=w944, "Y1 data in"=w937, "Y3 data in"=w933, "error in (no error)"=w923) -> ("Array of clusters"=w980:cluster{"Y data in":dbl[], "X data in":dbl[]}[], "error out"=w922:errorcluster)  [unwired: 1 in]
            n241 = call "4155C Config Chart Colours.vi"("Numeric"=w938, "XY Graph 2"=w973) -> ()  [unwired: 6 in]
            n242 = call "4155C Config Chart Colours.vi"("Numeric"=w938, "XY Graph 2"=w972) -> ()  [unwired: 6 in]
            n243 = call "4155C Config Chart Colours.vi"("Numeric"=w938, "XY Graph 2"=w941) -> ()  [unwired: 6 in]
            n244 = call "4155C Config Chart Colours.vi"("Numeric"=w938, "XY Graph 2"=w940) -> ()  [unwired: 6 in]
            n245 = call "4155C Config Chart Colours.vi"("Numeric"=w938, "XY Graph 2"=w982) -> ()  [unwired: 6 in]
            n246 = local write "Imax vs time"(w981) -> ()
            n247 = local write "Imin vs time"(w980) -> ()
            n248 = local write "Ion vs time"(w942) -> ()
            n249 = local write "Ioff vs time"(w943) -> ()
          }
        }
        n250 = call "4155C Split array.vi"("Number of VAR2 steps"=w787, "Y2 data in"=w784, "X data in"=w828, "Y1 data in"=w784, "Y3 data in"=w785, "error in (no error)"=w788) -> ("Array of clusters"=w830:cluster{"Y data in":dbl[], "X data in":dbl[]}[], "error out"=w829:errorcluster)  [unwired: 1 in]
        n251 = local write "I vs Vg"(w830) -> ()
        n252 = call "4155C Config Chart Colours.vi"("Numeric"=w787, "XY Graph 2"=w827) -> ()  [unwired: 6 in]
        n253 = Open/Create/Replace File(file path (use dialog)=w892, error in=w829, operation (0:open)=w848) -> (refnum out=w902:refnum<file>, error out=w903:errorcluster)  [unwired: 3 in, 1 out]
        n254 = call "4155C Make Big 2d array FPP.vi"("1D Var1"=w828, "1d ID"=w784, "1d Vp2"=w850, "1d IG"=w785, "1d Vp1"=w849, "VAR2 START"=w851, "Number of VAR2 steps"=w787, "VAR2 STEP"=w852, "VAR1 Name"="Vg", "Decimal places in header"=i8 1, "VAR2 Name"="Vd") -> ("Header array"=w898:string[], "Data array"=w899:dbl[][])  [unwired: 15 in]
        n255 = call "4155C Write array to file.vi"("Byte Stream File Refnum"=w902, "Header"=w898, "Data Array"=w899, "error in (no error)"=w903) -> ("dup refnum"=w900:refnum<file>, "error out"=w901:errorcluster)  [unwired: 1 in]
        n256 = Close File(refnum=w900, error in=w901) -> (error out=w887:errorcluster)  [unwired: 1 out]
      }
      frame "output" {
        n257 = local read "Transfer/Output - Probe 4"() -> (w995:u32)
        n258 = Delete From Array(array=w1100, index=0 ("Index")) -> (deleted portion=w1098:string, array with subset deleted=w1097:string[])  [unwired: 1 in]
        n259 = Bundle By Name(cluster=w1007, "Emergency Stop"=w1109) -> (w1063:T1)
        n260 = Number To Decimal String(number=w1059) -> (decimal integer string=w1058:string)  [unwired: 1 in]
        n261 = case shown="\"d\", Default" w1098 {
          tunnel: [w1194 w1195] -> w1096
          frame "s" {
            w1194 = u16 0 items=["Single", "Double"] ("sweep mode")
          }
          frame "d", Default {
            w1195 = u16 1 items=["Single", "Double"] ("sweep mode")
          }
        }
        n262 = Fract/Exp String To Number(string=w1097) -> (number=w1082:dbl[])  [unwired: 3 in, 1 out]
        n263 = Concatenate Strings(w1107, w1008, w1058, w1056, "_O_1_C_L.txt" ("Suffix (transfer)")) -> (w1108:string)
        n264 = local read "Transfer/Output - Drain"() -> (w997:u32)
        n265 = local read "Transfer/Output - Source/Common"() -> (w998:u32)
        n266 = VISA Write(VISA resource name=w1078, write buffer=":PAGE:CHAN:MODE SWE;" ("write buffer (\"\")"), error in (no error)=w1077) -> (VISA resource name out=w1075:refnum<visa-resource-name>, error out=w1076:errorcluster)  [unwired: 1 out]
        n267 = String To Path(string=w1108) -> (path=w1106:path)
        n268 = local read "Plot output curve extrema vs time"() -> (w1005:bool)
        n269 = Index Array(array=w1082, index #1=0 ("Index")) -> (element #1=w1095:dbl, element #2=w1094:dbl, element #3=w1093:dbl)  [unwired: 2 in]
        n270 = Delete From Array(array=w1082, length=3 ("Length"), index=0 ("Index")) -> (array with subset deleted=w1080:dbl[])  [unwired: 1 out]
        n271 = local read "Transfer/Output - Gate"() -> (w996:u32)
        n272 = case shown="True" w1005 {
          tunnel: w1055 -> [w1111 w1114]
          tunnel: w1052 -> [_ w1113]
          tunnel: [w1111 w1112] -> w1024
          frame False {
          }
          frame True {
            n273 = Build Array (concatenate)(w1114, w1113) -> (w1112:i32[])
          }
        }
        n274 = Bundle By Name(cluster=w1087, "Gate Start"=w1095, "Gate Stop"=w1094, "Gate Step (linear only)"=w1093, "Gate Compliance"=w1104, "Range mode"=w1071, "Range"=w1070) -> (w1072:T6)
        n275 = Index Array(array=w1080, index #1=0 ("Index")) -> (element #1=w1090:dbl, element #2=w1089:dbl, element #3=w1088:dbl)  [unwired: 2 in]
        n276 = call <vilib>:"compatOverwrite.vi"("overwrite (F)"=TRUE) -> ("overwrite?"=w1062:T8)
        n277 = Bundle By Name(cluster=w1086, "Drain Start"=w1090, "Drain Stop"=w1089, "Drain Step"=w1088, "Drain Compliance"=w1105, "Range mode"=w1069, "Range"=w1068) -> (w1073:T7)
        n278 = call "4155C Output v3.0.vi"("VISA resource name in"=w1075, "Source/Common"=w998, 2:"Gate"=w1072, 3:"Drain"=w1073, 4:"Drain"=w997, "Timings"=w1103, "error in (no error)"=w1076, 7:"Probe 4"=w1004, 8:"Gate"=w996, 9:"Probe 4"=w995, "sweep mode"=w1096, "Panel controls"=w1063, "Standby"=w999) -> ("VD"=w1061:dbl[], "Outparams"=w1067:T9, "VISA Resource Name out"=w1102:refnum<visa-resource-name>, "IS"=w1034:dbl[], "ID"=w1035:dbl[], "IG"=w1033:dbl[], "error out"=w1053:errorcluster, "Probe 4"=w1064:dbl[])  [unwired: 7 in]
        n279 = Unbundle By Name(w1067) -> ("V2 Step"=w1066:dbl, "V2 Start"=w1065:dbl, "Number of points"=w1022:i32)
        n280 = call "4155C Split array.vi"("Number of VAR2 steps"=w1022, "Y2 data in"=w1035, "X data in"=w1061, "Y1 data in"=w1034, "Y3 data in"=w1033, "error in (no error)"=w1053) -> ("Array of clusters"=w1054:cluster{"Y data in":dbl[], "X data in":dbl[]}[], "error out"=w1010:errorcluster)  [unwired: 1 in]
        n281 = case shown="True" "Plot output curve extrema vs time" {
          tunnel: w1060 -> [w1118 w1193]
          tunnel: w1051 -> [w1117 w1188]
          tunnel: w1037 -> [w1123 w1184]
          tunnel: w1036 -> [w1124 w1183]
          tunnel: w1035 -> [_ w1180]
          tunnel: w1034 -> [_ w1178]
          tunnel: w1033 -> [_ w1177]
          tunnel: w1032 -> [w1116 w1173]
          tunnel: w1031 -> [w1115 w1172]
          tunnel: w1030 -> [w1120 w1169]
          tunnel: w1029 -> [w1119 w1168]
          tunnel: w1028 -> [w1122 w1165]
          tunnel: w1027 -> [w1121 w1164]
          tunnel: w1026 -> [w1126 w1161]
          tunnel: w1025 -> [w1125 w1160]
          tunnel: w1024 -> [_ w1153]
          tunnel: [w1120 w1148] -> w1023
          tunnel: w1022 -> [_ w1147]
          tunnel: [w1119 w1146] -> w1021
          tunnel: [w1118 w1145] -> w1020
          tunnel: [w1117 w1144] -> w1019
          tunnel: [w1116 w1143] -> w1018
          tunnel: [w1115 w1142] -> w1017
          tunnel: [w1126 w1141] -> w1016
          tunnel: [w1125 w1140] -> w1015
          tunnel: [w1124 w1139] -> w1014
          tunnel: [w1123 w1138] -> w1013
          tunnel: [w1122 w1137] -> w1012
          tunnel: [w1121 w1136] -> w1011
          tunnel: w1010 -> [w1127 w1135]
          tunnel: [w1127 w1131] -> w1009
          frame False {
          }
          frame True {
            # "Adjusts graph colors."
            # "Adjusts graph colors."
            # "Ion will be the middle element of the array. The calculation of the index is done only once, since Is, Id, and Ig have the same dimensions."
            # "abs(Ig)"
            # "abs(Is)"
            # "Y1: Is\nY2: Id\nY3: Ig"
            # "abs(Id)"
            # "Adjusts graph colors."
            # "Adjusts graph colors."
            # "Adjusts graph colors."
            n282 = Absolute Value(x=w1178) -> (abs(x)=w1163:dbl[])
            n283 = Absolute Value(x=w1180) -> (abs(x)=w1179:dbl[])
            n284 = Absolute Value(x=w1177) -> (abs(x)=w1166:dbl[])
            n285 = Array Size(array=w1179) -> (size(s)=w1187:i32)
            n286 = Divide(x=w1187, y=2) -> (x/y=w1130:dbl)
            n287 = Subtract(x=w1130, y=1) -> (x-y=w1129:dbl)
            n288 = Array Max & Min(array=w1163) -> (max value=w1170:dbl, min value=w1171:dbl)  [unwired: 2 out]
            n289 = Array Max & Min(array=w1179) -> (max value=w1192:dbl, min value=w1176:dbl)  [unwired: 2 out]
            n290 = Array Max & Min(array=w1166) -> (max value=w1175:dbl, min value=w1174:dbl)  [unwired: 2 out]
            n291 = Index Array(array=w1163, index=w1129) -> (element=w1154:dbl)
            n292 = Index Array(array=w1163, index=0) -> (element=w1155:dbl)
            n293 = Index Array(array=w1179, index=w1129) -> (element=w1156:dbl)
            n294 = Index Array(array=w1179, index=0) -> (element=w1157:dbl)
            n295 = Index Array(array=w1166, index=w1129) -> (element=w1159:dbl)
            n296 = Index Array(array=w1166, index=0) -> (element=w1158:dbl)
            n297 = local write "Ig max"(w1175) -> ()
            n298 = local write "Ig min"(w1174) -> ()
            n299 = local write "Is max"(w1170) -> ()
            n300 = local write "Is min"(w1171) -> ()
            n301 = local write "Id max"(w1192) -> ()
            n302 = local write "Id min"(w1176) -> ()
            n303 = Build Array (concatenate)(w1169, w1170) -> (w1148:dbl[])
            n304 = Build Array (concatenate)(w1168, w1171) -> (w1146:dbl[])
            n305 = local write "Is off"(w1155) -> ()
            n306 = local write "Is on"(w1154) -> ()
            n307 = Build Array (concatenate)(w1193, w1192) -> (w1145:dbl[])
            n308 = Build Array (concatenate)(w1188, w1176) -> (w1144:dbl[])
            n309 = Build Array (concatenate)(w1173, w1175) -> (w1143:dbl[])
            n310 = Build Array (concatenate)(w1172, w1174) -> (w1142:dbl[])
            n311 = Build Array (concatenate)(w1161, w1154) -> (w1141:dbl[])
            n312 = Build Array (concatenate)(w1160, w1155) -> (w1140:dbl[])
            n313 = Build Array (concatenate)(w1183, w1156) -> (w1139:dbl[])
            n314 = Build Array (concatenate)(w1184, w1157) -> (w1138:dbl[])
            n315 = Build Array (concatenate)(w1165, w1159) -> (w1137:dbl[])
            n316 = Build Array (concatenate)(w1164, w1158) -> (w1136:dbl[])
            n317 = local write "Ig off"(w1158) -> ()
            n318 = local write "Ig on"(w1159) -> ()
            n319 = local write "Id off"(w1157) -> ()
            n320 = local write "Id on"(w1156) -> ()
            n321 = control-ref of="Imax vs time"() -> (w1182:refnum<vi>)
            n322 = control-ref of="Imin vs time"() -> (w1181:refnum<vi>)
            n323 = control-ref of="Ion vs time"() -> (w1150:refnum<vi>)
            n324 = control-ref of="Ioff vs time"() -> (w1149:refnum<vi>)
            n325 = control-ref of="I vs Vg"() -> (w1191:refnum<vi>)
            n326 = call "4155C Split array.vi"("Number of VAR2 steps"=w1147, "Y2 data in"=w1139, "X data in"=w1153, "Y1 data in"=w1141, "Y3 data in"=w1137, "error in (no error)"=w1135) -> ("Array of clusters"=w1151:cluster{"Y data in":dbl[], "X data in":dbl[]}[], "error out"=w1134:errorcluster)  [unwired: 1 in]
            n327 = call "4155C Split array.vi"("Number of VAR2 steps"=w1147, "Y2 data in"=w1138, "X data in"=w1153, "Y1 data in"=w1140, "Y3 data in"=w1136, "error in (no error)"=w1134) -> ("Array of clusters"=w1152:cluster{"Y data in":dbl[], "X data in":dbl[]}[], "error out"=w1133:errorcluster)  [unwired: 1 in]
            n328 = call "4155C Split array.vi"("Number of VAR2 steps"=w1147, "Y2 data in"=w1145, "X data in"=w1153, "Y1 data in"=w1148, "Y3 data in"=w1143, "error in (no error)"=w1133) -> ("Array of clusters"=w1190:cluster{"Y data in":dbl[], "X data in":dbl[]}[], "error out"=w1132:errorcluster)  [unwired: 1 in]
            n329 = call "4155C Split array.vi"("Number of VAR2 steps"=w1147, "Y2 data in"=w1144, "X data in"=w1153, "Y1 data in"=w1146, "Y3 data in"=w1142, "error in (no error)"=w1132) -> ("Array of clusters"=w1189:cluster{"Y data in":dbl[], "X data in":dbl[]}[], "error out"=w1131:errorcluster)  [unwired: 1 in]
            n330 = call "4155C Config Chart Colours.vi"("Numeric"=w1147, "XY Graph 2"=w1182) -> ()  [unwired: 6 in]
            n331 = call "4155C Config Chart Colours.vi"("Numeric"=w1147, "XY Graph 2"=w1181) -> ()  [unwired: 6 in]
            n332 = call "4155C Config Chart Colours.vi"("Numeric"=w1147, "XY Graph 2"=w1150) -> ()  [unwired: 6 in]
            n333 = call "4155C Config Chart Colours.vi"("Numeric"=w1147, "XY Graph 2"=w1149) -> ()  [unwired: 6 in]
            n334 = call "4155C Config Chart Colours.vi"("Numeric"=w1147, "XY Graph 2"=w1191) -> ()  [unwired: 6 in]
            n335 = local write "Imax vs time"(w1190) -> ()
            n336 = local write "Imin vs time"(w1189) -> ()
            n337 = local write "Ion vs time"(w1151) -> ()
            n338 = local write "Ioff vs time"(w1152) -> ()
          }
        }
        n339 = local write "I vs Vd"(w1054) -> ()
        n340 = Open/Create/Replace File(file path (use dialog)=w1106, error in=w1009, operation (0:open)=w1062) -> (refnum out=w1049:refnum<file>, error out=w1047:errorcluster)  [unwired: 3 in, 1 out]
        n341 = call "4155C Make Big 2d array.vi"("1D Var1"=w1061, "1d IS"=w1034, "1d ID"=w1035, "1d IG"=w1033, "1d SMU4"=w1064, "SMU4"=w1004, "VAR2 START"=w1065, "Number of VAR2 steps"=w1022, "VAR2 STEP"=w1066, "VAR1 Name"="Vd", "Decimal places in header"=i8 1, "VAR2 Name"="Vg") -> ("Header array"=w1050:string[], "Data array"=w1048:dbl[][])  [unwired: 14 in]
        n342 = call "4155C Write array to file.vi"("Byte Stream File Refnum"=w1049, "Header"=w1050, "Data Array"=w1048, "error in (no error)"=w1047) -> ("dup refnum"=w1046:refnum<file>, "error out"=w1045:errorcluster)  [unwired: 1 in]
        n343 = Close File(refnum=w1046, error in=w1045) -> (error out=w1101:errorcluster)  [unwired: 1 out]
      }
      frame "output-fpp" {
        # "Y1 = Y2 = ID\nY3 = IG"
        # "Adjusts graph colors."
        # "Adjusts graph colors."
        # "Y1 = Vp2\nY2 = Y3 = Vp1"
        n344 = local read "Plot output curve extrema vs time"() -> (w1212:bool)
        n345 = local read "FPP - Gate"() -> (w1250:u32)
        n346 = local read "FPP - Probe 1"() -> (w1249:u32)
        n347 = local read "FPP - Probe 2"() -> (w1248:u32)
        n348 = Number To Decimal String(number=w1263) -> (decimal integer string=w1307:string)  [unwired: 1 in]
        n349 = Bundle By Name(cluster=w1285, "Emergency Stop"=w1310) -> (w1320:T1)
        n350 = local read "Plot output curve extrema vs time"() -> (w1237:bool)
        n351 = Delete From Array(array=w1236, index=0 ("Index")) -> (deleted portion=w1298:string, array with subset deleted=w1297:string[])  [unwired: 1 in]
        n352 = VISA Write(VISA resource name=w1276, write buffer=":PAGE:CHAN:MODE SWE;" ("write buffer (\"\")"), error in (no error)=w1273) -> (VISA resource name out=w1275:refnum<visa-resource-name>, error out=w1274:errorcluster)  [unwired: 1 out]
        n353 = Concatenate Strings(w1306, "-outputfpp-" ("Substring"), w1307, w1262, ".txt" ("Substring")) -> (w1309:string)
        n354 = case shown="\"d\", Default" w1298 {
          tunnel: [w1404 w1405] -> w1296
          frame "s" {
            w1404 = u16 0 items=["Single", "Double"] ("sweep mode")
          }
          frame "d", Default {
            w1405 = u16 1 items=["Single", "Double"] ("sweep mode")
          }
        }
        n355 = Fract/Exp String To Number(string=w1297) -> (number=w1279:dbl[])  [unwired: 3 in, 1 out]
        n356 = String To Path(string=w1309) -> (path=w1305:path)
        n357 = Index Array(array=w1279, index #1=0 ("Index")) -> (element #1=w1295:dbl, element #2=w1294:dbl, element #3=w1293:dbl)  [unwired: 2 in]
        n358 = Delete From Array(array=w1279, length=3 ("Length"), index=0 ("Index")) -> (array with subset deleted=w1278:dbl[])  [unwired: 1 out]
        n359 = local read "FPP - Source"() -> (w1252:u32)
        n360 = case shown="True" w1237 {
          tunnel: w1238 -> [w1400 w1403]
          tunnel: w1239 -> [_ w1402]
          tunnel: [w1400 w1401] -> w1199
          frame False {
          }
          frame True {
            n361 = Build Array (concatenate)(w1403, w1402) -> (w1401:i32[])
          }
        }
        n362 = local read "FPP - Drain"() -> (w1251:u32)
        n363 = Bundle By Name(cluster=w1287, "Gate Start"=w1295, "Gate Stop"=w1294, "Gate Step (linear only)"=w1293, "Gate Compliance"=w1303, "Range mode"=w1271, "Range"=w1270) -> (w1319:T6)
        n364 = Index Array(array=w1278, index #1=0 ("Index")) -> (element #1=w1290:dbl, element #2=w1289:dbl, element #3=w1288:dbl)  [unwired: 2 in]
        n365 = call <vilib>:"compatOverwrite.vi"("overwrite (F)"=TRUE) -> ("overwrite?"=w1265:T8)
        n366 = control-ref of="I vs Vd"() -> (w1241:refnum<vi>)
        n367 = control-ref of="Vp vs Vg (FPP)"() -> (w1240:refnum<vi>)
        n368 = Bundle By Name(cluster=w1286, "Drain Start"=w1290, "Drain Stop"=w1289, "Drain Step"=w1288, "Drain Compliance"=w1304, "Range mode"=w1269, "Range"=w1272) -> (w1318:T7)
        n369 = call "4155C Output-FPP v3.0.vi"("VISA resource name in"=w1275, "FPP - Source"=w1252, "Gate"=w1319, "Drain"=w1318, "FPP - Drain"=w1251, "Timings"=w1302, "error in (no error)"=w1274, "FPP - Gate"=w1250, "FPP - Probe 1"=w1249, "sweep mode"=w1296, "FPP - Probe 2"=w1248, "Panel controls"=w1320) -> ("VD"=w1244:dbl[], "Outparams"=w1267:T9, "VISA Resource Name out"=w1301:refnum<visa-resource-name>, "Vprobe2"=w1243:dbl[], "ID"=w1198:dbl[], "IG"=w1197:dbl[], "Vprobe1"=w1242:dbl[], "error out"=w1211:errorcluster)  [unwired: 8 in]
        n370 = Unbundle By Name(w1267) -> ("V2 Step"=w1268:dbl, "V2 Start"=w1266:dbl, "Number of points"=w1200:i32)
        n371 = case shown="True" w1212 {
          tunnel: w1196 -> [w1324 w1399]
          tunnel: w1229 -> [w1323 w1394]
          tunnel: w1219 -> [w1329 w1390]
          tunnel: w1220 -> [w1330 w1389]
          tunnel: w1198 -> [_ w1386]
          tunnel: w1198 -> [_ w1384]
          tunnel: w1197 -> [_ w1383]
          tunnel: w1235 -> [w1322 w1379]
          tunnel: w1234 -> [w1321 w1378]
          tunnel: w1227 -> [w1326 w1375]
          tunnel: w1228 -> [w1325 w1374]
          tunnel: w1221 -> [w1328 w1371]
          tunnel: w1222 -> [w1327 w1370]
          tunnel: w1217 -> [w1332 w1367]
          tunnel: w1218 -> [w1331 w1366]
          tunnel: w1199 -> [_ w1359]
          tunnel: [w1326 w1354] -> w1226
          tunnel: w1200 -> [_ w1353]
          tunnel: [w1325 w1352] -> w1225
          tunnel: [w1324 w1351] -> w1230
          tunnel: [w1323 w1350] -> w1231
          tunnel: [w1322 w1349] -> w1232
          tunnel: [w1321 w1348] -> w1233
          tunnel: [w1332 w1347] -> w1213
          tunnel: [w1331 w1346] -> w1214
          tunnel: [w1330 w1345] -> w1215
          tunnel: [w1329 w1344] -> w1216
          tunnel: [w1328 w1343] -> w1224
          tunnel: [w1327 w1342] -> w1223
          tunnel: w1211 -> [w1333 w1341]
          tunnel: [w1333 w1337] -> w1210
          frame False {
          }
          frame True {
            # "Y1 = Y2 = ID\nY3 = IG"
            # "Adjusts graph colors."
            # "Adjusts graph colors."
            # "Ion will be the middle element of the array. The calculation of the index is done only once, since Is, Id, and Ig have the same dimensions."
            # "abs(Ig)"
            # "abs(Is)"
            # "abs(Id)"
            # "Adjusts graph colors."
            # "Adjusts graph colors."
            # "Adjusts graph colors."
            n372 = Absolute Value(x=w1384) -> (abs(x)=w1369:dbl[])
            n373 = Absolute Value(x=w1386) -> (abs(x)=w1385:dbl[])
            n374 = Absolute Value(x=w1383) -> (abs(x)=w1372:dbl[])
            n375 = Array Size(array=w1385) -> (size(s)=w1393:i32)
            n376 = Divide(x=w1393, y=2) -> (x/y=w1336:dbl)
            n377 = Subtract(x=w1336, y=1) -> (x-y=w1335:dbl)
            n378 = Array Max & Min(array=w1369) -> (max value=w1376:dbl, min value=w1377:dbl)  [unwired: 2 out]
            n379 = Array Max & Min(array=w1385) -> (max value=w1398:dbl, min value=w1382:dbl)  [unwired: 2 out]
            n380 = Array Max & Min(array=w1372) -> (max value=w1381:dbl, min value=w1380:dbl)  [unwired: 2 out]
            n381 = Index Array(array=w1369, index=w1335) -> (element=w1360:dbl)
            n382 = Index Array(array=w1369, index=0) -> (element=w1361:dbl)
            n383 = Index Array(array=w1385, index=w1335) -> (element=w1362:dbl)
            n384 = Index Array(array=w1385, index=0) -> (element=w1363:dbl)
            n385 = Index Array(array=w1372, index=w1335) -> (element=w1365:dbl)
            n386 = Index Array(array=w1372, index=0) -> (element=w1364:dbl)
            n387 = local write "Ig max"(w1381) -> ()
            n388 = local write "Ig min"(w1380) -> ()
            n389 = local write "Is max"(w1376) -> ()
            n390 = local write "Is min"(w1377) -> ()
            n391 = local write "Id max"(w1398) -> ()
            n392 = local write "Id min"(w1382) -> ()
            n393 = Build Array (concatenate)(w1375, w1376) -> (w1354:dbl[])
            n394 = Build Array (concatenate)(w1374, w1377) -> (w1352:dbl[])
            n395 = local write "Is off"(w1361) -> ()
            n396 = local write "Is on"(w1360) -> ()
            n397 = Build Array (concatenate)(w1399, w1398) -> (w1351:dbl[])
            n398 = Build Array (concatenate)(w1394, w1382) -> (w1350:dbl[])
            n399 = Build Array (concatenate)(w1379, w1381) -> (w1349:dbl[])
            n400 = Build Array (concatenate)(w1378, w1380) -> (w1348:dbl[])
            n401 = Build Array (concatenate)(w1367, w1360) -> (w1347:dbl[])
            n402 = Build Array (concatenate)(w1366, w1361) -> (w1346:dbl[])
            n403 = Build Array (concatenate)(w1389, w1362) -> (w1345:dbl[])
            n404 = Build Array (concatenate)(w1390, w1363) -> (w1344:dbl[])
            n405 = Build Array (concatenate)(w1371, w1365) -> (w1343:dbl[])
            n406 = Build Array (concatenate)(w1370, w1364) -> (w1342:dbl[])
            n407 = local write "Ig off"(w1364) -> ()
            n408 = local write "Ig on"(w1365) -> ()
            n409 = local write "Id off"(w1363) -> ()
            n410 = local write "Id on"(w1362) -> ()
            n411 = control-ref of="Imax vs time"() -> (w1388:refnum<vi>)
            n412 = control-ref of="Imin vs time"() -> (w1387:refnum<vi>)
            n413 = control-ref of="Ion vs time"() -> (w1356:refnum<vi>)
            n414 = control-ref of="Ioff vs time"() -> (w1355:refnum<vi>)
            n415 = control-ref of="I vs Vg"() -> (w1397:refnum<vi>)
            n416 = call "4155C Split array.vi"("Number of VAR2 steps"=w1353, "Y2 data in"=w1345, "X data in"=w1359, "Y1 data in"=w1347, "Y3 data in"=w1343, "error in (no error)"=w1341) -> ("Array of clusters"=w1357:cluster{"Y data in":dbl[], "X data in":dbl[]}[], "error out"=w1340:errorcluster)  [unwired: 1 in]
            n417 = call "4155C Split array.vi"("Number of VAR2 steps"=w1353, "Y2 data in"=w1344, "X data in"=w1359, "Y1 data in"=w1346, "Y3 data in"=w1342, "error in (no error)"=w1340) -> ("Array of clusters"=w1358:cluster{"Y data in":dbl[], "X data in":dbl[]}[], "error out"=w1339:errorcluster)  [unwired: 1 in]
            n418 = call "4155C Split array.vi"("Number of VAR2 steps"=w1353, "Y2 data in"=w1351, "X data in"=w1359, "Y1 data in"=w1354, "Y3 data in"=w1349, "error in (no error)"=w1339) -> ("Array of clusters"=w1396:cluster{"Y data in":dbl[], "X data in":dbl[]}[], "error out"=w1338:errorcluster)  [unwired: 1 in]
            n419 = call "4155C Split array.vi"("Number of VAR2 steps"=w1353, "Y2 data in"=w1350, "X data in"=w1359, "Y1 data in"=w1352, "Y3 data in"=w1348, "error in (no error)"=w1338) -> ("Array of clusters"=w1395:cluster{"Y data in":dbl[], "X data in":dbl[]}[], "error out"=w1337:errorcluster)  [unwired: 1 in]
            n420 = call "4155C Config Chart Colours.vi"("Numeric"=w1353, "XY Graph 2"=w1388) -> ()  [unwired: 6 in]
            n421 = call "4155C Config Chart Colours.vi"("Numeric"=w1353, "XY Graph 2"=w1387) -> ()  [unwired: 6 in]
            n422 = call "4155C Config Chart Colours.vi"("Numeric"=w1353, "XY Graph 2"=w1356) -> ()  [unwired: 6 in]
            n423 = call "4155C Config Chart Colours.vi"("Numeric"=w1353, "XY Graph 2"=w1355) -> ()  [unwired: 6 in]
            n424 = call "4155C Config Chart Colours.vi"("Numeric"=w1353, "XY Graph 2"=w1397) -> ()  [unwired: 6 in]
            n425 = local write "Imax vs time"(w1396) -> ()
            n426 = local write "Imin vs time"(w1395) -> ()
            n427 = local write "Ion vs time"(w1357) -> ()
            n428 = local write "Ioff vs time"(w1358) -> ()
          }
        }
        n429 = call "4155C Split array.vi"("Number of VAR2 steps"=w1200, "Y2 data in"=w1242, "X data in"=w1244, "Y1 data in"=w1243, "Y3 data in"=w1242, "error in (no error)"=w1210) -> ("Array of clusters"=w1245:cluster{"Y data in":dbl[], "X data in":dbl[]}[], "error out"=w1209:errorcluster)  [unwired: 1 in]
        n430 = call "4155C Split array.vi"("Number of VAR2 steps"=w1200, "Y2 data in"=w1198, "X data in"=w1244, "Y1 data in"=w1198, "Y3 data in"=w1197, "error in (no error)"=w1209) -> ("Array of clusters"=w1247:cluster{"Y data in":dbl[], "X data in":dbl[]}[], "error out"=w1246:errorcluster)  [unwired: 1 in]
        n431 = local write "I vs Vd"(w1247) -> ()
        n432 = local write "Vp vs Vg (FPP)"(w1245) -> ()
        n433 = Open/Create/Replace File(file path (use dialog)=w1305, error in=w1246, operation (0:open)=w1265) -> (refnum out=w1315:refnum<file>, error out=w1316:errorcluster)  [unwired: 3 in, 1 out]
        n434 = call "4155C Make Big 2d array FPP.vi"("1D Var1"=w1244, "1d ID"=w1198, "1d Vp2"=w1243, "1d IG"=w1197, "1d Vp1"=w1242, "VAR2 START"=w1266, "Number of VAR2 steps"=w1200, "VAR2 STEP"=w1268, "VAR1 Name"="Vd", "Decimal places in header"=i8 1, "VAR2 Name"="Vg") -> ("Header array"=w1311:string[], "Data array"=w1312:dbl[][])  [unwired: 15 in]
        n435 = call "4155C Write array to file.vi"("Byte Stream File Refnum"=w1315, "Header"=w1311, "Data Array"=w1312, "error in (no error)"=w1316) -> ("dup refnum"=w1313:refnum<file>, "error out"=w1314:errorcluster)  [unwired: 1 in]
        n436 = call "4155C Config Chart Colours.vi"("Numeric"=w1200, "XY Graph 2"=w1241) -> ()  [unwired: 6 in]
        n437 = call "4155C Config Chart Colours.vi"("Numeric"=w1200, "XY Graph 2"=w1240) -> ()  [unwired: 6 in]
        n438 = Close File(refnum=w1313, error in=w1314) -> (error out=w1300:errorcluster)  [unwired: 1 out]
      }
      frame "itime" {
        n439 = Delete From Array(array=w1417, index=1) -> (deleted portion=w1416:string)  [unwired: 1 in, 1 out]
        n440 = Delete From Array(array=w1417, index=0 ("Index")) -> (deleted portion=w1451:string)  [unwired: 1 in, 1 out]
        n441 = Fract/Exp String To Number(string=w1416) -> (number=w1415:dbl)  [unwired: 3 in, 1 out]
        n442 = case shown="\"l\"" w1451 {
          tunnel: w1450 -> [w1456 w1458 w1462]
          tunnel: [w1455 w1457 w1461] -> w1443
          tunnel: w1415 -> [w1453 _ w1460]
          frame "s" {
            w1454 = u32 0 items=["short  ", "medium  ", "long  "] ("integration time 2")
            n443 = Bundle By Name(cluster=w1456, "integration time"=w1454, "Short/Long integration time"=w1453) -> (w1455:T5)
          }
          frame "m", Default {
            w1459 = u32 1 items=["short  ", "medium  ", "long  "] ("integration time 2")
            n444 = Bundle By Name(cluster=w1458, "integration time"=w1459) -> (w1457:T5)
          }
          frame "l" {
            w1463 = u32 2 items=["short  ", "medium  ", "long  "] ("integration time 2")
            n445 = Bundle By Name(cluster=w1462, "integration time"=w1463, "Short/Long integration time"=w1460) -> (w1461:T5)
          }
        }
      }
      frame "pulsed" {
        n446 = Delete From Array(array=w1506, index=0 ("Index")) -> (deleted portion=w1507:string, array with subset deleted=w1494:string[])  [unwired: 1 in]
        n447 = case shown="\"on\", Default" w1507 {
          tunnel: w1505 -> [w1517 w1520]
          tunnel: [w1516 w1519] -> w1498
          tunnel: w1494 -> [w1514 _]
          frame "on", Default {
            w1515 = u16 1 items=["Continuous", "Pulsed"] ("sweep method")
            n448 = Fract/Exp String To Number(string=w1514) -> (number=w1512:dbl[])  [unwired: 3 in, 1 out]
            n449 = Index Array(array=w1512, index #1=0 ("Index")) -> (element #1=w1511:dbl, element #2=w1510:dbl, element #3=w1509:dbl)  [unwired: 2 in]
            n450 = Bundle By Name(cluster=w1517, "sweep method"=w1515, "Pulse period"=w1511, "Base voltage"=w1510, "Pulse width"=w1509) -> (w1516:T5)
          }
          frame "off" {
            w1518 = u16 0 items=["Continuous", "Pulsed"] ("sweep method")
            n451 = Bundle By Name(cluster=w1520, "sweep method"=w1518) -> (w1519:T5)
          }
        }
      }
      frame "gaterangemode" {
        n452 = Delete From Array(array=w1561, index=0 ("Index")) -> (deleted portion=w1562:string)  [unwired: 1 in, 1 out]
        n453 = case shown="\"f\"" w1562 {
          tunnel: [w1564 w1565 w1566] -> w1551
          frame "a", Default {
            w1564 = u16 0 items=["Auto", "Limited", "Fixed"] ("Gate Range\nmode 2")
          }
          frame "f" {
            w1565 = u16 2 items=["Auto", "Limited", "Fixed"] ("Gate Range\nmode 2")
          }
          frame "l" {
            w1566 = u16 1 items=["Auto", "Limited", "Fixed"] ("Gate Range\nmode 2")
          }
        }
      }
      frame "gaterange" {
        (unwired) u8 11 items=["10fA  ", "100fA  ", "1nA  ", "10nA", "100nA", "1uA", "10uA", "100uA", "1mA", "10mA", "100mA", "1A"] ("Gate Range 2")
        n454 = Delete From Array(array=w1614, index=0 ("Index")) -> (deleted portion=w1604:string)  [unwired: 1 in, 1 out]
        n455 = Scan Value(string=w1604, format string="") -> (value=w1602:dbl)  [unwired: 1 in, 1 out]
        n456 = Logarithm Base 10(1:w1602) -> (0:w1601:dbl)
        n457 = Round To Nearest(number=w1601) -> (nearest integer value=w1600:dbl)
        n458 = Add(x=w1600, y=11.0) -> (x+y=w1598:dbl)
        n459 = To Unsigned Byte Integer(number=w1598) -> (unsigned 8bit integer=w1597:u8)
      }
      frame "drainrange" {
        (unwired) u8 11 items=["10fA  ", "100fA  ", "1nA  ", "10nA", "100nA", "1uA", "10uA", "100uA", "1mA", "10mA", "100mA", "1A"] ("Gate Range 2")
        n460 = Delete From Array(array=w1663, index=0 ("Index")) -> (deleted portion=w1654:string)  [unwired: 1 in, 1 out]
        n461 = Scan Value(string=w1654, format string="") -> (value=w1652:dbl)  [unwired: 1 in, 1 out]
        n462 = Logarithm Base 10(1:w1652) -> (0:w1651:dbl)
        n463 = Round To Nearest(number=w1651) -> (nearest integer value=w1650:dbl)
        n464 = Add(x=w1650, y=11.0) -> (x+y=w1648:dbl)
        n465 = To Unsigned Byte Integer(number=w1648) -> (unsigned 8bit integer=w1647:u8)
      }
      frame "drainrangemode" {
        n466 = Delete From Array(array=w1705, index=0 ("Index")) -> (deleted portion=w1706:string)  [unwired: 1 in, 1 out]
        n467 = case shown="\"f\"" w1706 {
          tunnel: [w1708 w1709 w1710] -> w1695
          frame "a", Default {
            w1708 = u16 0 items=["Auto", "Limited", "Fixed"] ("Gate Range\nmode 2")
          }
          frame "f" {
            w1709 = u16 2 items=["Auto", "Limited", "Fixed"] ("Gate Range\nmode 2")
          }
          frame "l" {
            w1710 = u16 1 items=["Auto", "Limited", "Fixed"] ("Gate Range\nmode 2")
          }
        }
      }
      frame "Error", Default {
      }
      frame "logfile" {
        n468 = Number To Decimal String(number=w1781) -> (decimal integer string=w1816:string)  [unwired: 1 in]
        n469 = Concatenate Strings(w1815, "logfile" ("Substring"), w1816, w1779, ".txt" ("Substring")) -> (w1813:string)
        n470 = String To Path(string=w1813) -> (path=w1786:path)
        n471 = Unbundle(w1812) -> ("integration time"=w1811:u32, "Short/Long integration time"=w1810:dbl, "hold time (sec)"=w1809:dbl, "delay time (sec)"=w1808:dbl, "Step Time (0 disables)"=w1807:dbl, "sweep method"=w1806:u16, "Pulse period"=w1805:dbl, "Base voltage"=w1804:dbl, "Pulse width"=w1803:dbl)
        n472 = Build Array(w1811, w1810, w1809, w1808, w1807, w1806, w1805, w1804, w1803, w1797, w1798, w1799, w1800, w1801, w1802) -> (w1790:dbl[])
        n473 = Insert Into Array(array=dbl[][] [] ("Input Array"), new element=w1790) -> (w1789:dbl[][])  [unwired: 2 in]
        n474 = call <vilib>:"compatOverwrite.vi"("overwrite (F)"=TRUE) -> ("overwrite?"=w1784:T8)
        n475 = Open/Create/Replace File(file path (use dialog)=w1786, error in=w1788, operation (0:open)=w1784) -> (refnum out=w1794:refnum<file>, error out=w1793:errorcluster)  [unwired: 3 in, 1 out]
        n476 = call "4155C Write array to file.vi"("Byte Stream File Refnum"=w1794, "Header"=string[] ["Int Time", "Short/Long Itime", "Hold time", "Delay time", "Step time", "Sweep method", "Pulse period", "Base Voltage", "Pulse width", "Drain compliance", "Gate compliance", "Gate range mode", "Gate range", "S/D range mode", "S/D range"], "Data Array"=w1789, "error in (no error)"=w1793) -> ("dup refnum"=w1796:refnum<file>, "error out"=w1795:errorcluster)  [unwired: 1 in]
        n477 = Close File(refnum=w1796, error in=w1795) -> (error out=w1787:errorcluster)  [unwired: 1 out]
      }
      frame "sample" {
        w1858 = 1
        # "The suffix is Vg_Vd_Time."
        # "Add a time offset (elapsed time) to the time axis."
        # "Adjusts graph colors."
        n478 = Number To Decimal String(number=w1892) -> (decimal integer string=w1930:string)  [unwired: 1 in]
        n479 = local read "Sample - Drain"() -> (w1826:u32)
        n480 = Fract/Exp String To Number(string=w1928) -> (number=w1896:dbl[])  [unwired: 3 in, 1 out]
        n481 = Index Array(array=w1896, index=0 ("Index")) -> (element=w1850:dbl)
        n482 = Index Array(array=w1896, index=2 ("Index")) -> (element=w1924:dbl)
        n483 = Index Array(array=w1896, index=3 ("Index")) -> (element=w1847:dbl)
        n484 = Index Array(array=w1896, index=4 ("Index")) -> (element=w1895:dbl)
        n485 = Index Array(array=w1896, index=1 ("Index")) -> (element=w1852:dbl)
        n486 = local read "Sample - Probe 4"() -> (w1829:u32)
        n487 = local read "Sample - Source/Common"() -> (w1827:u32)
        n488 = local read "Time Units"() -> (w1822:u16)
        n489 = local read "Sample - Gate"() -> (w1828:u32)
        n490 = call "4155C Config Sampling Measurements v3.0.vi"("VISA session"=w1933, "Num Points"=w1924, "Sample - Drain"=w1826, "Display on/off"=TRUE, "Gate Compliance"=w1911, "Sampling interval"=w1895, "Sample - Source/Common"=w1827, "Sample - Probe 4"=w1829, "Drain Compliance"=w1931, "Standby"=w1830, "error in (no error)"=w1932, "Timings"=w1903, "Sample - Gate"=w1828, "Sample time"=w1847) -> ("dup VISA resource name"=w1935:refnum<visa-resource-name>, "error out"=w1934:errorcluster)
        n491 = local read "Plot sample extrema vs time"() -> (w1860:bool)
        n492 = Number To Decimal String(number=w1852) -> (decimal integer string=w1853:string)  [unwired: 1 in]
        n493 = Number To Decimal String(number=w1850) -> (decimal integer string=w1849:string)  [unwired: 1 in]
        n494 = Number To Decimal String(number=w1847) -> (decimal integer string=w1846:string)  [unwired: 1 in]
        n495 = call "4155C Take Sample v3.0.vi"("VISA resource name in"=w1935, "Emergency Stop"=w1908, "Sample - Gate"=w1828, "Vg"=w1850, "Sample - Drain"=w1826, "Vd"=w1852, "error in (no error)"=w1934) -> ("Time"=w1823:dbl[], "VISA Resource Name out"=w1905:refnum<visa-resource-name>, "Ig"=w1840:dbl[], "Id"=w1841:dbl[], "Is"=w1842:dbl[], "error out"=w1868:errorcluster)  [unwired: 3 in]
        n496 = Insert Into Array(array=w1834, new element=w1841) -> (w1837:dbl[])  [unwired: 1 in]
        n497 = case shown="2" w1822 {
          tunnel: [w1938 w1939 w1942] -> w1825
          tunnel: w1823 -> [w1937 w1939 w1941]
          frame 2 {
            n498 = Divide(x=w1937, y=3600.0) -> (x/y=w1938:dbl[])
          }
          frame 0, Default {
          }
          frame 1 {
            n499 = Divide(x=w1941, y=60.0) -> (x/y=w1942:dbl[])
          }
        }
        n500 = Insert Into Array(array=w1833, new element=w1842) -> (w1839:dbl[])  [unwired: 1 in]
        n501 = Insert Into Array(array=w1835, new element=w1840) -> (w1838:dbl[])  [unwired: 1 in]
        n502 = Concatenate Strings(w1853, "_" ("Substring"), w1849, "_" ("Substring"), w1846, ".txt" ("Substring")) -> (w1844:string)
        n503 = Concatenate Strings(w1855, w1854, w1930, w1890, "_S_" ("Substring"), w1844) -> (w1929:string)
        n504 = String To Path(string=w1929) -> (path=w1914:path)
        n505 = Add(x=w1825, y=w1824) -> (x+y=w1843:dbl[])
        n506 = Insert Into Array(array=w1832, new element=w1843) -> (w1836:dbl[])  [unwired: 1 in]
        n507 = case shown="True" w1860 {
          tunnel: w1843 -> [_ w1945]
          tunnel: [w1943 w1946] -> w1857
          tunnel: w1861 -> [w1943 w1944]
          frame False {
          }
          frame True {
            n508 = Insert Into Array(array=w1944, new element=w1945) -> (w1946:i32[])  [unwired: 1 in]
          }
        }
        n509 = case shown="True" "Plot sample extrema vs time" {
          tunnel: w1842 -> [_ w1975]
          tunnel: w1841 -> [_ w1976]
          tunnel: w1840 -> [_ w1977]
          tunnel: [w1953 w1963] -> w1831
          tunnel: w1868 -> [w1953 w1968]
          tunnel: w1874 -> [w1952 w1980]
          tunnel: w1873 -> [w1951 w1979]
          tunnel: w1872 -> [w1950 w1981]
          tunnel: w1871 -> [w1949 w1978]
          tunnel: w1870 -> [w1948 w1983]
          tunnel: w1869 -> [w1947 w1982]
          tunnel: [w1952 w1967] -> w1867
          tunnel: [w1951 w1961] -> w1866
          tunnel: [w1950 w1965] -> w1865
          tunnel: [w1949 w1960] -> w1864
          tunnel: [w1948 w1966] -> w1863
          tunnel: [w1947 w1959] -> w1862
          tunnel: w1857 -> [_ w1957]
          frame False {
          }
          frame True {
            w1962 = 1
            # "Number of VAR2 steps is 1."
            # "abs(Ig)"
            # "abs(Is)"
            # "abs(Id)"
            # "Adjusts graph colors."
            n510 = Absolute Value(x=w1977) -> (abs(x)=w1954:dbl[])
            n511 = Absolute Value(x=w1976) -> (abs(x)=w1955:dbl[])
            n512 = Absolute Value(x=w1975) -> (abs(x)=w1956:dbl[])
            n513 = Array Max & Min(array=w1956) -> (max value=w1974:dbl, min value=w1971:dbl)  [unwired: 2 out]
            n514 = Array Max & Min(array=w1955) -> (max value=w1973:dbl, min value=w1970:dbl)  [unwired: 2 out]
            n515 = Array Max & Min(array=w1954) -> (max value=w1972:dbl, min value=w1969:dbl)  [unwired: 2 out]
            n516 = local write "Id max"(w1973) -> ()
            n517 = local write "Id min"(w1970) -> ()
            n518 = local write "Ig max"(w1972) -> ()
            n519 = local write "Ig min"(w1969) -> ()
            n520 = Insert Into Array(array=w1983, new element=w1954) -> (w1966:dbl[])  [unwired: 1 in]
            n521 = Insert Into Array(array=w1982, new element=w1954) -> (w1959:dbl[])  [unwired: 1 in]
            n522 = local write "Is max"(w1974) -> ()
            n523 = local write "Is min"(w1971) -> ()
            n524 = Insert Into Array(array=w1981, new element=w1955) -> (w1965:dbl[])  [unwired: 1 in]
            n525 = Insert Into Array(array=w1978, new element=w1955) -> (w1960:dbl[])  [unwired: 1 in]
            n526 = Insert Into Array(array=w1980, new element=w1956) -> (w1967:dbl[])  [unwired: 1 in]
            n527 = Insert Into Array(array=w1979, new element=w1956) -> (w1961:dbl[])  [unwired: 1 in]
            n528 = control-ref of="Imax vs time"() -> (w1984:refnum<vi>)
            n529 = call "4155C Config Chart Colours.vi"("Numeric"=w1962, "XY Graph 2"=w1984) -> ()  [unwired: 6 in]
            n530 = call "4155C Split array.vi"("Number of VAR2 steps"=w1962, "Y2 data in"=w1965, "X data in"=w1957, "Y1 data in"=w1967, "Y3 data in"=w1966, "error in (no error)"=w1968) -> ("Array of clusters"=w1985:cluster{"Y data in":dbl[], "X data in":dbl[]}[], "error out"=w1964:errorcluster)  [unwired: 1 in]
            n531 = call "4155C Split array.vi"("Number of VAR2 steps"=w1962, "Y2 data in"=w1960, "X data in"=w1957, "Y1 data in"=w1961, "Y3 data in"=w1959, "error in (no error)"=w1964) -> ("Array of clusters"=w1958:cluster{"Y data in":dbl[], "X data in":dbl[]}[], "error out"=w1963:errorcluster)  [unwired: 1 in]
            n532 = local write "Imax vs time"(w1985) -> ()
            n533 = local write "Imin vs time"(w1958) -> ()
          }
        }
        n534 = control-ref of="I vs time (Bias Stress)"() -> (w1856:refnum<vi>)
        n535 = call "4155C Split array.vi"("Number of VAR2 steps"=w1858, "Y2 data in"=w1837, "X data in"=w1836, "Y1 data in"=w1839, "Y3 data in"=w1838) -> ("Array of clusters"=w1859:cluster{"Y data in":dbl[], "X data in":dbl[]}[])  [unwired: 2 in, 1 out]
        n536 = local write "I vs time (Bias Stress)"(w1859) -> ()
        n537 = call "4155C Config Chart Colours.vi"("Numeric"=w1858, "XY Graph 2"=w1856) -> ()  [unwired: 6 in]
        n538 = Insert Into Array(array=dbl[][] [] ("Input Array"), new element=w1843) -> (w1918:dbl[][])  [unwired: 2 in]
        n539 = Insert Into Array(array=w1918, new element=w1840) -> (w1917:dbl[][])  [unwired: 2 in]
        n540 = VISA Write(VISA resource name=w1905, write buffer=":DISP ON" ("write buffer (\"\")"), error in (no error)=w1831) -> (VISA resource name out=w1904:refnum<visa-resource-name>, error out=w1906:errorcluster)  [unwired: 1 out]
        n541 = Insert Into Array(array=w1917, new element=w1841) -> (w1916:dbl[][])  [unwired: 2 in]
        n542 = Insert Into Array(array=w1916, new element=w1842) -> (w1910:dbl[][])  [unwired: 2 in]
        n543 = call <vilib>:"compatOverwrite.vi"("overwrite (F)"=TRUE) -> ("overwrite?"=w1893:T8)
        n544 = Open/Create/Replace File(file path (use dialog)=w1914, error in=w1906, operation (0:open)=w1893) -> (refnum out=w1921:refnum<file>, error out=w1920:errorcluster)  [unwired: 3 in, 1 out]
        n545 = Transpose 2D Array(2D array=w1910) -> (transposed array=w1909:dbl[][])
        n546 = call "4155C Write array to file.vi"("Byte Stream File Refnum"=w1921, "Header"=string[] ["Time /Units", "Ig /A", "Id /A", "Is /A"], "Data Array"=w1909, "error in (no error)"=w1920) -> ("dup refnum"=w1923:refnum<file>, "error out"=w1922:errorcluster)  [unwired: 1 in]
        n547 = Close File(refnum=w1923, error in=w1922) -> (error out=w1912:errorcluster)  [unwired: 1 out]
      }
      frame "samplei" {
        w1998 = 1
        # "Adjusts graph colors."
        # "Add a time offset (elapsed time) to the time axis."
        n548 = Number To Decimal String(number=w2039) -> (decimal integer string=w2087:string)  [unwired: 1 in]
        n549 = local read "Sample I - Probe 4 (Disabled)"() -> (w2013:u32)
        n550 = local read "Sample I - Source/Common"() -> (w2010:u32)
        n551 = Concatenate Strings(w2068, "-samplei-" ("Substring"), w2087, w2038, ".txt" ("Substring")) -> (w2085:string)
        n552 = Fract/Exp String To Number(string=w2084) -> (number=w2053:dbl[])  [unwired: 3 in, 1 out]
        n553 = String To Path(string=w2085) -> (path=w2071:path)
        n554 = Index Array(array=w2053, index=4 ("Index")) -> (element=w2047:dbl)
        n555 = Index Array(array=w2053, index=3 ("Index")) -> (element=w2048:dbl)
        n556 = Index Array(array=w2053, index=1 ("Index")) -> (element=w2050:dbl)
        n557 = Index Array(array=w2053, index=0 ("Index")) -> (element=w2051:dbl)
        n558 = local read "Sample I - Drain/Gate"() -> (w2012:u32)
        n559 = Index Array(array=w2053, index=2 ("Index")) -> (element=w2049:dbl)
        n560 = local read "Plot sample extrema vs time"() -> (w2007:bool)
        n561 = local read "Time Units"() -> (w2004:u16)
        n562 = local read "Sample I - Probe 3 (Disabled)"() -> (w2011:u32)
        n563 = call "4155C Config SamplingI Measurements v3.0.vi"("VISA session"=w2090, "Num Points"=w2050, "Sample I - Probe 3 (Disabled)"=w2011, "Display on/off"=TRUE, "Sample I - Source/Common"=w2010, "Sample I - Drain/Gate"=w2012, "Sampling interval"=w2048, "Standby"=w2014, "error in (no error)"=w2089, "Timings"=w2060, "Sample I - Probe 4 (Disabled)"=w2013, "Sample time"=w2049) -> ("dup VISA resource name"=w2092:refnum<visa-resource-name>, "error out"=w2091:errorcluster)  [unwired: 2 in]
        n564 = call "4155C Take SampleI v3.0.vi"("Sample I - Drain/Gate"=w2012, "Emergency Stop"=w2065, "error in (no error)"=w2091, "Idg 2"=w2051, "Vdg compliance 2"=w2047, "VISA resource name in"=w2092) -> ("error out"=w2063:errorcluster, "Idg"=w1990:dbl[], "Vdg"=w1991:dbl[], "VISA Resource Name out"=w2061:refnum<visa-resource-name>, "Is"=w1987:dbl[], "Time"=w2002:dbl[])
        n565 = case shown="2" w2004 {
          tunnel: [w2095 w2096 w2099] -> w2003
          tunnel: w2002 -> [w2094 w2096 w2098]
          frame 2 {
            n566 = Divide(x=w2094, y=3600.0) -> (x/y=w2095:dbl[])
          }
          frame 0, Default {
          }
          frame 1 {
            n567 = Divide(x=w2098, y=60.0) -> (x/y=w2099:dbl[])
          }
        }
        n568 = control-ref of="Vdg vs time (Bias Stress)"() -> (w1999:refnum<vi>)
        n569 = Add(x=w2003, y=w2001) -> (x+y=w1996:dbl[])
        n570 = Insert Into Array(array=w1997, new element=w1996) -> (w1995:dbl[])  [unwired: 1 in]
        n571 = case shown="True" w2007 {
          tunnel: w1996 -> [_ w2102]
          tunnel: [w2100 w2103] -> w2005
          tunnel: w2006 -> [w2100 w2101]
          frame False {
          }
          frame True {
            n572 = Insert Into Array(array=w2101, new element=w2102) -> (w2103:i32[])  [unwired: 1 in]
          }
        }
        n573 = Insert Into Array(array=w1992, new element=w1991) -> (w1986:dbl[])  [unwired: 1 in]
        n574 = call "4155C Split array.vi"("Number of VAR2 steps"=w1998, "X data in"=w1995, "Y1 data in"=w1986) -> ("Array of clusters"=w2000:cluster{"Y data in":dbl[], "X data in":dbl[]}[])  [unwired: 4 in, 1 out]
        n575 = local write "Vdg vs time (Bias Stress)"(w2000) -> ()
        n576 = Insert Into Array(array=dbl[][] [] ("Input Array"), new element=w1996) -> (w2075:dbl[][])  [unwired: 2 in]
        n577 = call "4155C Config Chart Colours.vi"("Numeric"=w1998, "XY Graph 2"=w1999) -> ()  [unwired: 6 in]
        n578 = Insert Into Array(array=w1994, new element=w1990) -> (w1993:dbl[])  [unwired: 1 in]
        n579 = Insert Into Array(array=w2075, new element=w1991) -> (w2074:dbl[][])  [unwired: 2 in]
        n580 = Insert Into Array(array=w1989, new element=w1987) -> (w1988:dbl[])  [unwired: 1 in]
        n581 = Insert Into Array(array=w2074, new element=w1990) -> (w2073:dbl[][])  [unwired: 2 in]
        n582 = VISA Write(VISA resource name=w2061, write buffer=":DISP ON" ("write buffer (\"\")"), error in (no error)=w2063) -> (VISA resource name out=w2046:refnum<visa-resource-name>, error out=w2062:errorcluster)  [unwired: 1 out]
        n583 = Insert Into Array(array=w2073, new element=w1987) -> (w2067:dbl[][])  [unwired: 2 in]
        n584 = call <vilib>:"compatOverwrite.vi"("overwrite (F)"=TRUE) -> ("overwrite?"=w2041:T8)
        n585 = Open/Create/Replace File(file path (use dialog)=w2071, error in=w2062, operation (0:open)=w2041) -> (refnum out=w2078:refnum<file>, error out=w2077:errorcluster)  [unwired: 3 in, 1 out]
        n586 = Transpose 2D Array(2D array=w2067) -> (transposed array=w2066:dbl[][])
        n587 = call "4155C Write array to file.vi"("Byte Stream File Refnum"=w2078, "Header"=string[] ["Time /s", "Vdg /V", "Idg /A", "Is /A"], "Data Array"=w2066, "error in (no error)"=w2077) -> ("dup refnum"=w2080:refnum<file>, "error out"=w2079:errorcluster)  [unwired: 1 in]
        n588 = Close File(refnum=w2080, error in=w2079) -> (error out=w2044:errorcluster)  [unwired: 1 out]
        n589 = VISA Write(VISA resource name=w2046, write buffer=";:PAGE:SCON:STAN OFF;:PAGE:CHAN:VSU2:DIS;" ("write buffer (\"\")"), error in (no error)=w2044) -> (VISA resource name out=w2042:refnum<visa-resource-name>, error out=w2043:errorcluster)  [unwired: 1 out]
      }
      frame "#" {
        n590 = VISA Write(VISA resource name=w2138, write buffer=":DISP ON" ("write buffer (\"\")"), error in (no error)=w2137) -> (VISA resource name out=w2136:refnum<visa-resource-name>, error out=w2135:errorcluster)  [unwired: 1 out]
      }
      frame "stressV" {
        n591 = Number To Decimal String(number=w2179) -> (decimal integer string=w2220:string)  [unwired: 1 in]
        n592 = Concatenate Strings(w2204, "-stressV-" ("Substring"), w2220, w2178, ".txt" ("Substring")) -> (w2218:string)
        n593 = Fract/Exp String To Number(string=w2217) -> (number=w2190:dbl[])  [unwired: 3 in, 1 out]
        n594 = local read "Stress V - Source/Common"() -> (w2153:u32)
        n595 = String To Path(string=w2218) -> (path=w2208:path)
        n596 = Index Array(array=w2190, index=3 ("Index")) -> (element=w2187:dbl)
        n597 = Index Array(array=w2190, index=1 ("Index")) -> (element=w2185:dbl)
        n598 = Index Array(array=w2190, index=0 ("Index")) -> (element=w2184:dbl)
        n599 = Index Array(array=w2190, index=4 ("Index")) -> (element=w2189:dbl)
        n600 = Index Array(array=w2190, index=2 ("Index")) -> (element=w2186:dbl)
        n601 = local read "Stress V - Drain"() -> (w2152:u32)
        n602 = local read "Stress V - Gate"() -> (w2151:u32)
        n603 = call "4155C Config V Stress v3.0.vi"("Display on/off"=TRUE, "Stress V - Gate"=w2151, "Stress V - Drain"=w2152, "Stress V - Source/Common"=w2153, "IG compliance"=w2186, "ID compliance"=w2187, "error in (no error)"=w2222, "VG"=w2184, "VD"=w2185, "VISA session"=w2223) -> ("error out"=w2224:errorcluster, "dup VISA resource name"=w2225:refnum<visa-resource-name>)
        n604 = call "4155C Apply Stress.vi"("error in (no error)"=w2224, "Duration"=w2189, "Emergency Stop"=w2203, "VISA resource name in"=w2225) -> ("error out"=w2201:errorcluster, "VISA Resource Name out"=w2199:refnum<visa-resource-name>)
        n605 = VISA Write(VISA resource name=w2199, write buffer=":DISP ON" ("write buffer (\"\")"), error in (no error)=w2201) -> (VISA resource name out=w2198:refnum<visa-resource-name>, error out=w2200:errorcluster)  [unwired: 1 out]
        n606 = call <vilib>:"compatOverwrite.vi"("overwrite (F)"=TRUE) -> ("overwrite?"=w2183:T8)
        n607 = Open/Create/Replace File(file path (use dialog)=w2208, error in=w2200, operation (0:open)=w2183) -> (refnum out=w2211:refnum<file>, error out=w2210:errorcluster)  [unwired: 3 in, 1 out]
        n608 = call "4155C Write array to file.vi"("Byte Stream File Refnum"=w2211, "Header"=string[] ["V stress completed successfully", ""], "error in (no error)"=w2210) -> ("dup refnum"=w2213:refnum<file>, "error out"=w2212:errorcluster)  [unwired: 2 in]
        n609 = Close File(refnum=w2213, error in=w2212) -> (error out=w2206:errorcluster)  [unwired: 1 out]
      }
      frame "stressI" {
        n610 = local read "Stress I - Source/Common"() -> (w2230:u32)
        n611 = Number To Decimal String(number=w2257) -> (decimal integer string=w2294:string)  [unwired: 1 in]
        n612 = Concatenate Strings(w2278, "-stressI-" ("Substring"), w2294, w2256, ".txt" ("Substring")) -> (w2292:string)
        n613 = Fract/Exp String To Number(string=w2291) -> (number=w2266:dbl[])  [unwired: 3 in, 1 out]
        n614 = Index Array(array=w2266, index=1 ("Index")) -> (element=w2262:dbl)
        n615 = Index Array(array=w2266, index=0 ("Index")) -> (element=w2263:dbl)
        n616 = Index Array(array=w2266, index=2 ("Index")) -> (element=w2264:dbl)
        n617 = String To Path(string=w2292) -> (path=w2282:path)
        n618 = local read "Stress I - Drain/Gate"() -> (w2231:u32)
        n619 = call "4155C Config I Stress v3.0.vi"("Stress I - Drain/Gate"=w2231, "Stress I - Source/Common"=w2230, "Display on/off"=TRUE, "error in (no error)"=w2296, "VDG compliance"=w2262, "IDG"=w2263, "VISA session"=w2297) -> ("error out"=w2298:errorcluster, "dup VISA resource name"=w2299:refnum<visa-resource-name>)  [unwired: 1 in]
        n620 = call "4155C Apply Stress.vi"("error in (no error)"=w2298, "Duration"=w2264, "Emergency Stop"=w2277, "VISA resource name in"=w2299) -> ("error out"=w2275:errorcluster, "VISA Resource Name out"=w2273:refnum<visa-resource-name>)
        n621 = VISA Write(VISA resource name=w2273, write buffer=":DISP ON" ("write buffer (\"\")"), error in (no error)=w2275) -> (VISA resource name out=w2272:refnum<visa-resource-name>, error out=w2274:errorcluster)  [unwired: 1 out]
        n622 = call <vilib>:"compatOverwrite.vi"("overwrite (F)"=TRUE) -> ("overwrite?"=w2261:T8)
        n623 = Open/Create/Replace File(file path (use dialog)=w2282, error in=w2274, operation (0:open)=w2261) -> (refnum out=w2285:refnum<file>, error out=w2284:errorcluster)  [unwired: 3 in, 1 out]
        n624 = call "4155C Write array to file.vi"("Byte Stream File Refnum"=w2285, "Header"=string[] ["I stress completed successfully", ""], "error in (no error)"=w2284) -> ("dup refnum"=w2287:refnum<file>, "error out"=w2286:errorcluster)  [unwired: 2 in]
        n625 = Close File(refnum=w2287, error in=w2286) -> (error out=w2280:errorcluster)  [unwired: 1 out]
      }
      frame "vsu2pulse" {
        n626 = Number To Decimal String(number=w2330) -> (decimal integer string=w2365:string)  [unwired: 1 in]
        n627 = Concatenate Strings(w2350, "-vsu2-" ("Substring"), w2365, w2329, ".txt" ("Substring")) -> (w2363:string)
        n628 = Fract/Exp String To Number(string=w2362) -> (number=w2338:dbl[])  [unwired: 3 in, 1 out]
        n629 = String To Path(string=w2363) -> (path=w2354:path)
        n630 = Index Array(array=w2338, index=1 ("Index")) -> (element=w2337:dbl)
        n631 = Index Array(array=w2338, index=0 ("Index")) -> (element=w2335:dbl)
        n632 = local read "VSU2 Stress - Source/Common"() -> (w2304:u32)
        n633 = call "4155C Config VSU2 Stress v3.0.vi"("VISA session"=w2368, "Display on/off"=TRUE, "VSU2"=w2335, "error in (no error)"=w2367, "VSU2 Stress - Source/Common"=w2304) -> ("dup VISA resource name"=w2370:refnum<visa-resource-name>, "error out"=w2369:errorcluster)
        n634 = call "4155C Apply Stress.vi"("error in (no error)"=w2369, "Duration"=w2337, "Emergency Stop"=w2349, "VISA resource name in"=w2370) -> ("error out"=w2347:errorcluster, "VISA Resource Name out"=w2345:refnum<visa-resource-name>)
        n635 = VISA Write(VISA resource name=w2345, write buffer=":DISP ON" ("write buffer (\"\")"), error in (no error)=w2347) -> (VISA resource name out=w2344:refnum<visa-resource-name>, error out=w2346:errorcluster)  [unwired: 1 out]
        n636 = call <vilib>:"compatOverwrite.vi"("overwrite (F)"=TRUE) -> ("overwrite?"=w2334:T8)
        n637 = Open/Create/Replace File(file path (use dialog)=w2354, error in=w2346, operation (0:open)=w2334) -> (refnum out=w2357:refnum<file>, error out=w2356:errorcluster)  [unwired: 3 in, 1 out]
        n638 = call "4155C Write array to file.vi"("Byte Stream File Refnum"=w2357, "Header"=string[] ["VSU2 pulse completed successfully", ""], "error in (no error)"=w2356) -> ("dup refnum"=w2359:refnum<file>, "error out"=w2358:errorcluster)  [unwired: 2 in]
        n639 = Close File(refnum=w2359, error in=w2358) -> (error out=w2352:errorcluster)  [unwired: 1 out]
      }
      frame "sample-fpp" {
        w2381 = 1
        w2446 = string[] ["Time /s", "Id VgVd /A", "Ig VgVd /A", "Vp1 VgVd /V", "Vp2 VgVd /V"] ("Header")
        w2450 = "%d" ("format string")
        # "Y1 = Y2 = ID\nY3 = IG"
        # "Y1 = Vp2\nY2 = Y3 = Vp1"
        # "Add a time offset (elapsed time) to the time axis."
        n640 = local read "Plot sample extrema vs time"() -> (w2390:bool)
        n641 = Number To Decimal String(number=w2438) -> (decimal integer string=w2492:string)  [unwired: 1 in]
        n642 = Fract/Exp String To Number(string=w2489) -> (number=w2477:dbl[])  [unwired: 3 in, 1 out]
        n643 = local read "Plot sample extrema vs time"() -> (w2393:bool)
        n644 = Concatenate Strings(w2483, "-samplefpp-" ("Substring"), w2492, w2437, ".txt" ("Substring")) -> (w2490:string)
        n645 = local read "FPP - Source"() -> (w2416:u32)
        n646 = local read "FPP - Drain"() -> (w2417:u32)
        n647 = local read "FPP - Gate"() -> (w2418:u32)
        n648 = local read "FPP - Probe 1"() -> (w2419:u32)
        n649 = control-ref of="I vs time (Bias Stress)"() -> (w2410:refnum<vi>)
        n650 = String To Path(string=w2490) -> (path=w2458:path)
        n651 = Index Array(array=w2477, index=0 ("Index")) -> (element=w2445:dbl)
        n652 = Index Array(array=w2477, index=1 ("Index")) -> (element=w2444:dbl)
        n653 = local read "Time Units"() -> (w2406:u16)
        n654 = Index Array(array=w2477, index=2 ("Index")) -> (element=w2485:dbl)
        n655 = Index Array(array=w2477, index=3 ("Index")) -> (element=w2475:dbl)
        n656 = Number To Decimal String(number=w2445) -> (decimal integer string=w2466:string)  [unwired: 1 in]
        n657 = local read "FPP - Probe 2"() -> (w2420:u32)
        n658 = call "4155C Config Sampling Measurements FPP v3.0.vi"("VISA session"=w2495, "Gate Compliance"=w2484, "FPP - Source"=w2416, "FPP - Drain"=w2417, "Drain Compliance"=w2493, "error in (no error)"=w2494, "Num Points"=w2485, "Timings"=w2482, "FPP - Gate"=w2418, "FPP - Probe 1"=w2419, "Vg"=w2445, "Vd"=w2444, "Display on/off"=TRUE, "Sample time"=w2475, "FPP - Probe 2"=w2420, "Standby"=w2421) -> ("dup VISA resource name"=w2460:refnum<visa-resource-name>, "error out"=w2459:errorcluster)  [unwired: 2 in]
        n659 = call "4155C Take Sample FPP.vi"("VISA resource name in"=w2460, "error in (no error)"=w2459, "Emergency Stop"=w2461) -> ("Time"=w2409:dbl[], "Vp1"=w2376:dbl[], "VISA Resource Name out"=w2442:refnum<visa-resource-name>, "Ig"=w2387:dbl[], "Id"=w2386:dbl[], "Vp2"=w2375:dbl[], "error out"=w2389:errorcluster)  [unwired: 10 in]
        n660 = Insert Into Array(array=w2414, new element=w2386) -> (w2373:dbl[])  [unwired: 1 in]
        n661 = Insert Into Array(array=w2415, new element=w2387) -> (w2412:dbl[])  [unwired: 1 in]
        n662 = Number To Decimal String(number=w2444) -> (decimal integer string=w2464:string)  [unwired: 1 in]
        n663 = call "4155C Config Chart Colours.vi"("Numeric"=w2381, "XY Graph 2"=w2410) -> ()  [unwired: 6 in]
        n664 = case shown="2" w2406 {
          tunnel: [w2535 w2536 w2539] -> w2408
          tunnel: w2409 -> [w2534 w2536 w2538]
          frame 2 {
            n665 = Divide(x=w2534, y=3600.0) -> (x/y=w2535:dbl[])
          }
          frame 0, Default {
          }
          frame 1 {
            n666 = Divide(x=w2538, y=60.0) -> (x/y=w2539:dbl[])
          }
        }
        n667 = Concatenate Strings("(Vg = " ("Substring"), w2466, "V, Vd = " ("Substring"), w2464, "V)" ("Substring")) -> (w2462:string)
        n668 = Add(x=w2408, y=w2407) -> (x+y=w2380:dbl[])
        n669 = case shown="True" w2390 {
          tunnel: w2380 -> [_ w2498]
          tunnel: [w2496 w2499] -> w2391
          tunnel: w2392 -> [w2496 w2497]
          frame False {
          }
          frame True {
            n670 = Insert Into Array(array=w2497, new element=w2498) -> (w2499:i32[])  [unwired: 1 in]
          }
        }
        n671 = case shown="True" w2393 {
          tunnel: w2386 -> [_ w2526]
          tunnel: w2387 -> [_ w2527]
          tunnel: [w2506 w2518] -> w2388
          tunnel: w2389 -> [w2506 w2521]
          tunnel: w2405 -> [w2505 w2511]
          tunnel: w2404 -> [w2504 w2510]
          tunnel: w2403 -> [w2503 w2529]
          tunnel: w2402 -> [w2502 w2528]
          tunnel: w2401 -> [w2501 w2530]
          tunnel: [w2505 w2511] -> w2399
          tunnel: [w2504 w2510] -> w2398
          tunnel: [w2503 w2507] -> w2397
          tunnel: [w2502 w2508] -> w2396
          tunnel: [w2501 w2520] -> w2395
          tunnel: [w2500 w2516] -> w2394
          tunnel: w2391 -> [_ w2514]
          tunnel: w2400 -> [w2500 w2509]
          frame False {
          }
          frame True {
            w2517 = 1
            # "Y1 = Y2 = ID\nY3 = IG"
            # "Number of VAR2 steps is 1."
            # "abs(Ig)"
            # "abs(Id)"
            # "Adjusts graph colors."
            n672 = Absolute Value(x=w2527) -> (abs(x)=w2512:dbl[])
            n673 = Absolute Value(x=w2526) -> (abs(x)=w2513:dbl[])
            n674 = Array Max & Min(array=w2513) -> (max value=w2525:dbl, min value=w2523:dbl)  [unwired: 2 out]
            n675 = Array Max & Min(array=w2512) -> (max value=w2524:dbl, min value=w2522:dbl)  [unwired: 2 out]
            n676 = Insert Into Array(array=w2530, new element=w2512) -> (w2520:dbl[])  [unwired: 1 in]
            n677 = local write "Id max"(w2525) -> ()
            n678 = local write "Id min"(w2523) -> ()
            n679 = local write "Ig max"(w2524) -> ()
            n680 = local write "Ig min"(w2522) -> ()
            n681 = Insert Into Array(array=w2509, new element=w2512) -> (w2516:dbl[])  [unwired: 1 in]
            n682 = Insert Into Array(array=w2529, new element=w2513) -> (w2507:dbl[])  [unwired: 1 in]
            n683 = Insert Into Array(array=w2528, new element=w2513) -> (w2508:dbl[])  [unwired: 1 in]
            n684 = control-ref of="Imax vs time"() -> (w2531:refnum<vi>)
            n685 = call "4155C Config Chart Colours.vi"("Numeric"=w2517, "XY Graph 2"=w2531) -> ()  [unwired: 6 in]
            n686 = call "4155C Split array.vi"("Number of VAR2 steps"=w2517, "Y2 data in"=w2507, "X data in"=w2514, "Y1 data in"=w2507, "Y3 data in"=w2520, "error in (no error)"=w2521) -> ("Array of clusters"=w2532:cluster{"Y data in":dbl[], "X data in":dbl[]}[], "error out"=w2519:errorcluster)  [unwired: 1 in]
            n687 = call "4155C Split array.vi"("Number of VAR2 steps"=w2517, "Y2 data in"=w2508, "X data in"=w2514, "Y1 data in"=w2508, "Y3 data in"=w2516, "error in (no error)"=w2519) -> ("Array of clusters"=w2515:cluster{"Y data in":dbl[], "X data in":dbl[]}[], "error out"=w2518:errorcluster)  [unwired: 1 in]
            n688 = local write "Imax vs time"(w2532) -> ()
            n689 = local write "Imin vs time"(w2515) -> ()
          }
        }
        n690 = Insert Into Array(array=w2413, new element=w2380) -> (w2382:dbl[])  [unwired: 1 in]
        n691 = call "4155C Split array.vi"("Number of VAR2 steps"=w2381, "Y2 data in"=w2373, "X data in"=w2382, "Y1 data in"=w2373, "Y3 data in"=w2412) -> ("Array of clusters"=w2411:cluster{"Y data in":dbl[], "X data in":dbl[]}[])  [unwired: 2 in, 1 out]
        n692 = local write "I vs time (Bias Stress)"(w2411) -> ()
        n693 = Insert Into Array(array=w2379, new element=w2376) -> (w2374:dbl[])  [unwired: 1 in]
        n694 = Insert Into Array(array=w2378, new element=w2375) -> (w2377:dbl[])  [unwired: 1 in]
        n695 = Insert Into Array(array=dbl[][] [] ("Input Array"), new element=w2380) -> (w2473:dbl[][])  [unwired: 2 in]
        n696 = control-ref of="Vp vs time (FPP Bias Stress)"() -> (w2383:refnum<vi>)
        n697 = Insert Into Array(array=w2473, new element=w2386) -> (w2472:dbl[][])  [unwired: 2 in]
        n698 = call <vilib>:"compatOverwrite.vi"("overwrite (F)"=TRUE) -> ("overwrite?"=w2440:T8)
        n699 = Open/Create/Replace File(file path (use dialog)=w2458, error in=w2388, operation (0:open)=w2440) -> (refnum out=w2455:refnum<file>, error out=w2456:errorcluster)  [unwired: 3 in, 1 out]
        n700 = Array To Spreadsheet String(array=w2446, 3:w2450) -> (spreadsheet string=w2452:string)  [unwired: 1 in]
        n701 = call "4155C Split array.vi"("Number of VAR2 steps"=w2381, "Y2 data in"=w2374, "X data in"=w2382, "Y1 data in"=w2377, "Y3 data in"=w2374) -> ("Array of clusters"=w2384:cluster{"Y data in":dbl[], "X data in":dbl[]}[])  [unwired: 2 in, 1 out]
        n702 = Insert Into Array(array=w2472, new element=w2387) -> (w2471:dbl[][])  [unwired: 2 in]
        n703 = Search and Replace String(replace all?=TRUE ("replace all? (F)"), input string=w2452, search string="VgVd", replace string=w2462) -> (result string=w2448:string)  [unwired: 4 in, 3 out]
        n704 = local write "Vp vs time (FPP Bias Stress)"(w2384) -> ()
        n705 = Insert Into Array(array=w2471, new element=w2376) -> (w2469:dbl[][])  [unwired: 2 in]
        n706 = call "4155C Config Chart Colours.vi"("Numeric"=w2381, "XY Graph 2"=w2383) -> ()  [unwired: 6 in]
        n707 = Spreadsheet String To Array(format string=w2450, spreadsheet string=w2448, array type (2D Dbl)=w2446) -> (array=w2447:string[])  [unwired: 1 in]
        n708 = Insert Into Array(array=w2469, new element=w2375) -> (w2443:dbl[][])  [unwired: 2 in]
        n709 = Transpose 2D Array(2D array=w2443) -> (transposed array=w2468:dbl[][])
        n710 = call "4155C Write array to file.vi"("Byte Stream File Refnum"=w2455, "Header"=w2447, "Data Array"=w2468, "error in (no error)"=w2456) -> ("dup refnum"=w2453:refnum<file>, "error out"=w2454:errorcluster)  [unwired: 1 in]
        n711 = Close File(refnum=w2453, error in=w2454) -> (error out=w2441:errorcluster)  [unwired: 1 out]
      }
      frame "resample-fpp" {
        w2550 = 1
        w2612 = string[] ["Time /s", "Id VgVd /A", "Ig VgVd /A", "Vp1 VgVd /V", "Vp2 VgVd /V"] ("Header")
        w2616 = "%d" ("format string")
        # "Y1 = Y2 = ID\nY3 = IG"
        # "Y1 = Vp2\nY2 = Y3 = Vp1"
        # "Add a time offset (elapsed time) to the time axis."
        n712 = Number To Decimal String(number=w2600) -> (decimal integer string=w2650:string)  [unwired: 1 in]
        n713 = local read "Plot sample extrema vs time"() -> (w2559:bool)
        n714 = Fract/Exp String To Number(string=w2647) -> (number=w2605:dbl[])  [unwired: 3 in, 1 out]
        n715 = Concatenate Strings(w2643, "-resamplefpp-" ("Substring"), w2650, w2601, ".txt" ("Substring")) -> (w2648:string)
        n716 = local read "Plot sample extrema vs time"() -> (w2562:bool)
        n717 = String To Path(string=w2648) -> (path=w2624:path)
        n718 = local read "Time Units"() -> (w2575:u16)
        n719 = Index Array(array=w2605, index=0 ("Index")) -> (element=w2611:dbl)
        n720 = Index Array(array=w2605, index=1 ("Index")) -> (element=w2610:dbl)
        n721 = Number To Decimal String(number=w2611) -> (decimal integer string=w2630:string)  [unwired: 1 in]
        n722 = call "4155C Take Sample FPP.vi"("VISA resource name in"=w2607, "error in (no error)"=w2606, "Emergency Stop"=w2625) -> ("Time"=w2576:dbl[], "Vp1"=w2545:dbl[], "VISA Resource Name out"=w2609:refnum<visa-resource-name>, "Ig"=w2556:dbl[], "Id"=w2555:dbl[], "Vp2"=w2544:dbl[], "error out"=w2558:errorcluster)  [unwired: 10 in]
        n723 = Insert Into Array(array=w2583, new element=w2555) -> (w2542:dbl[])  [unwired: 1 in]
        n724 = case shown="1" w2575 {
          tunnel: [w2691 w2692 w2695] -> w2578
          tunnel: w2576 -> [w2690 w2692 w2694]
          frame 2 {
            n725 = Divide(x=w2690, y=3600.0) -> (x/y=w2691:dbl[])
          }
          frame 0, Default {
          }
          frame 1 {
            n726 = Divide(x=w2694, y=60.0) -> (x/y=w2695:dbl[])
          }
        }
        n727 = Insert Into Array(array=w2584, new element=w2556) -> (w2581:dbl[])  [unwired: 1 in]
        n728 = Number To Decimal String(number=w2610) -> (decimal integer string=w2628:string)  [unwired: 1 in]
        n729 = Add(x=w2578, y=w2577) -> (x+y=w2549:dbl[])
        n730 = case shown="True" w2559 {
          tunnel: w2549 -> [_ w2654]
          tunnel: [w2652 w2655] -> w2560
          tunnel: w2561 -> [w2652 w2653]
          frame False {
          }
          frame True {
            n731 = Insert Into Array(array=w2653, new element=w2654) -> (w2655:i32[])  [unwired: 1 in]
          }
        }
        n732 = case shown="True" w2562 {
          tunnel: w2555 -> [_ w2681]
          tunnel: w2556 -> [_ w2682]
          tunnel: [w2662 w2673] -> w2557
          tunnel: w2558 -> [w2662 w2676]
          tunnel: w2574 -> [w2661 w2666]
          tunnel: w2572 -> [w2660 w2665]
          tunnel: w2570 -> [w2659 w2684]
          tunnel: w2569 -> [w2658 w2683]
          tunnel: w2568 -> [w2657 w2686]
          tunnel: w2567 -> [w2656 w2685]
          tunnel: [w2661 w2666] -> w2573
          tunnel: [w2660 w2665] -> w2571
          tunnel: [w2659 w2664] -> w2566
          tunnel: [w2658 w2663] -> w2565
          tunnel: [w2657 w2675] -> w2564
          tunnel: [w2656 w2671] -> w2563
          tunnel: w2560 -> [_ w2669]
          frame False {
          }
          frame True {
            w2672 = 1
            # "Y1 = Y2 = ID\nY3 = IG"
            # "Number of VAR2 steps is 1."
            # "abs(Ig)"
            # "abs(Id)"
            # "Adjusts graph colors."
            n733 = Absolute Value(x=w2682) -> (abs(x)=w2667:dbl[])
            n734 = Absolute Value(x=w2681) -> (abs(x)=w2668:dbl[])
            n735 = Array Max & Min(array=w2668) -> (max value=w2680:dbl, min value=w2678:dbl)  [unwired: 2 out]
            n736 = Array Max & Min(array=w2667) -> (max value=w2679:dbl, min value=w2677:dbl)  [unwired: 2 out]
            n737 = local write "Id max"(w2680) -> ()
            n738 = local write "Id min"(w2678) -> ()
            n739 = local write "Ig max"(w2679) -> ()
            n740 = local write "Ig min"(w2677) -> ()
            n741 = Insert Into Array(array=w2686, new element=w2667) -> (w2675:dbl[])  [unwired: 1 in]
            n742 = Insert Into Array(array=w2685, new element=w2667) -> (w2671:dbl[])  [unwired: 1 in]
            n743 = Insert Into Array(array=w2684, new element=w2668) -> (w2664:dbl[])  [unwired: 1 in]
            n744 = Insert Into Array(array=w2683, new element=w2668) -> (w2663:dbl[])  [unwired: 1 in]
            n745 = control-ref of="Imax vs time"() -> (w2687:refnum<vi>)
            n746 = call "4155C Config Chart Colours.vi"("Numeric"=w2672, "XY Graph 2"=w2687) -> ()  [unwired: 6 in]
            n747 = call "4155C Split array.vi"("Number of VAR2 steps"=w2672, "Y2 data in"=w2664, "X data in"=w2669, "Y1 data in"=w2664, "Y3 data in"=w2675, "error in (no error)"=w2676) -> ("Array of clusters"=w2688:cluster{"Y data in":dbl[], "X data in":dbl[]}[], "error out"=w2674:errorcluster)  [unwired: 1 in]
            n748 = call "4155C Split array.vi"("Number of VAR2 steps"=w2672, "Y2 data in"=w2663, "X data in"=w2669, "Y1 data in"=w2663, "Y3 data in"=w2671, "error in (no error)"=w2674) -> ("Array of clusters"=w2670:cluster{"Y data in":dbl[], "X data in":dbl[]}[], "error out"=w2673:errorcluster)  [unwired: 1 in]
            n749 = local write "Imax vs time"(w2688) -> ()
            n750 = local write "Imin vs time"(w2670) -> ()
          }
        }
        n751 = Insert Into Array(array=w2582, new element=w2549) -> (w2551:dbl[])  [unwired: 1 in]
        n752 = Concatenate Strings("(Vg = " ("Substring"), w2630, "V, Vd = " ("Substring"), w2628, "V)" ("Substring")) -> (w2626:string)
        n753 = control-ref of="I vs time (Bias Stress)"() -> (w2579:refnum<vi>)
        n754 = call "4155C Split array.vi"("Number of VAR2 steps"=w2550, "Y2 data in"=w2542, "X data in"=w2551, "Y1 data in"=w2542, "Y3 data in"=w2581) -> ("Array of clusters"=w2580:cluster{"Y data in":dbl[], "X data in":dbl[]}[])  [unwired: 2 in, 1 out]
        n755 = local write "I vs time (Bias Stress)"(w2580) -> ()
        n756 = call "4155C Config Chart Colours.vi"("Numeric"=w2550, "XY Graph 2"=w2579) -> ()  [unwired: 6 in]
        n757 = Insert Into Array(array=dbl[][] [] ("Input Array"), new element=w2549) -> (w2637:dbl[][])  [unwired: 2 in]
        n758 = Insert Into Array(array=w2548, new element=w2545) -> (w2543:dbl[])  [unwired: 1 in]
        n759 = Insert Into Array(array=w2637, new element=w2555) -> (w2636:dbl[][])  [unwired: 2 in]
        n760 = call <vilib>:"compatOverwrite.vi"("overwrite (F)"=TRUE) -> ("overwrite?"=w2603:T8)
        n761 = Open/Create/Replace File(file path (use dialog)=w2624, error in=w2557, operation (0:open)=w2603) -> (refnum out=w2621:refnum<file>, error out=w2622:errorcluster)  [unwired: 3 in, 1 out]
        n762 = Array To Spreadsheet String(array=w2612, 3:w2616) -> (spreadsheet string=w2618:string)  [unwired: 1 in]
        n763 = Insert Into Array(array=w2636, new element=w2556) -> (w2635:dbl[][])  [unwired: 2 in]
        n764 = Insert Into Array(array=w2547, new element=w2544) -> (w2546:dbl[])  [unwired: 1 in]
        n765 = Search and Replace String(replace all?=TRUE ("replace all? (F)"), input string=w2618, search string="VgVd", replace string=w2626) -> (result string=w2614:string)  [unwired: 4 in, 3 out]
        n766 = Insert Into Array(array=w2635, new element=w2545) -> (w2633:dbl[][])  [unwired: 2 in]
        n767 = Spreadsheet String To Array(format string=w2616, spreadsheet string=w2614, array type (2D Dbl)=w2612) -> (array=w2613:string[])  [unwired: 1 in]
        n768 = Insert Into Array(array=w2633, new element=w2544) -> (w2604:dbl[][])  [unwired: 2 in]
        n769 = control-ref of="Vp vs time (FPP Bias Stress)"() -> (w2552:refnum<vi>)
        n770 = Transpose 2D Array(2D array=w2604) -> (transposed array=w2632:dbl[][])
        n771 = call "4155C Write array to file.vi"("Byte Stream File Refnum"=w2621, "Header"=w2613, "Data Array"=w2632, "error in (no error)"=w2622) -> ("dup refnum"=w2619:refnum<file>, "error out"=w2620:errorcluster)  [unwired: 1 in]
        n772 = Close File(refnum=w2619, error in=w2620) -> (error out=w2608:errorcluster)  [unwired: 1 out]
        n773 = call "4155C Split array.vi"("Number of VAR2 steps"=w2550, "Y2 data in"=w2543, "X data in"=w2551, "Y1 data in"=w2546, "Y3 data in"=w2543) -> ("Array of clusters"=w2553:cluster{"Y data in":dbl[], "X data in":dbl[]}[])  [unwired: 2 in, 1 out]
        n774 = local write "Vp vs time (FPP Bias Stress)"(w2553) -> ()
        n775 = call "4155C Config Chart Colours.vi"("Numeric"=w2550, "XY Graph 2"=w2552) -> ()  [unwired: 6 in]
      }
      frame "serial" {
        n776 = local read "Termination char\n(0xA = '\\n' = LF)\n(0xD = '\\r' = CR)"() -> (w2731:u8)
        n777 = local read "Enable Termination\nChar (T)"() -> (w2732:bool)
        n778 = Index Array(array=w2739, index=0 ("Index")) -> (element=w2738:string)
        n779 = local read "parity"() -> (w2722:u16)
        n780 = local read "Delay before read (ms)"() -> (w2733:u32)
        n781 = local read "byte count"() -> (w2730:u32)
        n782 = local read "VISA resource name"() -> (w2726:refnum<visa-resource-name>)
        n783 = local read "baud rate"() -> (w2725:u32)
        n784 = local read "Serial End Mode for Reads"() -> (w2724:u16)
        n785 = local read "Timeout (ms)"() -> (w2729:u32)
        n786 = local read "data bits"() -> (w2723:u16)
        n787 = local read "stop bits"() -> (w2728:u16)
        n788 = local read "flow control"() -> (w2727:u16)
        n789 = call "Serial write and read v0.5.vi"("Delay before read (ms)"=w2733, "Termination char\n(0xA = '\\n' = LF)\n(0xD = '\\r' = CR)"=w2731, "Enable Termination\nChar (T)"=w2732, "parity"=w2722, "stop bits"=w2728, "string to write"=w2738, "flow control"=w2727, "byte count"=w2730, "Serial Settings:Serial End Mode for Reads"=w2724, "Timeout (ms)"=w2729, "error in (no error)"=w2744, "VISA resource name"=w2726, "baud rate"=w2725, "data bits"=w2723) -> ("Serial port output"=w2734:string, "error out"=w2743:errorcluster)
        n790 = Build Array (concatenate)(w2734, w2735) -> (w2736:string[])
      }
      frame "pump" {
        # "Time array for valve position"
        # "Time array for absolute plunger position"
        # "Valve position"
        # "Absolute plunger position"
        # "Remove \"_\""
        # "Check if pump is idle. Else halt."
        n791 = Index Array(array=w2816, index=0 ("Index")) -> (element=w2797:string)
        n792 = local read "Hard stop pump"() -> (w2756:bool)
        n793 = local read "Halt pump"() -> (w2757:bool)
        n794 = local read "Serial End Mode for Reads"() -> (w2804:u16)
        n795 = local read "flow control"() -> (w2807:u16)
        n796 = local read "stop bits"() -> (w2808:u16)
        n797 = local read "parity"() -> (w2802:u16)
        n798 = local read "Delay before read (ms)"() -> (w2813:u32)
        n799 = local read "byte count"() -> (w2810:u32)
        n800 = local read "VISA resource name"() -> (w2806:refnum<visa-resource-name>)
        n801 = local read "baud rate"() -> (w2805:u32)
        n802 = local read "Timeout (ms)"() -> (w2809:u32)
        n803 = local read "Termination char\n(0xA = '\\n' = LF)\n(0xD = '\\r' = CR)"() -> (w2811:u8)
        n804 = local read "Enable Termination\nChar (T)"() -> (w2812:bool)
        n805 = case shown="\"Internal failure\"" w2796 {
          tunnel: w2797 -> [w2852 _ w2854 w2855 w2856 w2857 _ _ w2860 w2861 _]
          tunnel: [w2852 "/1H" w2854 w2855 w2856 w2857 "/1H" "/1H" w2860 w2861 "/1H"] -> w2758
          frame "No error", Default {
          }
          frame "Initialization" {
          }
          frame "Invalid command" {
          }
          frame "Invalid operand" {
          }
          frame "Device not initialized" {
          }
          frame "Internal failure" {
          }
          frame "Plunger overload" {
          }
          frame "Valve overload" {
          }
          frame "Plunger move not allowed" {
          }
          frame "A/D converter failure" {
          }
          frame "Command overflow" {
          }
        }
        n806 = local read "data bits"() -> (w2803:u16)
        n807 = String Subset(string=w2792, offset (0)=1) -> (substring=w2790:string)  [unwired: 1 in]
        n808 = call "SPM Pump v0.7.vi"("Termination char\n(0xA = '\\n' = LF)\n(0xD = '\\r' = CR)"=w2811, "Enable Termination\nChar (T)"=w2812, "Timeout (ms)"=w2809, "Serial Settings:Serial End Mode for Reads"=w2804, "byte count"=w2810, "Delay before read (ms)"=w2813, "Time <input>"=w2795, "error in (no error)"=w2821, "Serial port input"=w2758, "VISA resource name"=w2806, "parity"=w2802, "baud rate"=w2805, "stop bits"=w2808, "data bits"=w2803, "flow control"=w2807, "Time units <input>"=w2790, "Hard stop pump"=w2756, "Halt pump"=w2757) -> ("Input command"=w2789:string, "Serial port data"=w2779:string[], "Pump status"=w2785:string, "Valve position"=w2787:i32, "Absolute plunger position"=w2798:i32, "Serial port"=w2794:string, "error out"=w2820:errorcluster)  [unwired: 2 in, 1 out]
        n809 = case shown="\"?6\"" w2789 {
          tunnel: [w2833 w2841 w2847] -> w2801
          tunnel: w2800 -> [w2833 w2840 w2847]
          tunnel: w2798 -> [_ w2839 _]
          tunnel: w2786 -> [w2832 w2838 w2848]
          tunnel: [w2832 w2838 w2850] -> w2788
          tunnel: w2787 -> [_ _ w2849]
          tunnel: w2784 -> [_ w2837 w2845]
          tunnel: w2783 -> [w2831 w2836 w2846]
          tunnel: [w2831 w2835 w2846] -> w2782
          tunnel: [w2830 w2834 w2844] -> w2781
          tunnel: w2780 -> [w2830 w2834 w2843]
          frame "Q", Default {
          }
          frame "?" {
            n810 = Build Array (concatenate)(w2840, w2839) -> (w2841:i32[])
            n811 = Build Array (concatenate)(w2836, w2837) -> (w2835:i32[])
            n812 = call "4155C Split array.vi"("X data in"=w2835, "Y1 data in"=w2841) -> ("Array of clusters"=w2842:cluster{"Y data in":dbl[], "X data in":dbl[]}[])  [unwired: 5 in, 1 out]
            n813 = local write "Absolute plunger position vs time"(w2842) -> ()
          }
          frame "?6" {
            n814 = Build Array (concatenate)(w2848, w2849) -> (w2850:i32[])
            n815 = Build Array (concatenate)(w2843, w2845) -> (w2844:i32[])
            n816 = call "4155C Split array.vi"("X data in"=w2844, "Y1 data in"=w2850) -> ("Array of clusters"=w2851:cluster{"Y data in":dbl[], "X data in":dbl[]}[])  [unwired: 5 in, 1 out]
            n817 = local write "Valve position vs time"(w2851) -> ()
          }
        }
        n818 = Build Array (concatenate)(w2777, w2779) -> (w2778:string[][])
        n819 = Build Array (concatenate)(w2793, w2794) -> (w2814:string[])
      }
      frame "filename" {
        n820 = Index Array(array=w2873, index=0 ("Index")) -> (element=w2872:string)
      }
    }
    "Probe 4 Indicator" <- w78
    "Timings Indicator" <- w77
    n821 = local read "Time Units"() -> (w111:u16)
    n822 = case shown="0" w111 {
      tunnel: ["Time (Seconds)" ("element") "Time (Minutes)" ("element") "Time (Hours)" ("element")] -> w79
      frame 0 {
      }
      frame 1, Default {
      }
      frame 2 {
      }
    }
    n823 = Build Array(w185, w118, w128, w127, w126, w125, w124, w123, w122, w121, w120, w119, w117) -> (w223:dbl[][])
    n824 = Transpose 2D Array(2D array=w223) -> (transposed array=w222:dbl[][])
    n825 = Concatenate Strings(w86, w85, "I-vs-time.txt" ("Suffix (Imax,Imin,Ion,Ioff)")) -> (w233:string)
    n826 = Build Array(w79, "Is max (A)" ("VAR2 Name"), "Is min (A)" ("VAR2 Name"), "Id max (A)" ("VAR2 Name"), "Id min (A)" ("VAR2 Name"), "Ig max (A)" ("VAR2 Name"), "Ig min (A)" ("VAR2 Name"), "Is on (A)" ("VAR2 Name"), "Is off (A)" ("VAR2 Name"), "Id on (A)" ("VAR2 Name"), "Id off (A)" ("VAR2 Name"), "Ig on (A)" ("VAR2 Name"), "Ig off (A)" ("VAR2 Name")) -> (w228:string[])
    n827 = Array To Spreadsheet String(array=w222, 3:"%e" ("format string")) -> (spreadsheet string=w226:string)  [unwired: 1 in]
    n828 = Array To Spreadsheet String(array=w228, 3:"" ("format string")) -> (spreadsheet string=w227:string)  [unwired: 1 in]
    n829 = String To Path(string=w233) -> (path=w232:path)
    n830 = Build Array(w227, w226) -> (w225:string[])
    n831 = Write to Text File(file (use dialog)=w232, text=w225, error in=w182) -> (refnum out=w234:refnum<file>, error out=w224:errorcluster)  [unwired: 1 in, 1 out]
    n832 = Close File(refnum=w234, error in=w224) -> (error out=w166:errorcluster)  [unwired: 1 out]
    n833 = Build Array(w163, w186) -> (w191:i32[][])
    n834 = Build Array(w79, "Absolute plunger position" ("VAR2 Name")) -> (w194:string[])
    n835 = Transpose 2D Array(2D array=w191) -> (transposed array=w184:i32[][])
    n836 = Array To Spreadsheet String(array=w194, 3:"" ("format string")) -> (spreadsheet string=w193:string)  [unwired: 1 in]
    n837 = Array To Spreadsheet String(array=w184, 3:"%e" ("format string")) -> (spreadsheet string=w190:string)  [unwired: 1 in]
    n838 = Build Array(w193, w190) -> (w196:string[])
    n839 = Concatenate Strings(w86, w85, "plunger.txt" ("Suffix (plunger)")) -> (w188:string)
    n840 = String To Path(string=w188) -> (path=w187:path)
    n841 = Write to Text File(file (use dialog)=w187, text=w196, error in=w166) -> (refnum out=w189:refnum<file>, error out=w198:errorcluster)  [unwired: 1 in, 1 out]
    n842 = Close File(refnum=w189, error in=w198) -> (error out=w165:errorcluster)  [unwired: 1 out]
    n843 = Concatenate Strings(w86, w85, "serial-port.txt" ("Suffix (serial port log)")) -> (w204:string)
    n844 = String To Path(string=w204) -> (path=w203:path)
    n845 = Build Array(w79, "Serial port input" ("VAR2 Name"), "Pump status" ("VAR2 Name"), "Serial port output: ") -> (w153:string[])
    n846 = Array To Spreadsheet String(array=w159, 3:"" ("format string")) -> (spreadsheet string=w150:string)  [unwired: 1 in]
    n847 = Array To Spreadsheet String(array=w153, 3:"" ("format string")) -> (spreadsheet string=w151:string)  [unwired: 1 in]
    n848 = Array To Spreadsheet String(array=w158, 3:"" ("format string")) -> (spreadsheet string=w209:string)  [unwired: 1 in]
    n849 = Build Array(w151, w150) -> (w152:string[])
    n850 = Write to Text File(file (use dialog)=w203, text=w152, error in=w165) -> (refnum out=w205:refnum<file>, error out=w206:errorcluster)  [unwired: 1 in, 1 out]
    n851 = local write "Serial port data"(w209) -> ()
    n852 = Close File(refnum=w205, error in=w206) -> (error out=w164:errorcluster)  [unwired: 1 out]
    n853 = Build Array(w162, w168) -> (w174:i32[][])
    n854 = Build Array(w79, "Valve port" ("VAR2 Name")) -> (w177:string[])
    n855 = Transpose 2D Array(2D array=w174) -> (transposed array=w169:i32[][])
    n856 = Array To Spreadsheet String(array=w177, 3:"" ("format string")) -> (spreadsheet string=w176:string)  [unwired: 1 in]
    n857 = Array To Spreadsheet String(array=w169, 3:"%e" ("format string")) -> (spreadsheet string=w173:string)  [unwired: 1 in]
    n858 = Build Array(w176, w173) -> (w179:string[])
    n859 = Concatenate Strings(w86, w85, "valve-port.txt" ("Suffix (valve)")) -> (w171:string)
    n860 = String To Path(string=w171) -> (path=w170:path)
    n861 = Write to Text File(file (use dialog)=w170, text=w179, error in=w164) -> (refnum out=w172:refnum<file>, error out=w181:errorcluster)  [unwired: 1 in, 1 out]
    n862 = Close File(refnum=w172, error in=w181) -> (error out=w87:errorcluster)  [unwired: 1 out]
    n863 = Build Array(w84, w83, w82, w81) -> (w96:dbl[][])
    n864 = Build Array(w79, "Is (A)" ("VAR2 Name"), "Id (A)" ("VAR2 Name"), "Ig (A)" ("VAR2 Name")) -> (w92:string[])
    n865 = Transpose 2D Array(2D array=w96) -> (transposed array=w95:dbl[][])
    n866 = Concatenate Strings(w86, w85, "sample.txt" ("Suffix (Imax,Imin,Ion,Ioff)")) -> (w102:string)
    n867 = Array To Spreadsheet String(array=w92, 3:"" ("format string")) -> (spreadsheet string=w91:string)  [unwired: 1 in]
    n868 = Array To Spreadsheet String(array=w95, 3:"%e" ("format string")) -> (spreadsheet string=w99:string)  [unwired: 1 in]
    n869 = local write "Hard stop pump"(w71) -> ()
    n870 = String To Path(string=w102) -> (path=w101:path)
    n871 = local write "Halt pump"(w71) -> ()
    n872 = Build Array(w91, w99) -> (w98:string[])
    n873 = Write to Text File(file (use dialog)=w101, text=w98, error in=w87) -> (refnum out=w103:refnum<file>, error out=w97:errorcluster)  [unwired: 1 in, 1 out]
    n874 = Close File(refnum=w103, error in=w97) -> (error out=w76:errorcluster)  [unwired: 1 out]
    "error out" <- w76
  }
  "Is max" <- w15
  "Id max" <- w15
  "Ig max" <- w15
  "Imax vs time" <- w2
  "I vs Vg" <- w2
  "Imin vs time" <- w2
  "I vs Vd" <- w2
  "Serial port data" <- "" ("Serial port data")
  "Absolute plunger position vs time" <- w2
  "Valve position vs time" <- cluster{"Y data in":dbl[], "X data in":dbl[]}[] [] ("Valve position vs time")
  "Is min" <- w14
  "Id min" <- w14
  "Ig min" <- w14
  "Ion vs time" <- w2
  "Ioff vs time" <- w2
  "Is on" <- w13
  "Id on" <- w13
  "Ig on" <- w13
  "Is off" <- w12
  "Id off" <- w12
  "Ig off" <- w12
  "I vs time (Bias Stress)" <- w2
  "Vp1" <- w3
  "Vp2" <- w3
  "Vp vs time (FPP Bias Stress)" <- w2
  "Vp vs Vg (FPP)" <- w2
  "Vdg vs time (Bias Stress)" <- w2
